vi "rio_veloster20.vi"() -> ()   [LabVIEW 2015]
uses:
  <vilib>/Analysis/Matrix/Datatypes/RealMatrix.ctl
  <vilib>/FPGAPlugInAG/cRIO-9113/niLvFpga_Open_cRIO-9113.vi
  <vilib>/rvi/interface/common/dynamic/niFpgaDynamicAddResources.vi
  <vilib>/FPGAPlugInAG/Dynamic/niLvFpga_Abort_Dynamic.vi
  <vilib>/FPGAPlugInAG/Dynamic/niLvFpga_Run_Dynamic.vi
  G_rio.vi
  <vilib>/Instr/_visa.llb/VISA Configure Serial Port (Instr).vi
  <vilib>/Utility/error.llb/Error Cluster From Error Code.vi
  <vilib>/rvi/errors/niLvFpgaAdjustHostInterfaceError.vi
  <vilib>/Analysis/Matrix/Numeric/Conversions/Array To Matrix - RA2.vi
  <vilib>/Analysis/Matrix/Numeric/Multiply/Multiply - RM,RM.vi
  <vilib>/Analysis/Matrix/Numeric/Add/Add - RM,RM.vi
  <vilib>/Analysis/baseanly.llb/Real Inverse Matrix.vi
  <vilib>/Analysis/Matrix/Numeric/Subtract/Subtract - RM,RM.vi
  <vilib>/Analysis/Matrix/Numeric/Conversions/Array To Matrix - RA.vi
  <vilib>/Analysis/Matrix/Numeric/Multiply/Multiply - R,RM.vi
  <vilib>/Analysis/Matrix/Numeric/Conversions/Matrix To Array - RM.vi
  <vilib>/rvi/interface/nirviOpenFPGA/nirviOpenFPGA.xnode
  FPGA Bitfiles/autonomous_FPGATarget2_fpga4_FZHAM7r+pqE.lvbitx
  fpga/fpga4.vi
  <vilib>/rvi/interface/nirviMethod/nirviMethod.xnode
  <vilib>/rvi/interface/nirviReadWriteControl/nirviReadWriteControl.xnode
  <vilib>/rvi/interface/Simulation/niFpgaSimulationCallBeginRW.vi
  <vilib>/rvi/errors/niLvFpgaMergeErrorWithErrorCode.vi
  NiFpgaLv.dll
  <vilib>/FPGAPlugInAG/Dynamic/niLvFpga_ReadFifo_Dynamic.vi
  <vilib>/Analysis/Matrix/NI_Matrix.lvlib
  <vilib>/Analysis/NI_AALBase.lvlib
panel:
  in  "map name":T1(ring)
  out "316H":u8[](array[numeric])
  out "FPGA":refnum<k20>
  out "Key":u8
  out "mdps torque":dbl(graph)
  out "battery voltage 2":dbl
  in  "steer limit":dbl=100.0
  in  "buzz":bool
  out "hcount":u64=1
  out "hbias":dbl
  out "vcount":u64=1
  out "vgain":dbl=1.0
  in  "heading gain":dbl=1.414
  in  "pos gain":dbl=4.0
  out "Pos_time 10":i32
  out "T PWM":u16
  out "B PWM":u16
  out "solenoid":bool
  out "brk enc":u8
  out "shift lever":dbl
  out "mobileye":u8[](array[numeric])
  out "timer":u32
  out "Mobileye_time 100":u32
  out "H_GPS":dbl
  out "pos":dbl[](array[numeric])
  out "pos error":dbl
  in  "GPS init":bool=TRUE
  in  "Gear Manual":i32(slide)=1 scale=-1.0..1.0
  out "map":i32=2
  out "P, R, D":i32
  out "heading error":dbl
  out "POS init":bool
  out "VS_CAN":dbl
  in  "brake":bool
  in  "Slide":dbl(slide)=1000.0 min=1000.0 max=2000.0 step=1500.0 scale=1000.0..2000.0
  out "novatel":refnum<visa-resource-name>
  in  "ublox":bool
  out "rest":u8[](array[numeric])
  out "GPS_novatel_time":u32
  out "GPS_time 100":u32
  out "Con_time 10":i32
  out "CAN_time 10":u32
  out "gps2":refnum<visa-resource-name>
  out "gps1":refnum<visa-resource-name>
  out "Heading":dbl
  out "ecef ref":dbl[](array[numeric])
  out "h_gps":dbl
  out "pos_gps":dbl[](array[numeric]) format="%#_19f"
  out "get heading":bool
  out "get position":bool
  out "dt":dbl
  out "rt":dbl
  out "CAN Comm Enabled":bool
  in  "SPAS Enable":bool=TRUE
  out "Ref steer":dbl=1.0
  in  "Steer input":bool=TRUE
  in  "Ref steer manual":dbl(knob) scale=-550.0..550.0
  out "Ref vel":dbl=1.0
  in  "Ref vel manual":dbl
  in  "Velocity input":bool
  out "Auto":bool
  out "Run":bool
  out "E - STOP":bool
  out "Throttle Enable":bool=TRUE
  # "P"
  # "R"
  # "D"
  # "Ref steer manual"
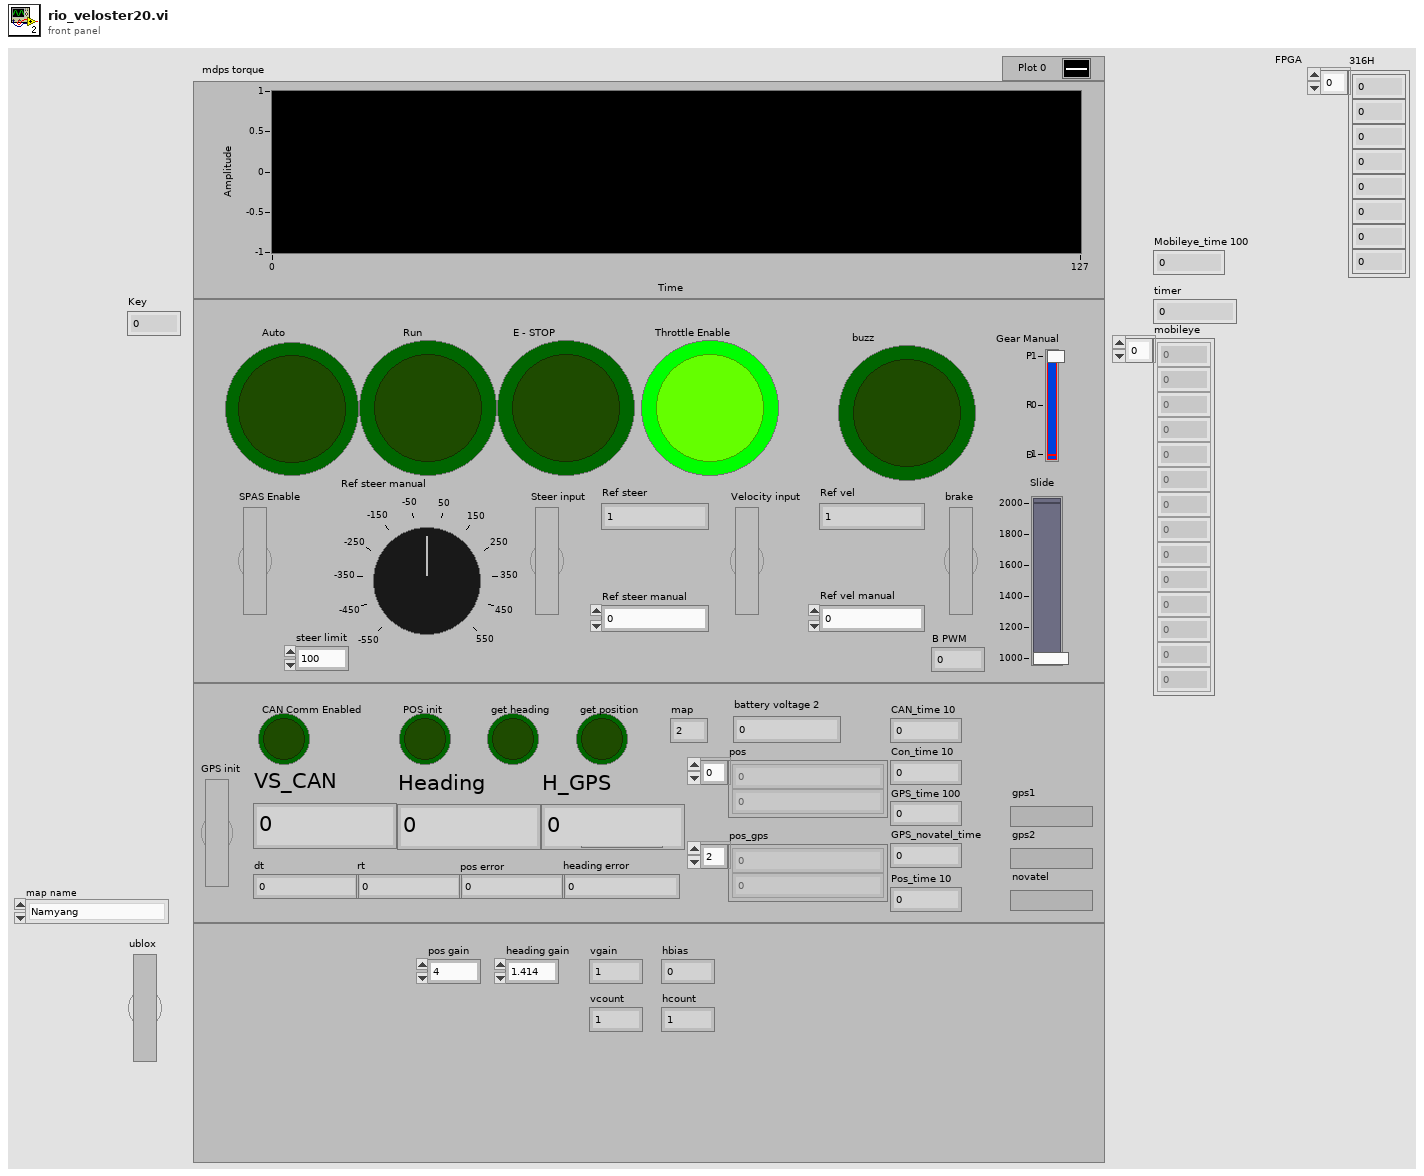
[diagram p1: front panel]
types:
  T1 = enum32{"Namyang", "Hyundai", "KAIST", "Ajou", "Munji", "Airforce", "Car", "KATRI", "Samsung", "Coex", "Gwangnaru", "Inje", "sinjin"}
  T2 = cluster{"timestamp high":u32, "timestamp low":u32, "identifier":u32, "type":enum8{"Data Frame", "Remote Frame", "(reserved)", "(reserved) ", "(reserved)  ", "(reserved)   ", "Bus Error", "Transceiver Fault"}, "info A":u8, "info B":u8, "data length":u8, "data":u8[]}
  T3 = cluster{"connection ID":refnum<k16>, "net address":u32, "port":u16}
  T4 = cluster{"hash":i64, "sys time":i64, "mobileye":u8[]}
  T5 = cluster{"hash":i64, "sys time":i64, "n":i32, "error":i32[]}
  T6 = cluster{"hash":i64, "sys time":i64, "time":dbl, "yaw_rate":dbl, "mdps torque":dbl, "mdps str_ang":dbl, "VS_CAN":dbl, "lat_accel":dbl, "mcp":dbl, "accel pedal value":dbl, "tps":dbl, "odometer":dbl, "battery voltage":dbl, "WHL_SPD_RR":dbl, "WHL_SPD_RL":dbl, "WHL_SPD_FR":dbl, "WHL_SPD_FL":dbl}
  T7 = cluster{"hash":i64, "sys time":i64, "ref_vel":dbl, "ref_steer":dbl, "alert":u8}
  T8 = cluster{"hash":i64, "sys time":i64, "ref_vel":dbl, "ref_steer":dbl}
  T9 = cluster{"hash":i64, "sys time":i64, "Auto":bool, "Run":bool, "Solenoid":bool, "T lim":bool, "brk_enc":u8, "B PWM":u16, "T PWM":u16, "ref_vel":dbl, "ref_bkr_enc":dbl, "ref_apv":dbl, "ref_steer":dbl}
  T10 = typedef "NI_Matrix.lvlib/RealMatrix.ctl" = dbl[][]
  T11 = cluster{"hash":i64, "sys time":i64, "time":dbl, "x":dbl, "y":dbl, "h":dbl, "numSV":i32, "postype":i32, "lag":i32, "hordev":dbl, "lat":dbl, "lon":dbl, "hgt":dbl, "map_idx":i32}
  T12 = cluster{"LCC[0]":dbl, "LCC[1]":dbl, "LCC[2]":dbl, "LCC[3]":dbl, "LCC[4]":dbl, "LCC[5]":dbl, "LCC[6]":dbl, "LCC[7]":dbl, "LCC[8]":dbl, "LCC[9]":dbl, "LCC[10]":dbl, "LCC[11]":dbl, "LCC[12]":dbl, "LCC[13]":dbl, "LCC[14]":dbl}
  T13 = cluster{"hash":i64, "sys time":i64, "time":dbl, "speed":dbl, "heading":dbl, "lat":dbl, "lon":dbl}
  T14 = cluster{"vel[0]":dbl, "vel[1]":dbl, "vel[2]":dbl, "vel[3]":dbl, "vel[4]":dbl, "vel[5]":dbl, "vel[6]":dbl}
  T15 = cluster{"output[0]":dbl, "output[1]":dbl, "output[2]":dbl, "output[3]":dbl, "output[4]":dbl, "output[5]":dbl, "output[6]":dbl, "output[7]":dbl, "output[8]":dbl, "output[9]":dbl, "output[10]":dbl, "output[11]":dbl, "output[12]":dbl, "output[13]":dbl, "output[14]":dbl}
  T16 = cluster{"output[0]":dbl, "output[1]":dbl, "output[2]":dbl, "output[3]":dbl, "output[4]":dbl, "output[5]":dbl, "output[6]":dbl}
  T17 = cluster{"hash":i64, "sys time":i64, "dt":dbl, "x":dbl, "y":dbl, "speed":dbl, "heading":dbl, "yaw_rate":dbl}
  T18 = cluster{"Real 2D Array[0]":dbl, "Real 2D Array[1]":dbl, "Real 2D Array[2]":dbl, "Real 2D Array[3]":dbl, "Real 2D Array[4]":dbl}
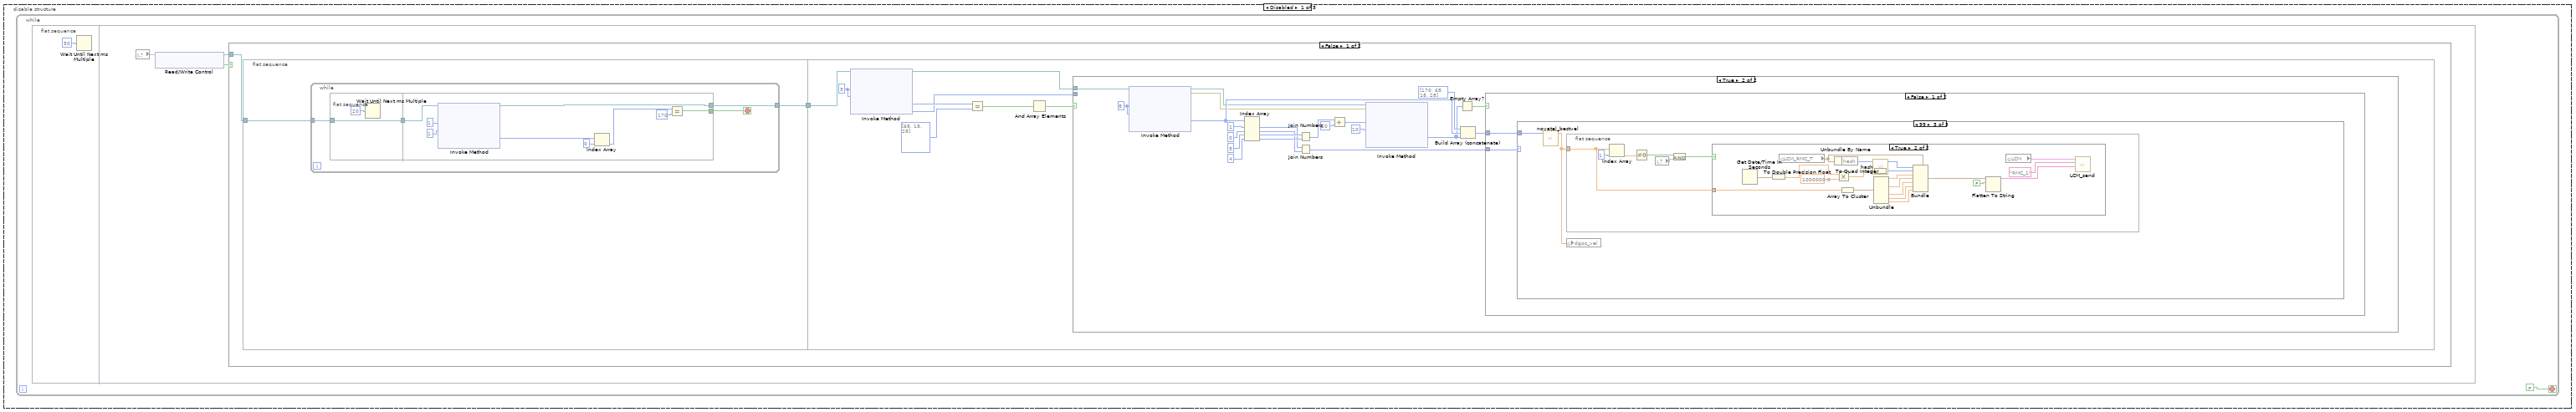
[diagram p2: hidden frame]
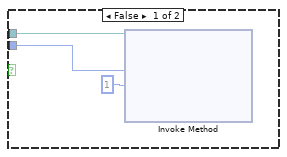
[diagram p3: hidden frame]
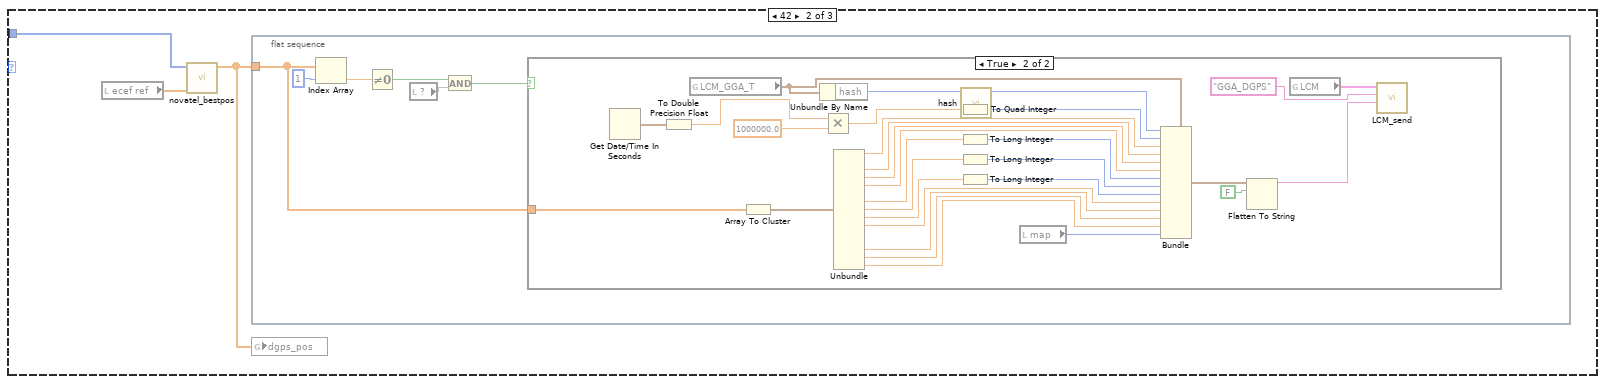
[diagram p5: hidden frame]
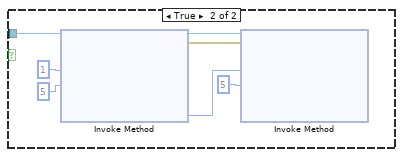
[diagram p9: hidden frame]
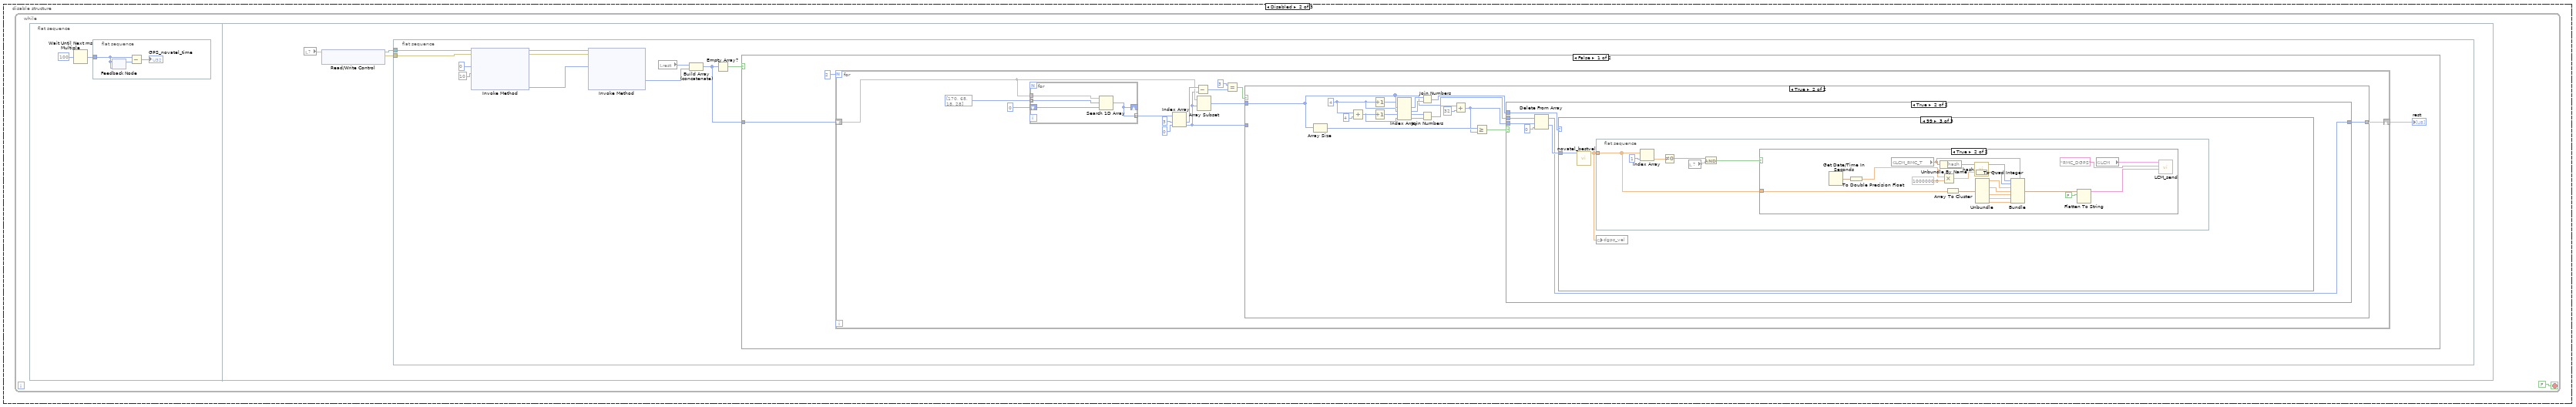
[diagram p10: hidden frame]
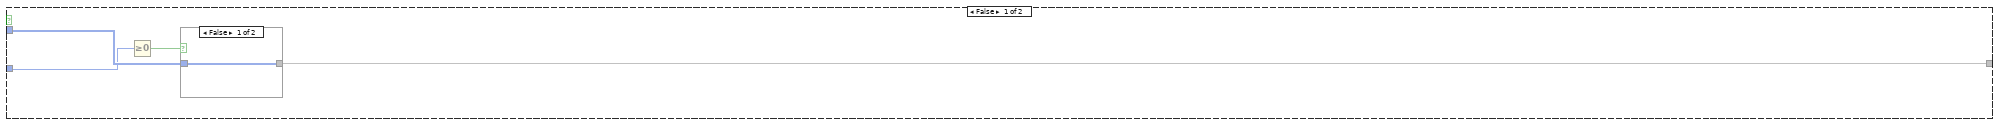
[diagram p11: hidden frame]
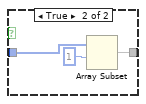
[diagram p12: hidden frame]
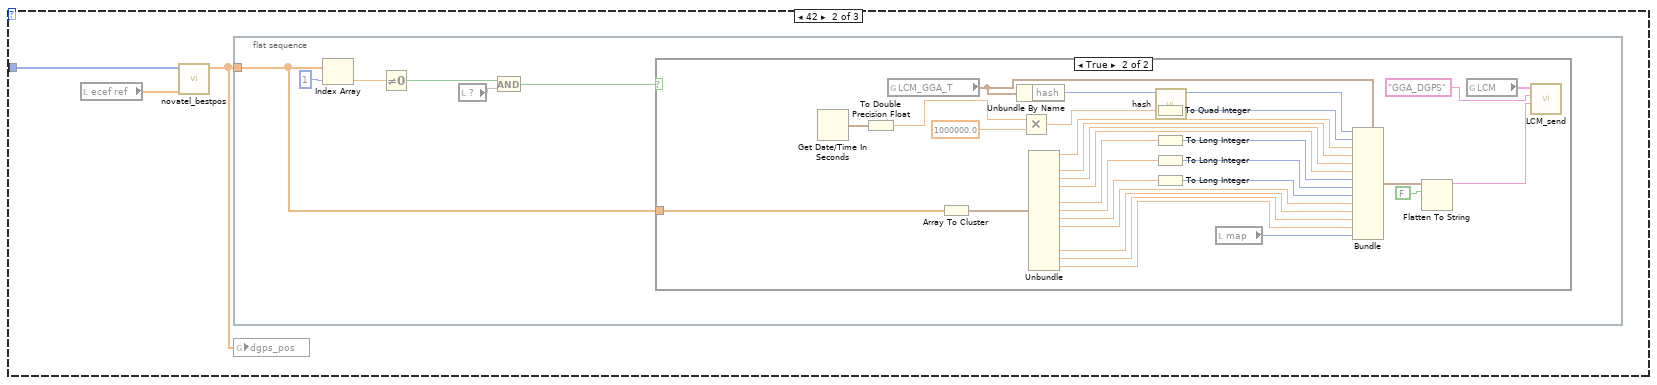
[diagram p15: hidden frame]
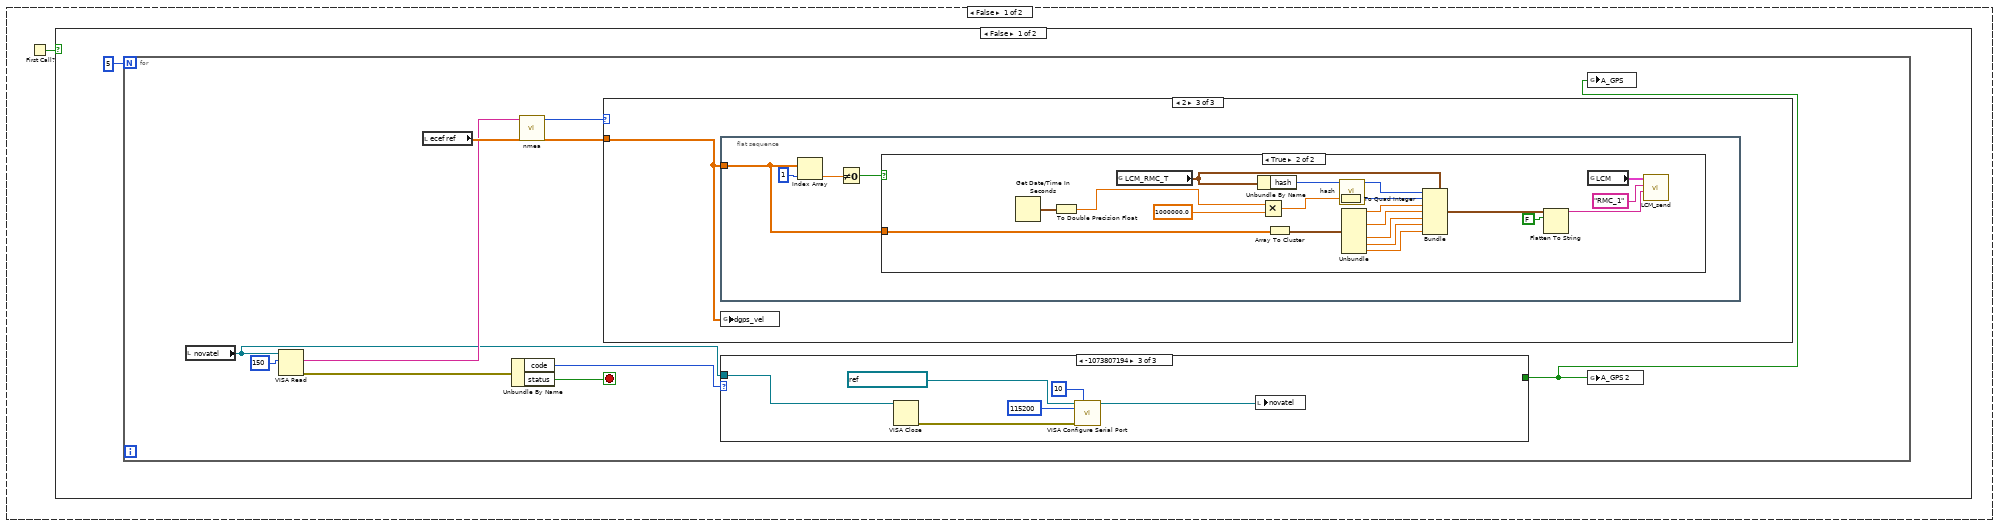
[diagram p19: hidden frame]
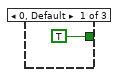
[diagram p20: hidden frame]
diagram:
  n1 = flat-sequence {
    frame #0 {
      w3 = u16 7668 ("port")
      w9 = u16 7667 ("port")
      n2 = xnode "Open FPGA VI Reference"() -> ("FPGA VI Reference Out"=w18:refnum<k20>, "error out"=w17:errorcluster)  [unwired: 2 in]
      n3 = global read "G_rio.vi" "LCM PC"() -> (w7:T3)
      n4 = Decrement(x=w9) -> (x-1=w8:u16)
      n5 = UDP Open(11:w3) -> (port=w5:refnum<k16>)  [unwired: 4 in, 2 out]
      n6 = xnode "Invoke Method"("FPGA VI Reference In"=w18, "error in"=w17) -> ("FPGA VI Reference Out"=w16:refnum<k20>, "error out"=w15:errorcluster)
      n7 = Bundle By Name(cluster=w7, "port"=w3, "connection ID"=w5, "net address"=u32 0) -> (w6:T3)
      n8 = UDP Open(11:w8) -> (port=w11:refnum<k16>)  [unwired: 4 in, 2 out]
      n9 = xnode "Invoke Method"("FPGA VI Reference In"=w16, "error in"=w15, "Wait Until Done (F)"=FALSE) -> ("FPGA VI Reference Out"=→"FPGA":refnum<k20>)  [unwired: 1 out]
      n10 = global read "G_rio.vi" "LCM"() -> (w13:T3)
      n11 = global write "G_rio.vi" "LCM PC"(w6) -> ()
      n12 = Bundle By Name(cluster=w13, "port"=w9, "connection ID"=w11, "net address"=u32 4294967295) -> (w12:T3)
      n13 = global write "G_rio.vi" "LCM"(w12) -> ()
    }
    frame #1 {
      n14 = flat-sequence {
        frame #0 {
          w59 = FALSE ("Auto")
          n15 = global write "G_rio.vi" "brake release"(FALSE ("brake release")) -> ()
          n16 = global write "G_rio.vi" "Auto"(w59) -> ()
          n17 = global write "G_rio.vi" "Auto SW"(w59) -> ()
        }
        frame #1 {
          w62 = FALSE ("GPS init")
          w63 = 0.0 ("Ref_vel_planner")
          n18 = global write "G_rio.vi" "T lim counter 2"(u16 300 ("T lim counter 2")) -> ()
          n19 = local write "Slide"(1500.0 ("Slide")) -> ()
          n20 = global write "G_rio.vi" "Ref_steer_planner"(w63) -> ()
          n21 = global write "G_rio.vi" "Ref_vel_planner"(w63) -> ()
          n22 = local write "rest"(u8[] [] ("rest")) -> ()
          n23 = local write "brake"(w62) -> ()
          n24 = local write "rest"(u8[] [] ("rest")) -> ()
          n25 = local write "Velocity input"(w62) -> ()
          n26 = local write "GPS init"(w62) -> ()
          "POS init" <- TRUE ("pos linit")
        }
      }
      n27 = disable-structure shown="Enabled" {
        frame Enabled {
          w22 = refnum<visa-resource-name> "ASRL1::INSTR" ("VISA resource name")
          w20 = refnum<visa-resource-name> "USB0::0x1546::0x01A6::NI-VISA-0::1::RAW" ("VISA resource name")
          w21 = refnum<visa-resource-name> "USB0::0x1546::0x01A6::NI-VISA-1::1::RAW" ("VISA resource name")
          n28 = call-poly "VISA Configure Serial Port"("VISA resource name"=w22, "timeout (10sec)"=u32 10, "baud rate (9600)"=u32 115200) -> ("VISA resource name out"=w24:refnum<visa-resource-name>, "error out"=w19:errorcluster)  [unwired: 11 in]
          n29 = case shown="Error" w19 {
            tunnel: [w37 w41] -> w23
            tunnel: w24 -> [w37 w40]
            tunnel: w22 -> [_ w38]
            frame No Error {
            }
            frame Error {
              n30 = VISA Close(VISA resource name=w40) -> (error out=w39:errorcluster)  [unwired: 1 in]
              n31 = call-poly "VISA Configure Serial Port"("VISA resource name"=w38, "timeout (10sec)"=u32 10, "baud rate (9600)"=u32 115200, "error in (no error)"=w39) -> ("VISA resource name out"=w41:refnum<visa-resource-name>)  [unwired: 10 in, 1 out]
            }
          }
          "novatel" <- w23
          n32 = call-poly "VISA Configure Serial Port"("VISA resource name"=w20, "timeout (10sec)"=u32 1, "baud rate (9600)"=u32 115200) -> ("VISA resource name out"=w27:refnum<visa-resource-name>, "error out"=w29:errorcluster)  [unwired: 11 in]
          n33 = call-poly "VISA Configure Serial Port"("VISA resource name"=w21, "timeout (10sec)"=u32 1, "baud rate (9600)"=u32 115200) -> ("VISA resource name out"=w25:refnum<visa-resource-name>, "error out"=w30:errorcluster)  [unwired: 11 in]
          n34 = case shown="Error" w29 {
            tunnel: [w44 w48] -> w28
            tunnel: w27 -> [w44 w47]
            tunnel: w20 -> [_ w45]
            frame No Error {
            }
            frame Error {
              n35 = VISA Close(VISA resource name=w47) -> (error out=w46:errorcluster)  [unwired: 1 in]
              n36 = call-poly "VISA Configure Serial Port"("VISA resource name"=w45, "timeout (10sec)"=u32 1, "baud rate (9600)"=u32 115200, "error in (no error)"=w46) -> ("VISA resource name out"=w48:refnum<visa-resource-name>)  [unwired: 10 in, 1 out]
            }
          }
          "gps2" <- w28
          n37 = case shown="Error" w30 {
            tunnel: [w51 w55] -> w26
            tunnel: w25 -> [w51 w54]
            tunnel: w21 -> [_ w52]
            frame No Error {
            }
            frame Error {
              n38 = VISA Close(VISA resource name=w54) -> (error out=w53:errorcluster)  [unwired: 1 in]
              n39 = call-poly "VISA Configure Serial Port"("VISA resource name"=w52, "timeout (10sec)"=u32 1, "baud rate (9600)"=u32 115200, "error in (no error)"=w53) -> ("VISA resource name out"=w55:refnum<visa-resource-name>)  [unwired: 10 in, 1 out]
            }
          }
          "gps1" <- w26
        }
        frame Disabled {
        }
      }
    }
    frame #2 {
      (unwired) FALSE
      n40 = disable-structure shown="Enabled" {
        frame Enabled {
          n41 = while {
            stop <- FALSE stop-if-true
            n42 = flat-sequence {
              frame #0 {
                n43 = Wait Until Next ms Multiple(millisecond multiple=u32 100) -> (millisecond timer value=w104:u32)
                n44 = flat-sequence {
                  tunnel: w104 -> [w106]
                  frame #0 {
                    n45 = feedback #1(w106) -> (w107:u32)
                    n46 = feedback-in #1(w106) -> ()
                    n47 = Subtract(x=w106, y=w107) -> (x-y=→"Mobileye_time 100":u32)
                  }
                }
              }
              frame #1 {
                n48 = local read "FPGA"() -> (w155:refnum<k20>)
                n49 = xnode "Read/Write Control"("FPGA VI Reference In"=w155) -> ("m 700"=w115:u8[], "m 760"=w151:u8[], "m 710"=w140:u8[], "m 711"=w136:u8[], "m 720"=w134:u8[], "m 721"=w133:u8[], "m 722"=w132:u8[], "m 723"=w131:u8[], "m 724"=w130:u8[], "m 725"=w129:u8[], "m 726"=w128:u8[], "m 727"=w127:u8[], "m 728"=w126:u8[], "m 729"=w125:u8[])  [unwired: 1 in, 2 out]
                n50 = Build Array(w134, w133, w132, w131, w130, w129, w128, w127, w126, w125) -> (w124:u8[][])
                n51 = Array Subset(array=w115, index=0, length=4) -> (w112:u8[])
                n52 = Array Subset(array=w136, index=6, length=6) -> (w135:u8[])
                n53 = Index Array(array=w115, index #1=4 ("index"), index #4=8 ("index"), index #5=11 ("index")) -> (element #1=w148:u8, element #2=w147:u8, element #3=w146:u8, element #4=w145:u8, element #5=w144:u8)  [unwired: 2 in]
                n54 = Index Array(array=w112, index #1=0 ("index")) -> (element #1=w121:u8, element #2=w120:u8, element #3=w119:u8, element #4=w118:u8)  [unwired: 3 in]
                n55 = Array Subset(array=w151, index=4, length=3) -> (w143:u8[])
                n56 = Array Subset(array=w140, index=5, length=7) -> (w139:u8[])
                n57 = Join Numbers(hi=w121, lo=w120) -> ((hi.lo)=w117:u16)
                n58 = Join Numbers(hi=w119, lo=w118) -> ((hi.lo)=w116:u16)
                n59 = Build Array (concatenate)(w112, w148, w147, w146, w145, w144, w143, w139, w135) -> (w123:u8[])
                n60 = for {
                  tunnel: w124 -> [w157] mode=indexing
                  shift-right: [w160] -> w111
                  shift-left: w123 -> [w161]
                  n61 = Array Subset(array=w157, index=4, length=8) -> (w156:u8[])
                  n62 = disable-structure shown="Enabled" {
                    disable-tunnel: [w164 TRUE ("lsb carry out")] -> w162
                    disable-tunnel: w156 -> [w163 _]
                    frame Disabled {
                      n63 = Index Array(array=w163, index=0) -> (element=w166:u8)
                      n64 = Rotate Right With Carry(2:w166, 3:FALSE ("carry")) -> (1:w164:bool)  [unwired: 1 out]
                    }
                    frame Enabled {
                    }
                  }
                  n65 = case shown="True" w162 {
                    tunnel: w161 -> [w169 w172]
                    tunnel: [w169 w171] -> w160
                    tunnel: w156 -> [_ w170]
                    frame False {
                    }
                    frame True {
                      n66 = Build Array (concatenate)(w172, w170) -> (w171:u8[])
                    }
                  }
                }
                "mobileye" <- w111
                n67 = Join Numbers(hi=w117, lo=w116) -> ((hi.lo)=w109:u32)
                "timer" <- w109
                n68 = feedback-in #2(w109) -> ()
                n69 = feedback #2(w109) -> (w110:u32)
                n70 = Not Equal?(x=w109, y=w110) -> (x != y?=w108:bool)
                n71 = global write "G_rio.vi" "A_camera"(w108) -> ()
              }
              frame #2 {
                n72 = Get Date/Time In Seconds() -> (seconds since 1Jan1904=w177:timestamp)
                n73 = global read "G_rio.vi" "LCM_EYE_RAW_T"() -> (w186:T4)
                n74 = To Double Precision Float(number=w177) -> (double precision float=w176:dbl)
                n75 = Unbundle By Name(w186) -> ("hash"=w185:i64)
                n76 = Multiply(x=w176, y=1000000.0) -> (x*y=w174:dbl)
                n77 = local read "mobileye"() -> (w178:u8[])
                n78 = call "hash.vi"("input"=w185) -> ("output"=w184:i64)  [unwired: 10 in]
                n79 = To Quad Integer(1:w174) -> (0:w173:i64)
                n80 = Bundle By Name(cluster=w186, "hash"=w184, "sys time"=w173, "mobileye"=w178) -> (w183:T4)
                n81 = Flatten To String(anything=w183, prepend array or string size? (T)=FALSE) -> (data string=w181:string)  [unwired: 2 in, 2 out]
                n82 = global read "G_rio.vi" "LCM"() -> (w182:T3)
                n83 = call "LCM_send.vi"("DATA"=w181, "ID"="EYE_RAW_T", "LCM"=w182) -> ()  [unwired: 7 in, 2 out]
              }
            }
          }
        }
        frame Disabled {
        }
      }
      n84 = while {
        stop <- FALSE stop-if-true
        n85 = flat-sequence {
          frame #0 {
            n86 = global read "G_rio.vi" "PWM Brake"() -> (w68:dbl)
            n87 = global read "G_rio.vi" "PWM Brake"() -> (w84:dbl)
            n88 = Wait Until Next ms Multiple(millisecond multiple=u32 33 ("millisecond timer value")) -> ()  [unwired: 1 out]
            n89 = global read "G_rio.vi" "accel pedal value"() -> (w72:dbl)
            n90 = global read "G_rio.vi" "brake_act_can"() -> (w74:bool)
            n91 = global read "G_rio.vi" "Ref APS"() -> (w73:dbl)
            n92 = local read "Ref vel"() -> (w85:dbl)
            n93 = Greater?(x=w68, y=1000.0) -> (0:w76:bool)
            n94 = Greater?(x=w84, y=1000.0) -> (0:w81:bool)
            n95 = Not Equal To 0?(x=w73) -> (x != 0?=w71:bool)
            n96 = Equal To 0?(x=w72) -> (x = 0?=w70:bool)
            n97 = Not(x=w74) -> (.not. x?=w75:bool)
            n98 = Not Equal To 0?(x=w85) -> (x != 0?=w82:bool)
            n99 = Or(x=w82, y=w81) -> (x .or. y?=w80:bool)
            n100 = And(x=w71, y=w70) -> (x .and. y?=w77:bool)
            n101 = And(x=w76, y=w75) -> (x .and. y?=w78:bool)
            n102 = Not Or(1:w78, 2:w77) -> (0:w79:bool)
            n103 = global write "G_rio.vi" "Speed Cont"(w80) -> ()
            n104 = global write "G_rio.vi" "A_control"(w79) -> ()
          }
          frame #1 {
            n105 = disable-structure shown="Enabled" {
              frame Enabled {
                n106 = call "alertvisual.vi"() -> ()  [unwired: 12 in]
              }
              frame Disabled {
              }
            }
          }
          frame #2 {
            n107 = Get Date/Time In Seconds() -> (seconds since 1Jan1904=w93:timestamp)
            n108 = To Double Precision Float(number=w93) -> (double precision float=w92:dbl)
            n109 = global read "G_rio.vi" "LCM_ERROR_T"() -> (w101:T5)
            n110 = global read "G_rio.vi" "error count"() -> (w87:i32[])
            n111 = Unbundle By Name(w101) -> ("hash"=w100:i64)
            n112 = Multiply(x=w92, y=1000000.0) -> (x*y=w90:dbl)
            n113 = Array Size(array=w87) -> (size(s)=w88:i32)
            n114 = call "hash.vi"("input"=w100) -> ("output"=w99:i64)  [unwired: 10 in]
            n115 = To Quad Integer(1:w90) -> (0:w89:i64)
            n116 = Bundle By Name(cluster=w101, "hash"=w99, "sys time"=w89, "n"=w88, "error"=w87) -> (w98:T5)
            n117 = Flatten To String(anything=w98, prepend array or string size? (T)=FALSE) -> (data string=w96:string)  [unwired: 2 in, 2 out]
            n118 = global read "G_rio.vi" "LCM"() -> (w97:T3)
            n119 = call "LCM_send.vi"("DATA"=w96, "ID"="ERROR_T", "LCM"=w97) -> ()  [unwired: 7 in, 2 out]
          }
        }
      }
      n120 = while {
        stop <- FALSE stop-if-true
        n121 = flat-sequence {
          frame #0 {
            n122 = Wait Until Next ms Multiple(millisecond multiple=u32 10) -> (millisecond timer value=w658:u32)
            n123 = flat-sequence {
              tunnel: w658 -> [w661]
              frame #0 {
                n124 = feedback #3(w661) -> (w662:u32)
                n125 = feedback-in #3(w661) -> ()
                n126 = Subtract(x=w661, y=w662) -> (x-y=→"CAN_time 10":u32)
              }
            }
          }
          frame #1 {
            n127 = disable-structure shown="Enabled" {
              disable-tunnel: [w665 _] -> w663
              frame Enabled {
                n128 = local read "FPGA"() -> (w664:refnum<k20>)
                n129 = for {
                  tunnel: u32[] [356, 544, 790, 809, 914, 1087, 1200, 1264, 1349, 1680] -> [w670] mode=indexing
                  tunnel: [w669] -> w666 mode=indexing
                  tunnel: w664 -> [w668]
                  n130 = case shown="4B0" w670 {
                    tunnel: [_ w672 w752 w784 w824 w884 w909 w976 w1009 w1038] -> w669
                    tunnel: w668 -> [_ w671 w751 w783 w823 w883 w908 w975 w1008 w1037]
                    frame 0, Default {
                    }
                    frame 544 {
                      n131 = flat-sequence {
                        tunnel: [w677] -> w672
                        tunnel: [w676] -> w673
                        tunnel: w671 -> [w674]
                        frame #0 {
                          n132 = xnode "Read/Write Control"("FPGA VI Reference In"=w674) -> ("can 220"=w681:u8[])  [unwired: 1 in, 2 out]
                          n133 = Index Array(array=w681, index #1=0 ("index")) -> (element #1=w687:u8, element #2=w686:u8, element #3=w685:u8, element #4=w684:u8)  [unwired: 3 in]
                          n134 = Join Numbers(hi=w687, lo=w686) -> ((hi.lo)=w683:u16)
                          n135 = Join Numbers(hi=w685, lo=w684) -> ((hi.lo)=w682:u16)
                          n136 = Join Numbers(hi=w683, lo=w682) -> ((hi.lo)=w675:u32)
                          n137 = disable-structure shown="Disabled" {
                            disable-tunnel: w675 -> [w689 _]
                            frame Disabled {
                              n138 = global write "G_rio.vi" "time"(w689) -> ()
                            }
                            frame Enabled {
                            }
                          }
                          n139 = feedback #4(u32 0) -> (w678:u32)
                          n140 = feedback-in #4(w675) -> ()
                          n141 = Not Equal?(x=w675, y=w678) -> (x != y?=w677:bool)
                          n142 = Array Subset(array=w681, index=4) -> (w676:u8[])  [unwired: 1 in]
                        }
                      }
                      n143 = case shown="True" w672 {
                        tunnel: w673 -> [_ w723]
                        frame False {
                        }
                        frame True {
                          w693 = u16 8191
                          w700 = u16 2047
                          n144 = Index Array(array=w723, index #1=5 ("index"), index #2=4 ("index"), index #3=1 ("index"), index #4=0 ("index"), index #5=7 ("index"), index #6=6 ("index")) -> (element #1=w716:u8, element #2=w715:u8, element #3=w714:u8, element #4=w713:u8, element #5=w712:u8, element #6=w711:u8)
                          n145 = Join Numbers(hi=w714, lo=w713) -> ((hi.lo)=w701:u16)
                          n146 = Join Numbers(hi=w712, lo=w711) -> ((hi.lo)=w692:u16)
                          n147 = And(x=w716, y=u8 15) -> (x .and. y?=w709:u8)
                          n148 = Logical Shift(y=i16 -6, x=w714) -> (x << y=w703:u8)
                          n149 = Logical Shift(y=i16 -6, x=w712) -> (x << y=w696:u8)
                          n150 = Equal To 0?(x=w703) -> (x = 0?=w704:bool)
                          n151 = Join Numbers(hi=w709, lo=w715) -> ((hi.lo)=w706:u16)
                          n152 = And(x=w700, y=w701) -> (x .and. y?=w699:u16)
                          n153 = And(x=w693, y=w692) -> (x .and. y?=w691:u16)
                          n154 = Not Equal?(x=w700, y=w699) -> (x != y?=w705:bool)
                          n155 = Not Equal?(x=w693, y=w691) -> (x != y?=w694:bool)
                          n156 = Equal To 0?(x=w696) -> (x = 0?=w695:bool)
                          n157 = Not Equal?(x=u16 4095, y=w706) -> (x != y?=w707:bool)
                          n158 = case shown="True" w707 {
                            tunnel: w706 -> [_ w750]
                            frame False {
                            }
                            frame True {
                              n159 = global write "G_rio.vi" "mcp"(w750) -> ()
                              n160 = Greater?(x=w750, y=u16 10) -> (0:w749:bool)
                              n161 = global write "G_rio.vi" "brake_act_can"(w749) -> ()
                            }
                          }
                          n162 = And(x=w704, y=w705) -> (x .and. y?=w698:bool)
                          n163 = And(x=w695, y=w694) -> (x .and. y?=w690:bool)
                          n164 = case shown="True" w698 {
                            tunnel: w699 -> [_ w747]
                            frame False {
                            }
                            frame True {
                              n165 = To Double Precision Float(number=w747) -> (double precision float=w746:dbl)
                              n166 = Multiply(x=w746, y=0.01) -> (x*y=w744:dbl)
                              n167 = Subtract(x=w744, y=10.23) -> (x-y=w742:dbl)
                              n168 = global write "G_rio.vi" "lat_accel"(w742) -> ()
                            }
                          }
                          n169 = case shown="True" w690 {
                            tunnel: w691 -> [_ w730]
                            frame False {
                            }
                            frame True {
                              n170 = To Double Precision Float(number=w730) -> (double precision float=w729:dbl)
                              n171 = Multiply(x=w729, y=0.01) -> (x*y=w727:dbl)
                              n172 = Subtract(x=w727, y=40.95) -> (x-y=w724:dbl)
                              n173 = disable-structure shown="Enabled" {
                                disable-tunnel: [w734 w739] -> w725
                                disable-tunnel: w724 -> [w732 w740]
                                frame Disabled {
                                n174 = Add(x=w732, y=-0.034) -> (x+y=w731:dbl)
                                n175 = Multiply(x=w731, y=1.045) -> (x*y=w735:dbl)
                                n176 = Add(x=w735, y=0.0) -> (x+y=w734:dbl)
                                }
                                frame Enabled {
                                n177 = Multiply(x=w740, y=1.007006684581104) -> (x*y=w739:dbl)
                                }
                              }
                              n178 = disable-structure shown="Enabled" {
                                disable-tunnel: w725 -> [w741 _]
                                frame Enabled {
                                n179 = global write "G_rio.vi" "yaw_rate"(w741) -> ()
                                }
                                frame Disabled {
                                }
                              }
                            }
                          }
                        }
                      }
                    }
                    frame 790 {
                      n180 = flat-sequence {
                        tunnel: [w757] -> w752
                        tunnel: [w756] -> w753
                        tunnel: w751 -> [w754]
                        frame #0 {
                          n181 = xnode "Read/Write Control"("FPGA VI Reference In"=w754) -> ("can 316"=w761:u8[])  [unwired: 1 in, 2 out]
                          n182 = Index Array(array=w761, index #1=0 ("index")) -> (element #1=w767:u8, element #2=w766:u8, element #3=w765:u8, element #4=w764:u8)  [unwired: 3 in]
                          n183 = Join Numbers(hi=w767, lo=w766) -> ((hi.lo)=w763:u16)
                          n184 = Join Numbers(hi=w765, lo=w764) -> ((hi.lo)=w762:u16)
                          n185 = Join Numbers(hi=w763, lo=w762) -> ((hi.lo)=w755:u32)
                          n186 = Array Subset(array=w761, index=4) -> (w756:u8[])  [unwired: 1 in]
                          n187 = feedback #5(u32 0) -> (w758:u32)
                          n188 = feedback-in #5(w755) -> ()
                          n189 = Not Equal?(x=w755, y=w758) -> (x != y?=w757:bool)
                        }
                      }
                      n190 = case shown="True" w752 {
                        tunnel: w753 -> [_ w781]
                        frame False {
                        }
                        frame True {
                          w772 = u8 1 ("x")
                          n191 = Index Array(array=w781, index #1=0 ("index"), index #2=3 ("index"), index #3=2 ("index")) -> (element #1=w775:u8, element #2=w778:u8, element #3=w777:u8)
                          n192 = Join Numbers(hi=w778, lo=w777) -> ((hi.lo)=w774:u16)
                          n193 = And(x=w772, y=w775) -> (x .and. y?=w773:u8)
                          n194 = Equal?(x=w772, y=w773) -> (x = y?=w771:bool)
                          n195 = Not Equal To 0?(x=w774) -> (x != 0?=w770:bool)
                          n196 = And(x=w771, y=w770) -> (x .and. y?=w769:bool)
                          n197 = case shown="False" w769 {
                            frame False {
                              n198 = global write "G_rio.vi" "Auto SW"(FALSE ("Auto SW")) -> ()
                            }
                            frame True {
                            }
                          }
                          "316H" <- w781
                        }
                      }
                    }
                    frame 809 {
                      n199 = flat-sequence {
                        tunnel: [w788] -> w784
                        tunnel: [w787] -> w785
                        tunnel: w783 -> [w786]
                        frame #0 {
                          n200 = xnode "Read/Write Control"("FPGA VI Reference In"=w786) -> ("can 329"=w793:u8[])  [unwired: 1 in, 2 out]
                          n201 = Index Array(array=w793, index #1=0 ("index")) -> (element #1=w799:u8, element #2=w798:u8, element #3=w797:u8, element #4=w796:u8)  [unwired: 3 in]
                          n202 = Join Numbers(hi=w799, lo=w798) -> ((hi.lo)=w795:u16)
                          n203 = Join Numbers(hi=w797, lo=w796) -> ((hi.lo)=w794:u16)
                          n204 = Join Numbers(hi=w795, lo=w794) -> ((hi.lo)=w789:u32)
                          n205 = Array Subset(array=w793, index=4) -> (w787:u8[])  [unwired: 1 in]
                          n206 = feedback #6(u32 0) -> (w790:u32)
                          n207 = feedback-in #6(w789) -> ()
                          n208 = Not Equal?(x=w789, y=w790) -> (x != y?=w788:bool)
                        }
                      }
                      n209 = case shown="True" w784 {
                        tunnel: w785 -> [_ w810]
                        frame False {
                        }
                        frame True {
                          # "10ms"
                          n210 = Index Array(array=w810, index #1=5 ("index"), index #2=6 ("index"), index #3=4 ("index")) -> (element #1=w807:u8, element #2=w804:u8)  [unwired: 1 out]
                          n211 = Not Equal?(x=w807, y=u8 255 ("x")) -> (x != y?=w803:bool)
                          n212 = Not Equal?(x=w804, y=u8 255 ("x")) -> (x != y?=w802:bool)
                          n213 = case shown="True" w803 {
                            tunnel: w807 -> [_ w822]
                            frame False {
                            }
                            frame True {
                              n214 = Subtract(x=w822, y=u8 32) -> (x-y=w820:u8)
                              n215 = To Double Precision Float(number=w820) -> (double precision float=w819:dbl)
                              n216 = Multiply(x=w819, y=100.0) -> (x*y=w817:dbl)
                              n217 = Divide(x=w817, y=213.0) -> (x/y=w815:dbl)
                              n218 = global write "G_rio.vi" "tps"(w815) -> ()
                            }
                          }
                          n219 = case shown="True" w802 {
                            tunnel: w804 -> [_ w814]
                            frame False {
                            }
                            frame True {
                              n220 = To Double Precision Float(number=w814) -> (double precision float=w813:dbl)
                              n221 = Multiply(x=w813, y=0.3906) -> (x*y=w812:dbl)
                              n222 = global write "G_rio.vi" "accel pedal value"(w812) -> ()
                            }
                          }
                        }
                      }
                    }
                    frame 914 {
                      n223 = flat-sequence {
                        tunnel: [w828] -> w824
                        tunnel: [w827] -> w825
                        tunnel: w823 -> [w826]
                        frame #0 {
                          n224 = xnode "Read/Write Control"("FPGA VI Reference In"=w826) -> ("can 392"=w833:u8[])  [unwired: 1 in, 2 out]
                          n225 = Index Array(array=w833, index #1=0 ("index")) -> (element #1=w839:u8, element #2=w838:u8, element #3=w837:u8, element #4=w836:u8)  [unwired: 3 in]
                          n226 = Join Numbers(hi=w839, lo=w838) -> ((hi.lo)=w835:u16)
                          n227 = Join Numbers(hi=w837, lo=w836) -> ((hi.lo)=w834:u16)
                          n228 = Join Numbers(hi=w835, lo=w834) -> ((hi.lo)=w829:u32)
                          n229 = Array Subset(array=w833, index=4) -> (w827:u8[])  [unwired: 1 in]
                          n230 = feedback #7(u32 0) -> (w830:u32)
                          n231 = feedback-in #7(w829) -> ()
                          n232 = Not Equal?(x=w829, y=w830) -> (x != y?=w828:bool)
                        }
                      }
                      n233 = case shown="True" w824 {
                        tunnel: w825 -> [_ w847]
                        frame False {
                        }
                        frame True {
                          # "20ms"
                          n234 = Array Subset(array=w847, index=0, length=7) -> (w844:u8[])
                          n235 = Index Array(array=w847, index #1=7 ("index"), index #2=2 ("index"), index #3=1 ("index"), index #4=4 ("index"), index #5=3 ("index")) -> (element #1=w841:u8, element #2=w853:u8, element #3=w852:u8, element #4=w849:u8, element #5=w848:u8)
                          n236 = Add Array Elements(numeric array=w844) -> (sum=w842:u8)
                          n237 = Equal?(x=w842, y=w841) -> (x = y?=w843:bool)
                          n238 = case shown="True" w843 {
                            tunnel: w853 -> [_ w867]
                            tunnel: w852 -> [_ w866]
                            tunnel: w849 -> [_ w863]
                            tunnel: w848 -> [_ w862]
                            frame False {
                            }
                            frame True {
                              w858 = u16 4095 ("y")
                              n239 = Join Numbers(hi=w867, lo=w866) -> ((hi.lo)=w859:u16)
                              n240 = Join Numbers(hi=w863, lo=w862) -> ((hi.lo)=w864:u16)
                              n241 = And(x=w858, y=w859) -> (x .and. y?=w857:u16)
                              n242 = Not Equal?(x=w864, y=u16 32767 ("x")) -> (x != y?=w860:bool)
                              n243 = Not Equal?(x=w858, y=w857) -> (x != y?=w861:bool)
                              n244 = case shown="True" w861 {
                                tunnel: w857 -> [_ w879]
                                frame False {
                                }
                                frame True {
                                n245 = To Double Precision Float(number=w879) -> (double precision float=w878:dbl)
                                n246 = Subtract(x=w878, y=2048.0) -> (x-y=w877:dbl)
                                n247 = Multiply(x=w877, y=0.01) -> (x*y=w880:dbl)
                                n248 = global write "G_rio.vi" "mdps torque"(w880) -> ()
                                }
                              }
                              n249 = case shown="True" w860 {
                                tunnel: w864 -> [_ w874]
                                frame False {
                                }
                                frame True {
                                n250 = To Double Precision Float(number=w874) -> (double precision float=w871:dbl)
                                n251 = Subtract(x=w871, y=65536.0) -> (x-y=w872:dbl)
                                n252 = Greater?(x=w871, y=32767.0 ("x")) -> (0:w875:bool)
                                n253 = Select(t=w872, s=w875, f=w871) -> (s? t:f=w870:dbl)
                                n254 = Multiply(x=w870, y=0.1) -> (x*y=w868:dbl)
                                n255 = global write "G_rio.vi" "mdps str_ang"(w868) -> ()
                                }
                              }
                            }
                          }
                        }
                      }
                    }
                    frame 1087 {
                      n256 = flat-sequence {
                        tunnel: [w888] -> w884
                        tunnel: [w887] -> w885
                        tunnel: w883 -> [w886]
                        frame #0 {
                          n257 = xnode "Read/Write Control"("FPGA VI Reference In"=w886) -> ("can 43F"=w893:u8[])  [unwired: 1 in, 2 out]
                          n258 = Index Array(array=w893, index #1=0 ("index")) -> (element #1=w899:u8, element #2=w898:u8, element #3=w897:u8, element #4=w896:u8)  [unwired: 3 in]
                          n259 = Join Numbers(hi=w899, lo=w898) -> ((hi.lo)=w895:u16)
                          n260 = Join Numbers(hi=w897, lo=w896) -> ((hi.lo)=w894:u16)
                          n261 = Join Numbers(hi=w895, lo=w894) -> ((hi.lo)=w889:u32)
                          n262 = Array Subset(array=w893, index=4) -> (w887:u8[])  [unwired: 1 in]
                          n263 = feedback #8(u32 0) -> (w890:u32)
                          n264 = feedback-in #8(w889) -> ()
                          n265 = Not Equal?(x=w889, y=w890) -> (x != y?=w888:bool)
                        }
                      }
                      n266 = case shown="True" w884 {
                        tunnel: w885 -> [_ w906]
                        frame False {
                        }
                        frame True {
                          w903 = u8 15 ("y")
                          # "10ms"
                          n267 = Index Array(array=w906, index=1) -> (element=w904:u8)
                          n268 = And(x=w904, y=w903) -> (x .and. y?=w902:u8)
                          n269 = Not Equal?(x=w902, y=w903) -> (x != y?=w901:bool)
                          n270 = case shown="True" w901 {
                            tunnel: w902 -> [_ w907]
                            frame False {
                            }
                            frame True {
                              n271 = global write "G_rio.vi" "gear selector disp"(w907) -> ()
                            }
                          }
                        }
                      }
                    }
                    frame 1200 {
                      n272 = flat-sequence {
                        tunnel: [w914] -> w909
                        tunnel: [w913] -> w910
                        tunnel: w908 -> [w912]
                        frame #0 {
                          n273 = xnode "Read/Write Control"("FPGA VI Reference In"=w912) -> ("can 4B0"=w918:u8[])  [unwired: 1 in, 2 out]
                          n274 = Index Array(array=w918, index #1=0 ("index")) -> (element #1=w924:u8, element #2=w923:u8, element #3=w922:u8, element #4=w921:u8)  [unwired: 3 in]
                          n275 = Join Numbers(hi=w924, lo=w923) -> ((hi.lo)=w920:u16)
                          n276 = Join Numbers(hi=w922, lo=w921) -> ((hi.lo)=w919:u16)
                          n277 = Join Numbers(hi=w920, lo=w919) -> ((hi.lo)=w911:u32)
                          n278 = Array Subset(array=w918, index=4) -> (w913:u8[])  [unwired: 1 in]
                          n279 = global write "G_rio.vi" "time"(w911) -> ()
                          n280 = feedback #9(u32 0) -> (w915:u32)
                          n281 = feedback-in #9(w911) -> ()
                          n282 = Not Equal?(x=w911, y=w915) -> (x != y?=w914:bool)
                        }
                      }
                      n283 = case shown="True" w909 {
                        tunnel: w910 -> [_ w955]
                        frame False {
                        }
                        frame True {
                          w929 = u16 16383 ("x")
                          w942 = u16 16383 ("x")
                          # "20ms"
                          n284 = Index Array(array=w955, index #1=1 ("index"), index #2=0 ("index"), index #3=3 ("index"), index #4=2 ("index"), index #5=5 ("index"), index #6=4 ("index"), index #7=7 ("index"), index #8=6 ("index")) -> (element #1=w934:u8, element #2=w933:u8, element #3=w932:u8, element #4=w931:u8, element #5=w952:u8, element #6=w951:u8, element #7=w947:u8, element #8=w946:u8)
                          n285 = Join Numbers(hi=w934, lo=w933) -> ((hi.lo)=w930:u16)
                          n286 = Join Numbers(hi=w932, lo=w931) -> ((hi.lo)=w928:u16)
                          n287 = Join Numbers(hi=w952, lo=w951) -> ((hi.lo)=w950:u16)
                          n288 = Join Numbers(hi=w947, lo=w946) -> ((hi.lo)=w943:u16)
                          n289 = And(x=w930, y=w929) -> (x .and. y?=w927:u16)
                          n290 = And(x=w929, y=w928) -> (x .and. y?=w926:u16)
                          n291 = And(x=w950, y=w942) -> (x .and. y?=w941:u16)
                          n292 = And(x=w942, y=w943) -> (x .and. y?=w940:u16)
                          n293 = Not Equal?(x=w941, y=w942) -> (x != y?=w945:bool)
                          n294 = Not Equal?(x=w942, y=w940) -> (x != y?=w944:bool)
                          n295 = And(x=w945, y=w944) -> (x .and. y?=w939:bool)
                          n296 = case shown="True" w939 {
                            tunnel: w941 -> [_ w974]
                            tunnel: w940 -> [_ w973]
                            tunnel: w927 -> [_ w966]
                            tunnel: w926 -> [_ w965]
                            frame False {
                            }
                            frame True {
                              w961 = 0.03125 ("y")
                              w972 = 0.03125 ("y")
                              n297 = To Double Precision Float(number=w966) -> (double precision float=w963:dbl)
                              n298 = To Double Precision Float(number=w965) -> (double precision float=w960:dbl)
                              n299 = To Double Precision Float(number=w974) -> (double precision float=w964:dbl)
                              n300 = To Double Precision Float(number=w973) -> (double precision float=w958:dbl)
                              n301 = Multiply(x=w963, y=w961) -> (x*y=w962:dbl)
                              n302 = Multiply(x=w961, y=w960) -> (x*y=w959:dbl)
                              n303 = Multiply(x=w964, y=w972) -> (x*y=w956:dbl)
                              n304 = Multiply(x=w972, y=w958) -> (x*y=w957:dbl)
                              n305 = global write "G_rio.vi" "WHL_SPD_FL"(w962) -> ()
                              n306 = global write "G_rio.vi" "WHL_SPD_FR"(w959) -> ()
                              n307 = global write "G_rio.vi" "WHL_SPD_RL"(w956) -> ()
                              n308 = global write "G_rio.vi" "WHL_SPD_RR"(w957) -> ()
                              n309 = Add(x=w956, y=w957) -> (x+y=w971:dbl)
                              n310 = Multiply(x=w971, y=0.5) -> (x*y=w968:dbl)
                              n311 = Multiply(x=w968, y=1.028) -> (x*y=w967:dbl)
                              n312 = global write "G_rio.vi" "vs_esc"(w967) -> ()
                            }
                          }
                        }
                      }
                    }
                    frame 1264 {
                      n313 = flat-sequence {
                        tunnel: [w980] -> w976
                        tunnel: [w979] -> w977
                        tunnel: w975 -> [w978]
                        frame #0 {
                          n314 = xnode "Read/Write Control"("FPGA VI Reference In"=w978) -> ("can 4F0"=w985:u8[])  [unwired: 1 in, 2 out]
                          n315 = Index Array(array=w985, index #1=0 ("index")) -> (element #1=w991:u8, element #2=w990:u8, element #3=w989:u8, element #4=w988:u8)  [unwired: 3 in]
                          n316 = Join Numbers(hi=w991, lo=w990) -> ((hi.lo)=w987:u16)
                          n317 = Join Numbers(hi=w989, lo=w988) -> ((hi.lo)=w986:u16)
                          n318 = Join Numbers(hi=w987, lo=w986) -> ((hi.lo)=w981:u32)
                          n319 = Array Subset(array=w985, index=4) -> (w979:u8[])  [unwired: 1 in]
                          n320 = feedback #10(u32 0) -> (w982:u32)
                          n321 = feedback-in #10(w981) -> ()
                          n322 = Not Equal?(x=w981, y=w982) -> (x != y?=w980:bool)
                        }
                      }
                      n323 = case shown="True" w976 {
                        tunnel: w977 -> [_ w1005]
                        frame False {
                        }
                        frame True {
                          # "20 ms"
                          n324 = Index Array(array=w1005, index #1=7 ("index"), index #2=6 ("index"), index #3=5 ("index")) -> (element #1=w999:u8, element #2=w1001:u8, element #3=w1000:u8)
                          n325 = Join Numbers(hi=w1001, lo=w1000) -> ((hi.lo)=w996:u16)
                          n326 = Join Numbers(hi=u8 0, lo=w999) -> ((hi.lo)=w997:u16)
                          n327 = Join Numbers(hi=w997, lo=w996) -> ((hi.lo)=w994:u32)
                          n328 = Not Equal?(x=u32 16777215, y=w994) -> (x != y?=w993:bool)
                          n329 = case shown="True" w993 {
                            tunnel: w994 -> [_ w1007]
                            frame False {
                            }
                            frame True {
                              n330 = To Double Precision Float(number=w1007) -> (double precision float=w1006:dbl)
                              n331 = global write "G_rio.vi" "odometer"(w1006) -> ()
                            }
                          }
                        }
                      }
                    }
                    frame 1349 {
                      n332 = flat-sequence {
                        tunnel: [w1013] -> w1009
                        tunnel: [w1012] -> w1010
                        tunnel: w1008 -> [w1011]
                        frame #0 {
                          n333 = xnode "Read/Write Control"("FPGA VI Reference In"=w1011) -> ("can 545"=w1018:u8[])  [unwired: 1 in, 2 out]
                          n334 = Index Array(array=w1018, index #1=0 ("index")) -> (element #1=w1024:u8, element #2=w1023:u8, element #3=w1022:u8, element #4=w1021:u8)  [unwired: 3 in]
                          n335 = Join Numbers(hi=w1024, lo=w1023) -> ((hi.lo)=w1020:u16)
                          n336 = Join Numbers(hi=w1022, lo=w1021) -> ((hi.lo)=w1019:u16)
                          n337 = Join Numbers(hi=w1020, lo=w1019) -> ((hi.lo)=w1014:u32)
                          n338 = Array Subset(array=w1018, index=4) -> (w1012:u8[])  [unwired: 1 in]
                          n339 = feedback #11(u32 0) -> (w1015:u32)
                          n340 = feedback-in #11(w1014) -> ()
                          n341 = Not Equal?(x=w1014, y=w1015) -> (x != y?=w1013:bool)
                        }
                      }
                      n342 = case shown="True" w1009 {
                        tunnel: w1010 -> [_ w1026]
                        frame False {
                        }
                        frame True {
                          n343 = Index Array(array=w1026, index=3) -> (element=w1028:u8)
                          n344 = Not Equal?(x=w1028, y=u8 255 ("x")) -> (x != y?=w1030:bool)
                          n345 = case shown="True" w1030 {
                            tunnel: w1028 -> [_ w1036]
                            frame False {
                            }
                            frame True {
                              n346 = To Double Precision Float(number=w1036) -> (double precision float=w1035:dbl)
                              n347 = Multiply(x=26.0, y=w1035) -> (x*y=w1033:dbl)
                              n348 = Divide(x=w1033, y=256.0) -> (x/y=w1031:dbl)
                              "battery voltage 2" <- w1031
                              n349 = global write "G_rio.vi" "battery voltage"(w1031) -> ()
                            }
                          }
                        }
                      }
                    }
                    frame 1680 {
                      n350 = flat-sequence {
                        tunnel: [w1042] -> w1038
                        tunnel: [w1041] -> w1039
                        tunnel: w1037 -> [w1040]
                        frame #0 {
                          n351 = xnode "Read/Write Control"("FPGA VI Reference In"=w1040) -> ("can 690"=w1047:u8[])  [unwired: 1 in, 2 out]
                          n352 = Index Array(array=w1047, index #1=0 ("index")) -> (element #1=w1053:u8, element #2=w1052:u8, element #3=w1051:u8, element #4=w1050:u8)  [unwired: 3 in]
                          n353 = Join Numbers(hi=w1053, lo=w1052) -> ((hi.lo)=w1049:u16)
                          n354 = Join Numbers(hi=w1051, lo=w1050) -> ((hi.lo)=w1048:u16)
                          n355 = Join Numbers(hi=w1049, lo=w1048) -> ((hi.lo)=w1043:u32)
                          n356 = Array Subset(array=w1047, index=4) -> (w1041:u8[])  [unwired: 1 in]
                          n357 = feedback #12(u32 0) -> (w1044:u32)
                          n358 = feedback-in #12(w1043) -> ()
                          n359 = Not Equal?(x=w1043, y=w1044) -> (x != y?=w1042:bool)
                        }
                      }
                      n360 = case shown="True" w1038 {
                        tunnel: w1039 -> [_ w1059]
                        frame False {
                        }
                        frame True {
                          n361 = Index Array(array=w1059, index=0) -> (element=w1056:u8)
                          n362 = And(x=u8 3, y=w1056) -> (x .and. y?=→"Key":u8)
                        }
                      }
                    }
                  }
                }
                n363 = Or Array Elements(Boolean array=w666) -> (logical OR=w665:bool)
              }
              frame Disabled {
              }
            }
            "CAN Comm Enabled" <- w663
            n364 = global write "G_rio.vi" "A_CAN"(w663) -> ()
          }
          frame #2 {
            n365 = global read "G_rio.vi" "gear selector disp"() -> (w1064:i8)
            n366 = global read "G_rio.vi" "vs_esc"() -> (w1060:dbl)
            n367 = Negate(x=w1060) -> (-x=w1062:dbl)
            n368 = Equal?(x=w1064, y=u8 7) -> (x = y?=w1063:bool)
            n369 = Select(t=w1062, s=w1063, f=w1060) -> (s? t:f=w1061:dbl)
            "VS_CAN" <- w1061
            n370 = global write "G_rio.vi" "VS_CAN"(w1061) -> ()
          }
          frame #3 {
            n371 = local read "CAN Comm Enabled"() -> (w1066:bool)
            n372 = case shown="True" w1066 {
              frame False {
              }
              frame True {
                n373 = Get Date/Time In Seconds() -> (seconds since 1Jan1904=w1075:timestamp)
                n374 = global read "G_rio.vi" "LCM_CAN_T"() -> (w1092:T6)
                n375 = To Double Precision Float(number=w1075) -> (double precision float=w1074:dbl)
                n376 = global read "G_rio.vi" "accel pedal value"() -> (w1082:dbl)
                n377 = global read "G_rio.vi" "battery voltage"() -> (w1081:dbl)
                n378 = global read "G_rio.vi" "time"() -> (w1094:u32)
                n379 = global read "G_rio.vi" "mcp"() -> (w1093:u16)
                n380 = Unbundle By Name(w1092) -> ("hash"=w1091:i64)
                n381 = global read "G_rio.vi" "mdps str_ang"() -> (w1086:dbl)
                n382 = global read "G_rio.vi" "WHL_SPD_RR"() -> (w1070:dbl)
                n383 = global read "G_rio.vi" "WHL_SPD_RL"() -> (w1069:dbl)
                n384 = global read "G_rio.vi" "WHL_SPD_FR"() -> (w1068:dbl)
                n385 = global read "G_rio.vi" "WHL_SPD_FL"() -> (w1067:dbl)
                n386 = Multiply(x=w1074, y=1000000.0) -> (x*y=w1072:dbl)
                n387 = global read "G_rio.vi" "mdps torque"() -> (w1087:dbl)
                n388 = global read "G_rio.vi" "odometer"() -> (w1079:dbl)
                n389 = global read "G_rio.vi" "yaw_rate"() -> (w1088:dbl)
                n390 = global read "G_rio.vi" "lat_accel"() -> (w1085:dbl)
                n391 = global read "G_rio.vi" "VS_CAN"() -> (w1080:dbl)
                n392 = call "hash.vi"("input"=w1091) -> ("output"=w1090:i64)  [unwired: 10 in]
                n393 = To Quad Integer(1:w1072) -> (0:w1071:i64)
                n394 = To Double Precision Float(number=w1094) -> (double precision float=w1089:dbl)
                n395 = To Double Precision Float(number=w1093) -> (double precision float=w1084:dbl)
                n396 = global read "G_rio.vi" "tps"() -> (w1083:dbl)
                n397 = Bundle By Name(cluster=w1092, "hash"=w1090, "sys time"=w1071, "time"=w1089, "yaw_rate"=w1088, "mdps torque"=w1087, "mdps str_ang"=w1086, "VS_CAN"=w1080, "lat_accel"=w1085, "mcp"=w1084, "accel pedal value"=w1082, "tps"=w1083, "odometer"=w1079, "battery voltage"=w1081, "WHL_SPD_RR"=w1070, "WHL_SPD_RL"=w1069, "WHL_SPD_FR"=w1068, "WHL_SPD_FL"=w1067) -> (w1078:T6)
                n398 = Flatten To String(anything=w1078, prepend array or string size? (T)=FALSE) -> (data string=w1077:string)  [unwired: 2 in, 2 out]
                n399 = disable-structure shown="Enabled" {
                  disable-tunnel: w1077 -> [w1096 _]
                  frame Enabled {
                    n400 = global read "G_rio.vi" "LCM"() -> (w1097:T3)
                    n401 = call "LCM_send.vi"("DATA"=w1096, "ID"="CAN_T", "LCM"=w1097) -> ()  [unwired: 7 in, 2 out]
                  }
                  frame Disabled {
                  }
                }
              }
            }
          }
        }
      }
      n402 = while {
        stop <- FALSE stop-if-true
        n403 = flat-sequence {
          frame #0 {
            n404 = Wait Until Next ms Multiple(millisecond multiple=u32 10) -> (millisecond timer value=w188:u32)
            n405 = flat-sequence {
              tunnel: w188 -> [w192]
              frame #0 {
                n406 = feedback #13(w192) -> (w193:u32)
                n407 = feedback-in #13(w192) -> ()
                n408 = Subtract(x=w192, y=w193) -> (x-y=w191:u32)
                n409 = To Long Integer(number=w191) -> (32bit integer=→"Con_time 10":i32)
              }
            }
          }
          frame #1 {
            n410 = disable-structure shown="Enabled" {
              disable-tunnel: [w216 TRUE ("Auto SW")] -> w197
              frame Disabled {
                n411 = global read "G_rio.vi" "Auto SW"() -> (w216:bool)
              }
              frame Enabled {
              }
            }
            n412 = flat-sequence {
              frame #0 {
                n413 = global read "G_rio.vi" "LCM PC"() -> (w230:T3)
                n414 = call "LCM_read.vi"("LCM"=w230) -> ("data"=w228:string, "ID"=w229:string)  [unwired: 7 in, 2 out]
                n415 = case shown="\"CON_INPUT_T\"" w229 {
                  tunnel: w228 -> [_ w231]
                  frame "False", Default {
                  }
                  frame "CON_INPUT_T" {
                    n416 = global read "G_rio.vi" "CON_INPUT_T 2"() -> (w233:T7)
                    n417 = Unflatten From String(type=w233, binary string=w231, data includes array or string size? (T)=FALSE) -> (value=w232:T7, error out=w234:errorcluster)  [unwired: 2 in, 1 out]
                    n418 = case shown="No Error" w234 {
                      tunnel: w232 -> [w242 _]
                      tunnel: w231 -> [_ w243]
                      frame No Error {
                        w238 = u8 1 ("y")
                        n419 = Unbundle By Name(w242) -> ("ref_vel"=w241:dbl, "ref_steer"=w240:dbl, "alert"=w239:u8)
                        n420 = global write "G_rio.vi" "Ref_vel_planner"(w241) -> ()
                        n421 = global write "G_rio.vi" "Ref_steer_planner"(w240) -> ()
                        n422 = And(x=w239, y=w238) -> (x .and. y?=w237:u8)
                        n423 = Equal?(x=w237, y=w238) -> (x = y?=w236:bool)
                        n424 = global write "G_rio.vi" "A_laser"(w236) -> ()
                      }
                      frame Error {
                        n425 = global read "G_rio.vi" "CON_INPUT_T"() -> (w246:T8)
                        n426 = Unflatten From String(type=w246, binary string=w243, data includes array or string size? (T)=FALSE) -> (value=w248:T8)  [unwired: 2 in, 2 out]
                        n427 = Unbundle By Name(w248) -> ("ref_vel"=w245:dbl, "ref_steer"=w244:dbl)
                        n428 = global write "G_rio.vi" "Ref_vel_planner"(w245) -> ()
                        n429 = global write "G_rio.vi" "Ref_steer_planner"(w244) -> ()
                      }
                    }
                  }
                }
              }
            }
            n430 = global read "G_rio.vi" "Throttle_Enable"() -> (→"Throttle Enable":bool)
            n431 = local read "FPGA"() -> (w213:refnum<k20>)
            n432 = xnode "Read/Write Control"("FPGA VI Reference In"=w213) -> ("Auto"=w196:bool, "Run"=w212:bool, "T Lim"=w214:bool, "brk enc"=w202:u8)  [unwired: 1 in, 2 out]
            "brk enc" <- w202
            n433 = global write "G_rio.vi" "T Lim"(w214) -> ()
            n434 = case shown="True" w197 {
              tunnel: w196 -> [w223 w226]
              tunnel: [_ w225] -> w195
              frame False {
                n435 = case shown="False" w223 {
                  frame False {
                    n436 = global write "G_rio.vi" "Auto SW"(TRUE ("Auto SW")) -> ()
                  }
                  frame True {
                  }
                }
              }
              frame True {
                n437 = case shown="True" w226 {
                  tunnel: [_ TRUE] -> w225
                  frame False {
                  }
                  frame True {
                  }
                }
              }
            }
            "Auto" <- w195
            n438 = To Double Precision Float(number=w202) -> (double precision float=w210:dbl)
            n439 = Subtract(x=w210, y=220.0) -> (x-y=w208:dbl)
            n440 = Multiply(x=w208, y=-100.0) -> (x*y=w205:dbl)
            n441 = Divide(x=w205, y=175.0) -> (x/y=w204:dbl)
            n442 = In Range and Coerce(upper limit=100.0, x=w204, lower limit=0.0) -> (coerced(x)=w201:dbl)  [unwired: 1 out]
            n443 = global write "G_rio.vi" "Auto"(w195) -> ()
            n444 = global write "G_rio.vi" "brake encoder"(w201) -> ()
            n445 = case shown="False" w195 {
              tunnel: [_ w219] -> w194
              frame False {
                n446 = global write "G_rio.vi" "Auto SW counter"(u16 0 ("Auto SW counter")) -> ()
              }
              frame True {
                n447 = global read "G_rio.vi" "brake_act_can"() -> (w222:bool)
                n448 = global read "G_rio.vi" "brake release"() -> (w220:bool)
                n449 = Not(x=w222) -> (.not. x?=w221:bool)
                n450 = Or(x=w220, y=w221) -> (x .or. y?=w219:bool)
              }
            }
            n451 = And(x=w195, y=w212) -> (x .and. y?=w199:bool)
            "Run" <- w199
            n452 = global write "G_rio.vi" "Run"(w199) -> ()
            n453 = Not(x=w199) -> (.not. x?=w198:bool)
            n454 = And(x=w195, y=w198) -> (x .and. y?=→"E - STOP":bool)
            n455 = global write "G_rio.vi" "brake release"(w194) -> ()
          }
          frame #2 {
            n456 = flat-sequence {
              frame #0 {
                n457 = global read "G_rio.vi" "Ref_vel_planner"() -> (w307:dbl)
                n458 = Select(t=w307, s="Velocity input", f="Ref vel manual") -> (s? t:f=w310:dbl)
                n459 = To Long Integer(number=w310) -> (32bit integer=w309:i32)
                n460 = Sign(1:w309) -> (0:w308:i32)
                "P, R, D" <- w308
                n461 = case shown="1" w308 {
                  tunnel: [w314 _ w321] -> w311
                  tunnel: w310 -> [w316 _ w320]
                  frame -1 {
                    n462 = global read "G_rio.vi" "gear selector disp"() -> (w319:i8)
                    n463 = Equal?(x=w319, y=u8 7) -> (x = y?=w317:bool)
                    n464 = Select(t=w316, s=w317, f=0.0) -> (s? t:f=w314:dbl)
                  }
                  frame 0, Default {
                  }
                  frame 1 {
                    n465 = global read "G_rio.vi" "gear selector disp"() -> (w322:i8)
                    n466 = case shown="4, 5" w322 {
                      tunnel: [_ w323] -> w321
                      tunnel: w320 -> [_ w323]
                      frame 0, Default {
                      }
                      frame 4, 5 {
                      }
                    }
                  }
                }
                "Ref vel" <- w311
              }
            }
            n467 = disable-structure shown="Enabled" {
              disable-tunnel: [w251 TRUE ("Steer input")] -> w249
              frame Disabled {
                n468 = feedback #14(FALSE ("Steer input")) -> (w251:bool)
                n469 = Not(x=w251) -> (.not. x?=w250:bool)
                n470 = feedback-in #14(w250) -> ()
              }
              frame Enabled {
              }
            }
            n471 = case shown="True" w249 {
              frame False {
              }
              frame True {
                n472 = flat-sequence {
                  frame #0 {
                    n473 = global read "G_rio.vi" "Ref_steer_planner"() -> (w257:dbl)
                    n474 = global read "G_rio.vi" "mdps str_ang"() -> (w259:dbl)
                    n475 = global read "G_rio.vi" "mdps str_ang"() -> (w260:dbl)
                    n476 = Negate(x="Ref steer manual") -> (-x=w255:dbl)
                    n477 = Select(t=w257, s="Steer input", f=w255) -> (s? t:f=w258:dbl)
                    n478 = Subtract(x=w259, y="steer limit") -> (x-y=w261:dbl)
                    n479 = Add(x=w260, y="steer limit") -> (x+y=w262:dbl)
                    n480 = In Range and Coerce(upper limit=w262, x=w258, lower limit=w261) -> (coerced(x)=→"Ref steer":dbl)  [unwired: 1 out]
                  }
                  frame #1 {
                    w268 = u8 0 ("element")
                    n481 = local read "Ref steer"() -> (w270:dbl)
                    n482 = Multiply(x=w270, y=10.0) -> (x*y=w279:dbl)
                    n483 = Greater Than 0?(x=w279) -> (x > 0?=w280:bool)
                    n484 = Add(x=w279, y=65536.0) -> (x+y=w277:dbl)
                    n485 = Select(t=w279, s=w280, f=w277) -> (s? t:f=w276:dbl)
                    n486 = To Unsigned Word Integer(number=w276) -> (unsigned 16bit integer=w267:u16)
                    n487 = Split Number(x=w267) -> (hi(x)=w275:u8, lo(x)=w274:u8)
                    n488 = Build Array(u8 0 ("Con steer status"), w274, w275, w268, w268, w268, w268) -> (w272:u8[])
                    n489 = global read "G_rio.vi" "Auto"() -> (w282:bool)
                    n490 = Add Array Elements(numeric array=w272) -> (sum=w273:u8)
                    n491 = Build Array (concatenate)(w272, w273) -> (w269:u8[])
                    n492 = And(x=w282, y="SPAS Enable") -> (x .and. y?=w265:bool)
                    n493 = global write "G_rio.vi" "Steering Cont"(w265) -> ()
                    n494 = local read "FPGA"() -> (w266:refnum<k20>)
                    n495 = case shown="True" w265 {
                      tunnel: w269 -> [_ w287]
                      tunnel: w266 -> [w284 w286]
                      frame False {
                        n496 = xnode "Read/Write Control"("FPGA VI Reference In"=w284, "send can"=FALSE) -> ()  [unwired: 1 in, 2 out]
                      }
                      frame True {
                        n497 = disable-structure shown="Enabled" {
                          disable-tunnel: w287 -> [w292 _]
                          disable-tunnel: w286 -> [w288 _]
                          frame Enabled {
                            n498 = flat-sequence {
                              tunnel: w292 -> [w296]
                              tunnel: [w296] -> w291
                              tunnel: [w294] -> w290
                              tunnel: w288 -> [w293]
                              tunnel: w291 -> [w301]
                              tunnel: w290 -> [w299]
                              tunnel: [w298] -> w289
                              tunnel: w289 -> [w304]
                              frame #0 {
                                n499 = xnode "Read/Write Control"("FPGA VI Reference In"=w293, "send can"=TRUE) -> ("FPGA VI Reference Out"=w294:refnum<k20>)  [unwired: 1 in, 1 out]
                              }
                              frame #1 {
                                n500 = Bundle By Name(cluster=T2 {"timestamp high"=0, "timestamp low"=0, "identifier"=0, "type"=enum."Data Frame", "info A"=0, "info B"=0, "data length"=8, "data"=[0, 0, 0, 0, 0, 0, 0, 0]} ("Mod4/CAN1 input"), "identifier"=u32 912, "data"=w301, "data length"=u8 8) -> (w300:T2)
                                n501 = xnode "Read/Write Control"("FPGA VI Reference In"=w299, "Mod4/CAN1 input"=w300) -> ("FPGA VI Reference Out"=w298:refnum<k20>)  [unwired: 1 in, 1 out]
                              }
                              frame #2 {
                                n502 = disable-structure shown="Disabled" {
                                disable-tunnel: w304 -> [w306 _]
                                frame Disabled {
                                n503 = xnode "Read/Write Control"("FPGA VI Reference In"=w306, "send can"=FALSE) -> ()  [unwired: 1 in, 2 out]
                                }
                                frame Enabled {
                                }
                                }
                              }
                            }
                          }
                          frame Disabled {
                          }
                        }
                      }
                    }
                  }
                }
              }
            }
          }
          frame #3 {
            n504 = flat-sequence {
              frame #0 {
                n505 = global read "G_rio.vi" "VS_CAN"() -> (w378:dbl)
                n506 = local read "Ref vel"() -> (w377:dbl)
                n507 = call "T_control.vi"("Ref vel"=w377, "VS_CAN"=w378, "pid gain"=dbl[] [3.0, 0.0, 0.10000000000000003] ("pid gain 1")) -> ("Ref APS"=w380:dbl)  [unwired: 16 in]
                n508 = global write "G_rio.vi" "Ref APS"(w380) -> ()
              }
            }
            n509 = global read "G_rio.vi" "Auto"() -> (w324:bool)
            n510 = case shown="False" w324 {
              tunnel: [w326 w360] -> w325
              frame False {
                n511 = global read "G_rio.vi" "VS_CAN"() -> (w330:dbl)
                n512 = Absolute Value(x=w330) -> (abs(x)=w329:dbl)
                n513 = Less?(x=w329, y=0.05) -> (x < y?=w327:bool)
                n514 = case shown="True" w327 {
                  tunnel: [_ w333] -> w326
                  frame False {
                  }
                  frame True {
                    n515 = Sign(1:"Gear Manual") -> (0:w334:i32)
                    n516 = To Long Integer(number=w334) -> (32bit integer=w332:i32)
                    n517 = case shown="0" w332 {
                      tunnel: [w341 w345 w349] -> w333
                      frame 0 {
                        n518 = global read "G_rio.vi" "gear selector disp"() -> (w339:i8)
                        n519 = Equal To 0?(x=w339) -> (x = 0?=w338:bool)
                        n520 = Equal?(x=u8 7 ("y"), y=w339) -> (x = y?=w343:bool)
                        n521 = Select(t=-1.0, s=w338, f=1.0) -> (s? t:f=w337:dbl)
                        n522 = Select(t=0.0, s=w343, f=w337) -> (s? t:f=w341:dbl)
                      }
                      frame 1, Default {
                        n523 = global read "G_rio.vi" "gear selector disp"() -> (w348:i8)
                        n524 = Equal To 0?(x=w348) -> (x = 0?=w347:bool)
                        n525 = Select(t=0.0, s=w347, f=1.0 ("t")) -> (s? t:f=w345:dbl)
                      }
                      frame -1 {
                        n526 = global read "G_rio.vi" "gear selector disp"() -> (w350:i8)
                        n527 = case shown="3..5, Default" w350 {
                          tunnel: [-1.0 1.0 0.0] -> w349
                          frame 0, 6, 7 {
                          }
                          frame 1, 2 {
                          }
                          frame 3..5, Default {
                          }
                        }
                      }
                    }
                  }
                }
              }
              frame True {
                n528 = global read "G_rio.vi" "VS_CAN"() -> (w357:dbl)
                n529 = Absolute Value(x=w357) -> (abs(x)=w356:dbl)
                n530 = Less?(x=w356, y=0.05) -> (x < y?=w354:bool)
                n531 = global read "G_rio.vi" "Run"() -> (w359:bool)
                n532 = And(x=w354, y=w359) -> (x .and. y?=w358:bool)
                n533 = case shown="True" w358 {
                  tunnel: [_ w362] -> w360
                  frame False {
                  }
                  frame True {
                    n534 = local read "P, R, D"() -> (w361:i32)
                    n535 = case shown="-1" w361 {
                      tunnel: [w363 w368 w372] -> w362
                      frame -1 {
                        n536 = global read "G_rio.vi" "gear selector disp"() -> (w364:i8)
                        n537 = case shown="0" w364 {
                          tunnel: [-1.0 ("t") 1.0 ("t") _ _] -> w363
                          frame 0 {
                          }
                          frame 1, Default {
                          }
                          frame 4, 8 {
                          }
                          frame 7 {
                          }
                        }
                      }
                      frame 0, Default {
                        n538 = global read "G_rio.vi" "gear selector disp"() -> (w371:i8)
                        n539 = Equal To 0?(x=w371) -> (x = 0?=w370:bool)
                        n540 = Select(t=0.0, s=w370, f=1.0 ("t")) -> (s? t:f=w368:dbl)
                      }
                      frame 1 {
                        n541 = global read "G_rio.vi" "gear selector disp"() -> (w373:i8)
                        n542 = case shown="1, 2" w373 {
                          tunnel: [-1.0 1.0 0.0] -> w372
                          frame 0, 6, 7 {
                          }
                          frame 1, 2 {
                          }
                          frame 3..5, Default {
                          }
                        }
                      }
                    }
                  }
                }
              }
            }
            "shift lever" <- w325
          }
          frame #4 {
            n543 = flat-sequence {
              tunnel: [w386] -> w382
              tunnel: [w385] -> w381
              tunnel: w382 -> [w609]
              tunnel: w381 -> [w610]
              frame #0 {
                n544 = flat-sequence {
                  tunnel: [w442] -> w387
                  frame #0 {
                    n545 = global read "G_rio.vi" "accel pedal value"() -> (w434:dbl)
                    n546 = Equal To 0?(x=w434) -> (x = 0?=w433:bool)
                    n547 = case shown="True" w433 {
                      tunnel: [TRUE w445] -> w436
                      frame False {
                        n548 = global write "G_rio.vi" "T lim counter 2"(u16 300 ("T lim counter 2")) -> ()
                      }
                      frame True {
                        n549 = global read "G_rio.vi" "T lim counter 2"() -> (w447:u16)
                        n550 = Decrement(x=w447) -> (x-1=w448:u16)
                        n551 = Max & Min(x=u16 0, y=w448) -> (max(x,y)=w446:u16)  [unwired: 1 out]
                        n552 = global write "G_rio.vi" "T lim counter 2"(w446) -> ()
                        n553 = Not Equal To 0?(x=w446) -> (x != 0?=w445:bool)
                      }
                    }
                    n554 = global read "G_rio.vi" "brake_act_can"() -> (w435:bool)
                    n555 = global read "G_rio.vi" "Throttle_Enable"() -> (w439:bool)
                    n556 = local read "Ref vel"() -> (w432:dbl)
                    n557 = Not Equal To 0?(x=w432) -> (x != 0?=w441:bool)
                    n558 = Not(x=w435) -> (.not. x?=w440:bool)
                    n559 = global read "G_rio.vi" "Auto"() -> (w437:bool)
                    n560 = global read "G_rio.vi" "Run"() -> (w438:bool)
                    n561 = Compound Arithmetic op=AND(w437, w438, w441, w440, w439, w436) -> (w442:bool)
                  }
                }
                n562 = global read "G_rio.vi" "Auto"() -> (w383:bool)
                n563 = case shown="True" w383 {
                  tunnel: [1000.0 ("f") w392] -> w384
                  frame False {
                  }
                  frame True {
                    n564 = global read "G_rio.vi" "VS_CAN"() -> (w390:dbl)
                    n565 = local read "Ref vel"() -> (w395:dbl)
                    n566 = Subtract(x=w395, y=w390) -> (x-y=w394:dbl)
                    n567 = Less?(x=w394, y=-2.0 ("lower limit")) -> (x < y?=w396:bool)
                    n568 = case shown="True" w396 {
                      tunnel: w394 -> [w399 w429]
                      tunnel: [w400 w419] -> w393
                      tunnel: w395 -> [w404 w420]
                      frame False {
                        n569 = Equal To 0?(x=w404) -> (x = 0?=w403:bool)
                        n570 = global read "G_rio.vi" "PWM Brake"() -> (w398:dbl)
                        n571 = Greater?(x=w399, y=1.0) -> (0:w408:bool)
                        n572 = Multiply(x=w398, y=0.999) -> (x*y=w410:dbl)
                        n573 = Max & Min(x=w410, y=1000.0) -> (max(x,y)=w406:dbl)  [unwired: 1 out]
                        n574 = Select(t=1000.0, s=w408, f=w406) -> (s? t:f=w401:dbl)
                        n575 = Select(t=2000.0, s=w403, f=w401) -> (s? t:f=w400:dbl)
                      }
                      frame True {
                        w417 = 0.5 ("gain brake")
                        w426 = 10.0 ("y")
                        n576 = Absolute Value(x=w429) -> (abs(x)=w428:dbl)
                        n577 = Add(x=w428, y=w426) -> (x+y=w427:dbl)
                        n578 = Multiply(x=w427, y=w426) -> (x*y=w425:dbl)
                        n579 = Threshold 1D Array(2:w425, 3:dbl[] [10.0, 15.0, 25.0, 50.0, 80.0, 120.0, 170.0, 230.0, 290.0, 350.0, 420.0]) -> (0:w423:dbl)  [unwired: 1 in]
                        n580 = global read "G_rio.vi" "PWM Brake"() -> (w412:dbl)
                        n581 = Interpolate 1D Array(1:w423, 2:dbl[] [1000.0, 1100.0, 1200.0, 1300.0, 1400.0, 1500.0, 1600.0, 1700.0, 1800.0, 1900.0, 2000.0]) -> (0:w418:dbl)
                        n582 = Decrement(x=w417) -> (x-1=w416:dbl)
                        n583 = Multiply(x=w418, y=w417) -> (x*y=w414:dbl)
                        n584 = Multiply(x=w416, y=w412) -> (x*y=w415:dbl)
                        n585 = Subtract(x=w414, y=w415) -> (x-y=w413:dbl)
                        n586 = Equal To 0?(x=w420) -> (x = 0?=w421:bool)
                        n587 = Select(t=2000.0, s=w421, f=w413) -> (s? t:f=w419:dbl)
                      }
                    }
                    n588 = global read "G_rio.vi" "Run"() -> (w389:bool)
                    n589 = Select(t=w393, s=w389, f=2000.0) -> (s? t:f=w392:dbl)
                  }
                }
                n590 = case shown="True" w387 {
                  tunnel: [_ TRUE] -> w386
                  tunnel: [w450 w469] -> w385
                  frame False {
                    n591 = flat-sequence {
                      tunnel: [w460] -> w450
                      frame #0 {
                        n592 = global read "G_rio.vi" "T Lim"() -> (w451:bool)
                        n593 = case shown="True" w451 {
                          selector: w451 -> [_ w458]
                          frame False {
                            n594 = global write "G_rio.vi" "T lim counter"(u16 0 ("T lim counter")) -> ()
                          }
                          frame True {
                            n595 = global write "G_rio.vi" "T lim once"(w458) -> ()
                            n596 = global write "G_rio.vi" "T lim counter 2"(u16 300 ("T lim counter 2")) -> ()
                            n597 = global read "G_rio.vi" "T lim counter"() -> (w457:u16)
                            n598 = Increment(x=w457) -> (x+1=w456:u16)
                            n599 = Max & Min(x=u16 100, y=w456) -> (min(x,y)=w455:u16)  [unwired: 1 out]
                            n600 = global write "G_rio.vi" "T lim counter"(w455) -> ()
                          }
                        }
                      }
                      frame #1 {
                        n601 = global read "G_rio.vi" "T lim once"() -> (w459:bool)
                        n602 = case shown="True" w459 {
                          tunnel: [-1.0 ("t") w465] -> w460
                          frame False {
                          }
                          frame True {
                            n603 = global read "G_rio.vi" "T lim counter"() -> (w464:u16)
                            n604 = Equal?(x=w464, y=u16 100) -> (x = y?=w463:bool)
                            n605 = Select(t=0.0, s=w463, f=-0.15) -> (s? t:f=w465:dbl)
                          }
                        }
                        n606 = global write "G_rio.vi" "Throttle_Enable"(w459) -> ()
                      }
                    }
                  }
                  frame True {
                    n607 = disable-structure shown="Enabled" {
                      disable-tunnel: [w488 w544] -> w469
                      frame Enabled {
                        n608 = global read "G_rio.vi" "accel pedal value"() -> (w492:dbl)
                        n609 = global read "G_rio.vi" "Ref APS"() -> (w493:dbl)
                        n610 = global read "G_rio.vi" "accel pedal value"() -> (w491:dbl)
                        n611 = global read "G_rio.vi" "accel pedal value"() -> (w480:dbl)
                        n612 = Subtract(x=w493, y=w492) -> (x-y=w479:dbl)
                        n613 = flat-sequence {
                          tunnel: w479 -> [w514]
                          tunnel: [w511] -> w487
                          frame #0 {
                            n614 = feedback #15(0.0) -> (w519:dbl)
                            n615 = feedback-in #15(w514) -> ()
                            n616 = Multiply(x=w514, y=0.01) -> (x*y=w515:dbl)
                            n617 = Subtract(x=w514, y=w519) -> (x-y=w518:dbl)
                            n618 = feedback #16(0.0) -> (w510:dbl)
                            n619 = Multiply(x=0.999, y=w510) -> (x*y=w509:dbl)
                            n620 = Divide(x=w518, y=0.01) -> (x/y=w505:dbl)
                            n621 = Add(x=w515, y=w509) -> (x+y=w506:dbl)
                            n622 = feedback-in #16(w506) -> ()
                            n623 = Build Array(w514, w506, w505) -> (w513:dbl[])
                            n624 = Multiply(x=w513, y=dbl[] [8.0, 0.02, 0.4] ("pid gain 2")) -> (x*y=w512:dbl[])
                            n625 = Add Array Elements(numeric array=w512) -> (sum=w511:dbl)
                          }
                        }
                        n626 = Greater Than 0?(x=w479) -> (x > 0?=w481:bool)
                        n627 = Less Than 0?(x=w479) -> (x < 0?=w473:bool)
                        n628 = Equal To 0?(x=w480) -> (x = 0?=w472:bool)
                        n629 = Greater?(x=w491, y=95.0) -> (0:w482:bool)
                        n630 = And(x=w482, y=w481) -> (x .and. y?=w477:bool)
                        n631 = And(x=w472, y=w473) -> (x .and. y?=w478:bool)
                        n632 = Or(x=w477, y=w478) -> (x .or. y?=w476:bool)
                        n633 = Multiply(x=w487, y=0.01) -> (x*y=w485:dbl)
                        n634 = In Range and Coerce(upper limit=1.0 ("x"), x=w485, lower limit=-1.0) -> (coerced(x)=w475:dbl)  [unwired: 1 out]
                        n635 = flat-sequence {
                          tunnel: w475 -> [w495]
                          tunnel: [w501] -> w474
                          frame #0 {
                            w494 = 0.5 ("x")
                            n636 = Multiply(x=w495, y=w494) -> (x*y=w499:dbl)
                            n637 = Subtract(x=1.0, y=w494) -> (x-y=w497:dbl)
                            n638 = feedback #17(0.0) -> (w496:dbl)
                            n639 = Multiply(x=w497, y=w496) -> (x*y=w498:dbl)
                            n640 = Add(x=w499, y=w498) -> (x+y=w501:dbl)
                            n641 = feedback-in #17(w501) -> ()
                          }
                        }
                        n642 = Select(t=0.0 ("f"), s=w476, f=w474) -> (s? t:f=w488:dbl)
                      }
                      frame Disabled {
                        n643 = global read "G_rio.vi" "VS_CAN"() -> (w546:dbl)
                        n644 = global read "G_rio.vi" "VS_CAN"() -> (w532:dbl)
                        n645 = local read "Ref vel"() -> (w547:dbl)
                        n646 = Divide(x=w532, y=3.6) -> (x/y=w530:dbl)
                        n647 = Subtract(x=w547, y=w546) -> (x-y=w525:dbl)
                        n648 = feedback #18(0.0 ("y")) -> (w537:dbl)
                        n649 = feedback-in #18(w530) -> ()
                        n650 = Subtract(x=w530, y=w537) -> (x-y=w536:dbl)
                        n651 = Divide(x=w525, y=3.6) -> (x/y=w521:dbl)
                        n652 = Divide(x=dbl[] [-100.0, -3.0, -1.0, 1.0, 3.0, 100.0] ("array_x"), y=3.6) -> (x/y=w522:dbl[])
                        n653 = call "lookuptable.vi"("array_y"=dbl[] [-0.5, -0.1, -0.01, 0.01, 0.1, 0.5] ("array_x"), "array_x"=w522, "x"=w521) -> ("y"=w540:dbl)  [unwired: 8 in]
                        n654 = Multiply(x=100.0, y=w536) -> (x*y=w534:dbl)
                        n655 = Multiply(x=1.0 ("P_gain"), y=w540) -> (x*y=w529:dbl)
                        n656 = Multiply(x=0.0 ("D_gain"), y=w534) -> (x*y=w528:dbl)
                        n657 = Subtract(x=w529, y=w528) -> (x-y=w527:dbl)
                        n658 = flat-sequence {
                          tunnel: w527 -> [w549]
                          tunnel: [w548] -> w520
                          frame #0 {
                            n659 = feedback #19(0.0 ("y")) -> (w556:dbl)
                            n660 = Multiply(x=-0.01, y=999.0) -> (x*y=w555:dbl)
                            n661 = Multiply(x=0.7 ("Rate"), y=0.01 ("x")) -> (x*y=w551:dbl)
                            n662 = Add(x=w556, y=w555) -> (x+y=w557:dbl)
                            n663 = Add(x=w551, y=w556) -> (x+y=w558:dbl)
                            n664 = In Range and Coerce(upper limit=w558, x=w549, lower limit=w557) -> (coerced(x)=w548:dbl)  [unwired: 1 out]
                            n665 = feedback-in #19(w548) -> ()
                          }
                        }
                        n666 = In Range and Coerce(upper limit=1.0, x=w520, lower limit=-1.0) -> (coerced(x)=w541:dbl)  [unwired: 1 out]
                        n667 = flat-sequence {
                          tunnel: w541 -> [w561]
                          tunnel: [w560] -> w544
                          frame #0 {
                            n668 = Greater Than 0?(x=w561) -> (x > 0?=w569:bool)
                            n669 = global read "G_rio.vi" "accel pedal value"() -> (w572:dbl)
                            n670 = global read "G_rio.vi" "accel pedal value"() -> (w568:dbl)
                            n671 = Less Than 0?(x=w561) -> (x < 0?=w567:bool)
                            n672 = Equal To 0?(x=w568) -> (x = 0?=w566:bool)
                            n673 = Greater?(x=w572, y=95.0) -> (0:w570:bool)
                            n674 = And(x=w570, y=w569) -> (x .and. y?=w565:bool)
                            n675 = And(x=w567, y=w566) -> (x .and. y?=w564:bool)
                            n676 = Or(x=w565, y=w564) -> (x .or. y?=w563:bool)
                            n677 = Select(t=0.0, s=w563, f=w561) -> (s? t:f=w560:dbl)
                          }
                        }
                      }
                    }
                    n678 = global write "G_rio.vi" "T lim counter"(u16 0 ("T lim counter")) -> ()
                    n679 = global write "G_rio.vi" "T lim once"(FALSE ("T lim once")) -> ()
                  }
                }
                n680 = disable-structure shown="Enabled" {
                  disable-tunnel: w384 -> [w431 _]
                  frame Enabled {
                    n681 = global write "G_rio.vi" "PWM Brake"(w431) -> ()
                  }
                  frame Disabled {
                  }
                }
              }
              frame #1 {
                n682 = local read "shift lever"() -> (w589:dbl)
                n683 = disable-structure shown="Enabled" {
                  disable-tunnel: [w611 w616] -> w578
                  frame Disabled {
                    n684 = global read "G_rio.vi" "accel pedal value"() -> (w614:dbl)
                    n685 = global read "G_rio.vi" "Ref APS"() -> (w615:dbl)
                    n686 = Equal To 0?(x=w615) -> (x = 0?=w612:bool)
                    n687 = Not Equal To 0?(x=w614) -> (x != 0?=w613:bool)
                    n688 = And(x=w612, y=w613) -> (x .and. y?=w611:bool)
                  }
                  frame Enabled {
                    n689 = global read "G_rio.vi" "accel pedal value"() -> (w617:dbl)
                    n690 = global read "G_rio.vi" "Ref APS"() -> (w618:dbl)
                    n691 = Subtract(x=w617, y=w618) -> (x-y=w619:dbl)
                    n692 = Greater?(x=w619, y=5.0) -> (0:w616:bool)
                  }
                }
                n693 = Multiply(x=w610, y=500.0 ("T gain")) -> (x*y=w607:dbl)
                n694 = disable-structure shown="Enabled" {
                  disable-tunnel: [w628 _] -> w588
                  frame Enabled {
                    n695 = global read "G_rio.vi" "Auto"() -> (w632:bool)
                    n696 = global read "G_rio.vi" "Run"() -> (w631:bool)
                    n697 = Compound Arithmetic op=AND(w632, w631) -> (w630:bool)
                    n698 = And(x=w630, y="buzz") -> (x .and. y?=w628:bool)
                  }
                  frame Disabled {
                  }
                }
                n699 = Multiply(x=w589, y=250.0 ("S gain")) -> (x*y=w597:dbl)
                n700 = In Range and Coerce(upper limit=500.0, x=w607, lower limit=-500.0) -> (coerced(x)=w591:dbl)  [unwired: 1 out]
                n701 = global read "G_rio.vi" "PWM Brake"() -> (w584:dbl)
                n702 = global read "G_rio.vi" "PWM Brake"() -> (w586:dbl)
                n703 = In Range and Coerce(upper limit=500.0, x=w597, lower limit=-500.0) -> (coerced(x)=w600:dbl)  [unwired: 1 out]
                n704 = global read "G_rio.vi" "mdps torque"() -> (w576:dbl)
                n705 = Add(x=w591, y=1500.0) -> (x+y=w603:dbl)
                n706 = global read "G_rio.vi" "brake_act_can"() -> (w581:bool)
                n707 = global read "G_rio.vi" "brake release"() -> (w580:bool)
                n708 = Equal?(x=w584, y=1000.0) -> (x = y?=w582:bool)
                n709 = Add(x=w600, y=1500.0) -> (x+y=w602:dbl)
                n710 = Select(t=w586, s="brake", f="Slide") -> (s? t:f=w585:dbl)
                n711 = Absolute Value(x=w576) -> (abs(x)=w573:dbl)
                "mdps torque" <- w573
                n712 = To Unsigned Word Integer(number=w603) -> (unsigned 16bit integer=w587:u16)
                "T PWM" <- w587
                n713 = Compound Arithmetic op=AND(w582, w581, w580) -> (w579:bool)
                n714 = To Unsigned Word Integer(number=w602) -> (unsigned 16bit integer=w590:u16)
                n715 = To Unsigned Word Integer(number=w585) -> (unsigned 16bit integer=w594:u16)
                "B PWM" <- w594
                n716 = Greater?(x=w573, y=5.0) -> (0:w574:bool)
                n717 = local read "FPGA"() -> (w595:refnum<k20>)
                n718 = Compound Arithmetic op=OR(w574, w579, w578) -> (w577:bool)
                n719 = case shown="True" w577 {
                  frame False {
                    n720 = global write "G_rio.vi" "Auto SW counter"(u16 0 ("Auto SW counter")) -> ()
                  }
                  frame True {
                    w624 = u16 40 ("x")
                    n721 = global read "G_rio.vi" "Auto SW counter"() -> (w626:u16)
                    n722 = Increment(x=w626) -> (x+1=w625:u16)
                    n723 = Max & Min(x=w624, y=w625) -> (min(x,y)=w623:u16)  [unwired: 1 out]
                    n724 = Equal?(x=w624, y=w623) -> (x = y?=w622:bool)
                    n725 = global write "G_rio.vi" "Auto SW counter"(w623) -> ()
                    n726 = case shown="True" w622 {
                      frame False {
                      }
                      frame True {
                        n727 = global write "G_rio.vi" "Auto SW"(FALSE ("Auto SW")) -> ()
                      }
                    }
                  }
                }
                n728 = xnode "Read/Write Control"("FPGA VI Reference In"=w595, "Buzz"=w588, "S Pwm 1"=w590, "S Pwm 2"=w590, "B Pwm"=w594, "T Pwm"=w587, "Solenoid"=w609) -> ()  [unwired: 1 in, 2 out]
                "solenoid" <- w609
              }
              frame #2 {
                n729 = Get Date/Time In Seconds() -> (seconds since 1Jan1904=w637:timestamp)
                n730 = global read "G_rio.vi" "LCM_CON_T"() -> (w656:T9)
                n731 = To Double Precision Float(number=w637) -> (double precision float=w636:dbl)
                n732 = Unbundle By Name(w656) -> ("hash"=w654:i64)
                n733 = Multiply(x=w636, y=1000000.0) -> (x*y=w634:dbl)
                n734 = global read "G_rio.vi" "Ref Brk Enc"() -> (w640:dbl)
                n735 = local read "solenoid"() -> (w645:bool)
                n736 = local read "Ref steer"() -> (w638:dbl)
                n737 = global read "G_rio.vi" "Ref APS"() -> (w639:dbl)
                n738 = local read "brk enc"() -> (w644:u8)
                n739 = local read "B PWM"() -> (w643:u16)
                n740 = local read "T PWM"() -> (w642:u16)
                n741 = To Quad Integer(1:w634) -> (0:w633:i64)
                n742 = call "hash.vi"("input"=w654) -> ("output"=w653:i64)  [unwired: 10 in]
                n743 = local read "Ref vel"() -> (w641:dbl)
                n744 = global read "G_rio.vi" "T Lim"() -> (w646:bool)
                n745 = global read "G_rio.vi" "Auto"() -> (w648:bool)
                n746 = global read "G_rio.vi" "Run"() -> (w647:bool)
                n747 = Bundle(cluster=w656, "hash"=w653, "sys time"=w633, "Auto"=w648, "Run"=w647, "Solenoid"=w645, "T lim"=w646, "brk_enc"=w644, "B PWM"=w643, "T PWM"=w642, "ref_vel"=w641, "ref_bkr_enc"=w640, "ref_apv"=w639, "ref_steer"=w638) -> (w649:T9)
                n748 = Flatten To String(anything=w649, prepend array or string size? (T)=FALSE) -> (data string=w651:string)  [unwired: 2 in, 2 out]
                n749 = global read "G_rio.vi" "LCM"() -> (w650:T3)
                n750 = call "LCM_send.vi"("DATA"=w651, "ID"="CON_T", "LCM"=w650) -> ()  [unwired: 7 in, 2 out]
              }
            }
          }
        }
      }
    }
  }
  n751 = flat-sequence {
    tunnel: [dbl[] [0.0, 0.0, 0.0, 0.0, 0.0] ("pos(i)")] -> w1
    tunnel: w1 -> [w1106]
    frame #0 {
      w1102 = FALSE ("get heading")
      w1105 = u64 1
      w1104 = 0.0 ("dh_hat")
      n752 = local write "GPS init"(w1102) -> ()
      n753 = call "getecefdcmref.vi"("map name"="map name") -> ("XYZ"=→"ecef ref":dbl[])  [unwired: 10 in, 4 out]
      "vgain" <- 1.0 ("initH")
      "vcount" <- w1105
      "hbias" <- 0.02314872284554697 ("hbias")
      "hcount" <- w1105
      "get heading" <- w1102
      "get position" <- w1102
      "heading error" <- w1104
      "h_gps" <- w1104
      "rt" <- w1104
      "pos error" <- w1104
      "map" <- "map name"
    }
    frame #1 {
      n754 = disable-structure shown="Enabled" {
        frame Disabled {
          n755 = while {
            stop <- FALSE stop-if-true
            n756 = flat-sequence {
              frame #0 {
                n757 = Wait Until Next ms Multiple(millisecond multiple=u32 50) -> ()  [unwired: 1 out]
              }
              frame #1 {
                n758 = local read item#-1() -> (w1111)
                n759 = xnode "Read/Write Control"("FPGA VI Reference In"=w1111) -> ("FPGA VI Reference Out"=w1109:refnum<k20>, "Connection error GPS 1"=w1110:bool)  [unwired: 1 in, 1 out]
                n760 = case shown="False" w1110 {
                  tunnel: w1109 -> [w1113 w1233]
                  frame False {
                    n761 = flat-sequence {
                      tunnel: w1113 -> [w1115]
                      tunnel: [w1114] -> w1112
                      tunnel: w1112 -> [w1134]
                      frame #0 {
                        n762 = while {
                          tunnel: w1115 -> [w1119]
                          tunnel: [w1117] -> w1114
                          stop <- w1118 stop-if-true
                          n763 = flat-sequence {
                            tunnel: w1119 -> [w1121]
                            tunnel: [w1121] -> w1116
                            tunnel: [w1124] -> w1118
                            tunnel: [w1123] -> w1117
                            tunnel: w1116 -> [w1130]
                            frame #0 {
                              n764 = Wait Until Next ms Multiple(millisecond multiple=u32 20) -> ()  [unwired: 1 out]
                            }
                            frame #1 {
                              n765 = xnode "Invoke Method"("FPGA VI Reference In"=w1130, "Number of Elements"=u32 1, "Timeout (ms)"=1) -> ("FPGA VI Reference Out"=w1123:refnum<k20>, "Data"=w1125:u8[])  [unwired: 1 in, 2 out]
                              n766 = Index Array(array=w1125, index=0) -> (element=w1127:u8)
                              n767 = Equal?(x=w1127, y=u8 170) -> (x = y?=w1124:bool)
                            }
                          }
                        }
                      }
                      frame #1 {
                        w1135 = u32 3 ("Number of Elements")
                        n768 = xnode "Invoke Method"("FPGA VI Reference In"=w1134, "Number of Elements"=w1135, "Timeout (ms)"=w1135) -> ("FPGA VI Reference Out"=w1133:refnum<k20>, "Data"=w1137:u8[], "Elements Remaining"=w1131:u32)  [unwired: 1 in, 1 out]
                        n769 = Equal?(x=w1137, y=u8[] [68, 18, 28]) -> (x = y?=w1138:bool[])
                        n770 = And Array Elements(Boolean array=w1138) -> (logical AND=w1132:bool)
                        n771 = case shown="True" w1132 {
                          tunnel: w1133 -> [w1141 w1146]
                          tunnel: w1131 -> [w1140 _]
                          frame False {
                            n772 = xnode "Invoke Method"("FPGA VI Reference In"=w1141, "Number of Elements"=w1140, "Timeout (ms)"=1) -> ()  [unwired: 1 in, 4 out]
                          }
                          frame True {
                            w1142 = u32 8 ("Number of Elements")
                            n773 = xnode "Invoke Method"("FPGA VI Reference In"=w1146, "Number of Elements"=w1142, "Timeout (ms)"=w1142) -> ("FPGA VI Reference Out"=w1159:refnum<k20>, "error out"=w1160:errorcluster, "Data"=w1162:u8[])  [unwired: 1 in, 1 out]
                            n774 = Index Array(array=w1162, index #1=1 ("index"), index #2=0 ("index"), index #3=5 ("index"), index #4=4 ("index")) -> (element #1=w1149:u8, element #2=w1150:u8, element #3=w1154:u8, element #4=w1155:u8)
                            n775 = Join Numbers(hi=w1154, lo=w1155) -> ((hi.lo)=w1156:u16)
                            n776 = Join Numbers(hi=w1149, lo=w1150) -> ((hi.lo)=w1151:u16)
                            n777 = Add(x=w1156, y=u16 20) -> (x+y=w1158:u16)
                            n778 = xnode "Invoke Method"("FPGA VI Reference In"=w1159, "error in"=w1160, "Number of Elements"=w1158, "Timeout (ms)"=10) -> ("Data"=w1144:u8[])  [unwired: 3 out]
                            n779 = Empty Array?(array=w1144) -> (empty?=w1143:bool)
                            n780 = Build Array (concatenate)(u8[] [170, 68, 18, 28], w1162, w1144) -> (w1163:u8[])
                            n781 = case shown="False" w1143 {
                              tunnel: w1163 -> [w1165 _]
                              tunnel: w1151 -> [w1164 _]
                              frame False {
                                n782 = case shown="99" w1164 {
                                tunnel: w1165 -> [_ w1168 w1206]
                                frame 0, Default {
                                }
                                frame 42 {
                                n783 = local read "ecef ref"() -> (w1167:dbl[])
                                n784 = call "novatel_bestpos.vi"("ecef ref"=w1167, "gps_data"=w1168) -> ("LCC"=w1166:dbl[])  [unwired: 9 in]
                                n785 = flat-sequence {
                                tunnel: w1166 -> [w1171]
                                frame #0 {
                                n786 = Index Array(array=w1171, index=1) -> (element=w1174:dbl)
                                n787 = Not Equal To 0?(x=w1174) -> (x != 0?=w1170:bool)
                                n788 = local read item#-1() -> (w1173)
                                n789 = And(x=w1170, y=w1173) -> (x .and. y?=w1169:bool)
                                n790 = case shown="True" w1169 {
                                tunnel: w1171 -> [_ w1194]
                                frame False {
                                }
                                frame True {
                                n791 = Get Date/Time In Seconds() -> (seconds since 1Jan1904=w1179:timestamp)
                                n792 = To Double Precision Float(number=w1179) -> (double precision float=w1178:dbl)
                                n793 = global read "G_rio.vi" "LCM_GGA_T"() -> (w1203:T11)
                                n794 = Array To Cluster(array=w1194) -> (cluster=w1202:T12)
                                n795 = Unbundle By Name(w1203) -> ("hash"=w1199:i64)
                                n796 = Multiply(x=w1178, y=1000000.0) -> (x*y=w1176:dbl)
                                n797 = Unbundle(w1202) -> ("LCC[0]"=w1204:dbl, "LCC[2]"=w1193:dbl, "LCC[3]"=w1192:dbl, "LCC[4]"=w1191:dbl, "LCC[6]"=w1190:dbl, "LCC[7]"=w1188:dbl, "LCC[8]"=w1186:dbl, "LCC[9]"=w1184:dbl, "LCC[12]"=w1183:dbl, "LCC[13]"=w1182:dbl, "LCC[14]"=w1181:dbl)  [unwired: 4 out]
                                n798 = To Quad Integer(1:w1176) -> (0:w1175:i64)
                                n799 = To Long Integer(number=w1190) -> (32bit integer=w1189:i32)
                                n800 = To Long Integer(number=w1188) -> (32bit integer=w1187:i32)
                                n801 = To Long Integer(number=w1186) -> (32bit integer=w1185:i32)
                                n802 = call "hash.vi"("input"=w1199) -> ("output"=w1198:i64)  [unwired: 10 in]
                                n803 = local read "map"() -> (w1180:i32)
                                n804 = Bundle(cluster=w1203, "hash"=w1198, "sys time"=w1175, "time"=w1204, "x"=w1193, "y"=w1192, "h"=w1191, "numSV"=w1189, "postype"=w1187, "lag"=w1185, "hordev"=w1184, "lat"=w1183, "lon"=w1182, "hgt"=w1181, "map_idx"=w1180) -> (w1200:T11)
                                n805 = Flatten To String(anything=w1200, prepend array or string size? (T)=FALSE) -> (data string=w1196:string)  [unwired: 2 in, 2 out]
                                n806 = global read "G_rio.vi" "LCM"() -> (w1195:T3)
                                n807 = call "LCM_send.vi"("DATA"=w1196, "ID"="GGA_DGPS", "LCM"=w1195) -> ()  [unwired: 7 in, 2 out]
                                }
                                }
                                }
                                }
                                n808 = global write "G_rio.vi" "dgps_pos"(w1166) -> ()
                                }
                                frame 99 {
                                n809 = call "novatel_bestvel.vi"("gps_data"=w1206) -> ("vel"=w1205:dbl[])  [unwired: 10 in]
                                n810 = flat-sequence {
                                tunnel: w1205 -> [w1208]
                                frame #0 {
                                n811 = Index Array(array=w1208, index=1) -> (element=w1211:dbl)
                                n812 = Not Equal To 0?(x=w1211) -> (x != 0?=w1212:bool)
                                n813 = local read item#-1() -> (w1210)
                                n814 = And(x=w1212, y=w1210) -> (x .and. y?=w1207:bool)
                                n815 = case shown="True" w1207 {
                                tunnel: w1208 -> [_ w1231]
                                frame False {
                                }
                                frame True {
                                n816 = Get Date/Time In Seconds() -> (seconds since 1Jan1904=w1217:timestamp)
                                n817 = To Double Precision Float(number=w1217) -> (double precision float=w1216:dbl)
                                n818 = global read "G_rio.vi" "LCM_RMC_T"() -> (w1232:T13)
                                n819 = Unbundle By Name(w1232) -> ("hash"=w1228:i64)
                                n820 = Multiply(x=w1216, y=1000000.0) -> (x*y=w1214:dbl)
                                n821 = Array To Cluster(array=w1231) -> (cluster=w1230:T14)
                                n822 = To Quad Integer(1:w1214) -> (0:w1213:i64)
                                n823 = call "hash.vi"("input"=w1228) -> ("output"=w1227:i64)  [unwired: 10 in]
                                n824 = Unbundle(w1230) -> ("vel[0]"=w1222:dbl, "vel[2]"=w1221:dbl, "vel[4]"=w1220:dbl, "vel[5]"=w1219:dbl, "vel[6]"=w1218:dbl)  [unwired: 2 out]
                                n825 = Bundle(cluster=w1232, "hash"=w1227, "sys time"=w1213, "time"=w1222, "speed"=w1221, "heading"=w1220, "lat"=w1219, "lon"=w1218) -> (w1223:T13)
                                n826 = Flatten To String(anything=w1223, prepend array or string size? (T)=FALSE) -> (data string=w1225:string)  [unwired: 2 in, 2 out]
                                n827 = global read "G_rio.vi" "LCM"() -> (w1224:T3)
                                n828 = call "LCM_send.vi"("DATA"=w1225, "ID"="RMC_1", "LCM"=w1224) -> ()  [unwired: 7 in, 2 out]
                                }
                                }
                                }
                                }
                                n829 = global write "G_rio.vi" "dgps_vel"(w1205) -> ()
                                }
                                }
                              }
                              frame True {
                              }
                            }
                          }
                        }
                      }
                    }
                  }
                  frame True {
                    n830 = xnode "Invoke Method"("FPGA VI Reference In"=w1233, "Number of Elements"=u32 1, "Timeout (ms)"=5) -> ("FPGA VI Reference Out"=w1237:refnum<k20>, "error out"=w1238:errorcluster, "Elements Remaining"=w1239:u32)  [unwired: 1 in, 1 out]
                    n831 = xnode "Invoke Method"("FPGA VI Reference In"=w1237, "error in"=w1238, "Number of Elements"=w1239, "Timeout (ms)"=5) -> ()  [unwired: 4 out]
                  }
                }
              }
            }
          }
        }
        frame Disabled {
          n832 = while {
            stop <- FALSE stop-if-true
            n833 = flat-sequence {
              frame #0 {
                n834 = Wait Until Next ms Multiple(millisecond multiple=u32 100) -> (millisecond timer value=w1241:u32)
                n835 = flat-sequence {
                  tunnel: w1241 -> [w1244]
                  frame #0 {
                    n836 = feedback #20(w1244) -> (w1245:u32)
                    n837 = feedback-in #20(w1244) -> ()
                    n838 = Subtract(x=w1244, y=w1245) -> (x-y=→"GPS_novatel_time":u32)
                  }
                }
              }
              frame #1 {
                n839 = local read item#-1() -> (w1248)
                n840 = xnode "Read/Write Control"("FPGA VI Reference In"=w1248) -> ("FPGA VI Reference Out"=w1247:refnum<k20>, "error out"=w1246:errorcluster)  [unwired: 1 in, 1 out]
                n841 = flat-sequence {
                  tunnel: w1247 -> [w1259]
                  tunnel: w1246 -> [w1258]
                  frame #0 {
                    n842 = xnode "Invoke Method"("FPGA VI Reference In"=w1259, "error in"=w1258, "Number of Elements"=u32 0, "Timeout (ms)"=10) -> ("FPGA VI Reference Out"=w1257:refnum<k20>, "error out"=w1256:errorcluster, "Elements Remaining"=w1255:u32)  [unwired: 1 out]
                    n843 = xnode "Invoke Method"("FPGA VI Reference In"=w1257, "error in"=w1256, "Number of Elements"=w1255) -> ("Data"=w1249:u8[])  [unwired: 1 in, 3 out]
                    n844 = local read "rest"() -> (w1251:u8[])
                    n845 = Build Array (concatenate)(w1251, w1249) -> (w1250:u8[])
                    n846 = Empty Array?(array=w1250) -> (empty?=w1252:bool)
                    n847 = case shown="False" w1252 {
                      tunnel: w1250 -> [w1262 _]
                      frame False {
                        n848 = for {
                          N: 2 -> [_]
                          shift-right: [w1266] -> w1260
                          shift-left: w1262 -> [w1264]
                          n849 = for {
                            tunnel: w1264 -> [w1377]
                            tunnel: u8[] [170, 68, 18, 28] -> [w1375] mode=indexing
                            shift-right: [w1374] -> _
                            shift-left: 0 ("start index (0)") -> [w1376]
                            tunnel: [w1374] -> w1273 mode=indexing
                            n850 = Search 1D Array(1D array=w1377, element=w1375, start index (0)=w1376) -> (index of element=w1374:i32)
                          }
                          n851 = Index Array(array=w1273, index #1=3 ("index"), index #2=0 ("index")) -> (element #1=w1270:i32, element #2=w1263:i32)
                          n852 = Subtract(x=w1270, y=w1263) -> (x-y=w1269:i32)
                          n853 = Array Subset(array=w1264, index=w1263) -> (w1265:u8[])  [unwired: 1 in]
                          n854 = Equal?(x=3, y=w1269) -> (x = y?=w1267:bool)
                          n855 = case shown="True" w1267 {
                            tunnel: w1265 -> [w1279 w1288]
                            tunnel: [w1278 w1285] -> w1266
                            tunnel: w1263 -> [w1277 _]
                            frame False {
                              n856 = Greater Or Equal To 0?(x=w1277) -> (x >= 0?=w1276:bool)
                              n857 = case shown="False" w1276 {
                                tunnel: w1279 -> [w1280 w1283]
                                tunnel: [w1280 w1281] -> w1278
                                frame False {
                                }
                                frame True {
                                n858 = Array Subset(array=w1283, index=1 ("length")) -> (w1281:u8[])  [unwired: 1 in]
                                }
                              }
                            }
                            frame True {
                              w1284 = 4 ("index")
                              n859 = Array Size(array=w1288) -> (size(s)=w1290:i32)
                              n860 = Add(x=w1284, y=4) -> (x+y=w1297:i32)
                              n861 = Increment(x=w1284) -> (x+1=w1300:i32)
                              n862 = Increment(x=w1297) -> (x+1=w1298:i32)
                              n863 = Index Array(array=w1288, index #1=w1300, index #2=w1284, index #3=w1298, index #4=w1297) -> (element #1=w1296:u8, element #2=w1295:u8, element #3=w1294:u8, element #4=w1293:u8)
                              n864 = Join Numbers(hi=w1296, lo=w1295) -> ((hi.lo)=w1286:u16)
                              n865 = Join Numbers(hi=w1294, lo=w1293) -> ((hi.lo)=w1292:u16)
                              n866 = Add(x=w1292, y=u16 32) -> (x+y=w1287:u16)
                              n867 = Greater Or Equal?(x=w1290, y=w1287) -> (x >= y?=w1289:bool)
                              n868 = case shown="True" w1289 {
                                tunnel: w1288 -> [_ w1306]
                                tunnel: w1287 -> [_ w1305]
                                tunnel: w1286 -> [_ w1302]
                                tunnel: [_ w1301] -> w1285
                                frame False {
                                }
                                frame True {
                                n869 = Delete From Array(array=w1306, length=w1305, index=0) -> (deleted portion=w1303:u8[], array with subset deleted=w1301:u8[])
                                n870 = case shown="99" w1302 {
                                tunnel: w1303 -> [_ w1309 w1347]
                                frame 0, Default {
                                }
                                frame 42 {
                                n871 = local read "ecef ref"() -> (w1308:dbl[])
                                n872 = call "novatel_bestpos.vi"("ecef ref"=w1308, "gps_data"=w1309) -> ("LCC"=w1307:dbl[])  [unwired: 9 in]
                                n873 = flat-sequence {
                                tunnel: w1307 -> [w1312]
                                frame #0 {
                                n874 = Index Array(array=w1312, index=1) -> (element=w1315:dbl)
                                n875 = Not Equal To 0?(x=w1315) -> (x != 0?=w1311:bool)
                                n876 = local read item#-1() -> (w1314)
                                n877 = And(x=w1311, y=w1314) -> (x .and. y?=w1310:bool)
                                n878 = case shown="True" w1310 {
                                tunnel: w1312 -> [_ w1335]
                                frame False {
                                }
                                frame True {
                                n879 = Get Date/Time In Seconds() -> (seconds since 1Jan1904=w1320:timestamp)
                                n880 = To Double Precision Float(number=w1320) -> (double precision float=w1319:dbl)
                                n881 = global read "G_rio.vi" "LCM_GGA_T"() -> (w1344:T11)
                                n882 = Array To Cluster(array=w1335) -> (cluster=w1343:T12)
                                n883 = Unbundle By Name(w1344) -> ("hash"=w1340:i64)
                                n884 = Multiply(x=w1319, y=1000000.0) -> (x*y=w1317:dbl)
                                n885 = Unbundle(w1343) -> ("LCC[0]"=w1345:dbl, "LCC[2]"=w1334:dbl, "LCC[3]"=w1333:dbl, "LCC[4]"=w1332:dbl, "LCC[6]"=w1331:dbl, "LCC[7]"=w1329:dbl, "LCC[8]"=w1327:dbl, "LCC[9]"=w1325:dbl, "LCC[12]"=w1324:dbl, "LCC[13]"=w1323:dbl, "LCC[14]"=w1322:dbl)  [unwired: 4 out]
                                n886 = To Quad Integer(1:w1317) -> (0:w1316:i64)
                                n887 = To Long Integer(number=w1331) -> (32bit integer=w1330:i32)
                                n888 = To Long Integer(number=w1329) -> (32bit integer=w1328:i32)
                                n889 = To Long Integer(number=w1327) -> (32bit integer=w1326:i32)
                                n890 = call "hash.vi"("input"=w1340) -> ("output"=w1339:i64)  [unwired: 10 in]
                                n891 = local read "map"() -> (w1321:i32)
                                n892 = Bundle(cluster=w1344, "hash"=w1339, "sys time"=w1316, "time"=w1345, "x"=w1334, "y"=w1333, "h"=w1332, "numSV"=w1330, "postype"=w1328, "lag"=w1326, "hordev"=w1325, "lat"=w1324, "lon"=w1323, "hgt"=w1322, "map_idx"=w1321) -> (w1341:T11)
                                n893 = Flatten To String(anything=w1341, prepend array or string size? (T)=FALSE) -> (data string=w1337:string)  [unwired: 2 in, 2 out]
                                n894 = global read "G_rio.vi" "LCM"() -> (w1336:T3)
                                n895 = call "LCM_send.vi"("DATA"=w1337, "ID"="GGA_DGPS", "LCM"=w1336) -> ()  [unwired: 7 in, 2 out]
                                }
                                }
                                }
                                }
                                n896 = global write "G_rio.vi" "dgps_pos"(w1307) -> ()
                                }
                                frame 99 {
                                n897 = call "novatel_bestvel.vi"("gps_data"=w1347) -> ("vel"=w1346:dbl[])  [unwired: 10 in]
                                n898 = flat-sequence {
                                tunnel: w1346 -> [w1350]
                                frame #0 {
                                n899 = Index Array(array=w1350, index=1) -> (element=w1352:dbl)
                                n900 = Not Equal To 0?(x=w1352) -> (x != 0?=w1353:bool)
                                n901 = local read item#-1() -> (w1348)
                                n902 = And(x=w1353, y=w1348) -> (x .and. y?=w1349:bool)
                                n903 = case shown="True" w1349 {
                                tunnel: w1350 -> [_ w1372]
                                frame False {
                                }
                                frame True {
                                n904 = Get Date/Time In Seconds() -> (seconds since 1Jan1904=w1358:timestamp)
                                n905 = To Double Precision Float(number=w1358) -> (double precision float=w1357:dbl)
                                n906 = global read "G_rio.vi" "LCM_RMC_T"() -> (w1373:T13)
                                n907 = Unbundle By Name(w1373) -> ("hash"=w1369:i64)
                                n908 = Multiply(x=w1357, y=1000000.0) -> (x*y=w1355:dbl)
                                n909 = Array To Cluster(array=w1372) -> (cluster=w1371:T14)
                                n910 = To Quad Integer(1:w1355) -> (0:w1354:i64)
                                n911 = call "hash.vi"("input"=w1369) -> ("output"=w1368:i64)  [unwired: 10 in]
                                n912 = Unbundle(w1371) -> ("vel[0]"=w1363:dbl, "vel[2]"=w1362:dbl, "vel[4]"=w1361:dbl, "vel[5]"=w1360:dbl, "vel[6]"=w1359:dbl)  [unwired: 2 out]
                                n913 = Bundle(cluster=w1373, "hash"=w1368, "sys time"=w1354, "time"=w1363, "speed"=w1362, "heading"=w1361, "lat"=w1360, "lon"=w1359) -> (w1364:T13)
                                n914 = Flatten To String(anything=w1364, prepend array or string size? (T)=FALSE) -> (data string=w1366:string)  [unwired: 2 in, 2 out]
                                n915 = global read "G_rio.vi" "LCM"() -> (w1365:T3)
                                n916 = call "LCM_send.vi"("DATA"=w1366, "ID"="RMC_DGPS", "LCM"=w1365) -> ()  [unwired: 7 in, 2 out]
                                }
                                }
                                }
                                }
                                n917 = global write "G_rio.vi" "dgps_vel"(w1346) -> ()
                                }
                                }
                                }
                              }
                            }
                          }
                        }
                        "rest" <- w1260
                      }
                      frame True {
                      }
                    }
                  }
                }
              }
            }
          }
        }
        frame Enabled {
          n918 = while {
            stop <- FALSE stop-if-true
            n919 = flat-sequence {
              tunnel: [w1380] -> w1378
              tunnel: w1378 -> [w1385]
              frame #0 {
                n920 = Wait Until Next ms Multiple(millisecond multiple=u32 50) -> (millisecond timer value=w1383:u32)
                n921 = feedback #21(w1383) -> (w1382:u32)
                n922 = feedback-in #21(w1383) -> ()
                n923 = Subtract(x=w1383, y=w1382) -> (x-y=→"GPS_time 100":u32)
                n924 = local read "ublox"() -> (w1380:bool)
              }
              frame #1 {
                n925 = case shown="True" w1385 {
                  frame False {
                    n926 = First Call?() -> (First Call?: T/F=w1386:bool)
                    n927 = case shown="False" w1386 {
                      frame False {
                        n928 = for {
                          N: 5 -> [_]
                          stop <- w1392 stop-if-true
                          n929 = local read "novatel"() -> (w1388:refnum<visa-resource-name>)
                          n930 = VISA Read(VISA resource name=w1388, byte count=u32 150) -> (read buffer=w1394:string, error out=w1393:errorcluster)  [unwired: 1 in, 2 out]
                          n931 = local read "ecef ref"() -> (w1395:dbl[])
                          n932 = Unbundle By Name(w1393) -> ("code"=w1391:i32, "status"=w1392:bool)
                          n933 = call "nmea.vi"("ecef ref"=w1395, "NMEA"=w1394) -> ("output"=w1397:dbl[], "type"=w1396:u32)  [unwired: 8 in]
                          n934 = case shown="2" w1396 {
                            tunnel: w1397 -> [_ w1406 w1439]
                            frame 0, Default {
                            }
                            frame 1 {
                              n935 = global write "G_rio.vi" "dgps_pos"(w1406) -> ()
                              n936 = Index Array(array=w1406, index=1) -> (element=w1408:dbl)
                              n937 = Not Equal To 0?(x=w1408) -> (x != 0?=w1405:bool)
                              n938 = case shown="True" w1405 {
                                tunnel: w1406 -> [_ w1428]
                                frame False {
                                }
                                frame True {
                                n939 = Get Date/Time In Seconds() -> (seconds since 1Jan1904=w1413:timestamp)
                                n940 = To Double Precision Float(number=w1413) -> (double precision float=w1412:dbl)
                                n941 = global read "G_rio.vi" "LCM_GGA_T"() -> (w1437:T11)
                                n942 = Array To Cluster(array=w1428) -> (cluster=w1436:T15)
                                n943 = Unbundle By Name(w1437) -> ("hash"=w1433:i64)
                                n944 = Multiply(x=w1412, y=1000000.0) -> (x*y=w1410:dbl)
                                n945 = Unbundle(w1436) -> ("output[0]"=w1438:dbl, "output[2]"=w1427:dbl, "output[3]"=w1426:dbl, "output[4]"=w1425:dbl, "output[6]"=w1424:dbl, "output[7]"=w1422:dbl, "output[8]"=w1420:dbl, "output[9]"=w1418:dbl, "output[12]"=w1417:dbl, "output[13]"=w1416:dbl, "output[14]"=w1415:dbl)  [unwired: 4 out]
                                n946 = call "hash.vi"("input"=w1433) -> ("output"=w1432:i64)  [unwired: 10 in]
                                n947 = To Quad Integer(1:w1410) -> (0:w1409:i64)
                                n948 = To Long Integer(number=w1424) -> (32bit integer=w1423:i32)
                                n949 = To Long Integer(number=w1422) -> (32bit integer=w1421:i32)
                                n950 = To Long Integer(number=w1420) -> (32bit integer=w1419:i32)
                                n951 = local read "map"() -> (w1414:i32)
                                n952 = Bundle(cluster=w1437, "hash"=w1432, "sys time"=w1409, "time"=w1438, "x"=w1427, "y"=w1426, "h"=w1425, "numSV"=w1423, "postype"=w1421, "lag"=w1419, "hordev"=w1418, "lat"=w1417, "lon"=w1416, "hgt"=w1415, "map_idx"=w1414) -> (w1434:T11)
                                n953 = Flatten To String(anything=w1434, prepend array or string size? (T)=FALSE) -> (data string=w1430:string)  [unwired: 2 in, 2 out]
                                n954 = global read "G_rio.vi" "LCM"() -> (w1429:T3)
                                n955 = call "LCM_send.vi"("DATA"=w1430, "ID"="GGA_1", "LCM"=w1429) -> ()  [unwired: 7 in, 2 out]
                                }
                              }
                            }
                            frame 2 {
                              n956 = flat-sequence {
                                tunnel: w1439 -> [w1441]
                                frame #0 {
                                n957 = Index Array(array=w1441, index=1) -> (element=w1443:dbl)
                                n958 = Not Equal To 0?(x=w1443) -> (x != 0?=w1440:bool)
                                n959 = case shown="True" w1440 {
                                tunnel: w1441 -> [_ w1462]
                                frame False {
                                }
                                frame True {
                                n960 = Get Date/Time In Seconds() -> (seconds since 1Jan1904=w1448:timestamp)
                                n961 = To Double Precision Float(number=w1448) -> (double precision float=w1447:dbl)
                                n962 = global read "G_rio.vi" "LCM_RMC_T"() -> (w1463:T13)
                                n963 = Unbundle By Name(w1463) -> ("hash"=w1459:i64)
                                n964 = Multiply(x=w1447, y=1000000.0) -> (x*y=w1445:dbl)
                                n965 = Array To Cluster(array=w1462) -> (cluster=w1461:T16)
                                n966 = To Quad Integer(1:w1445) -> (0:w1444:i64)
                                n967 = call "hash.vi"("input"=w1459) -> ("output"=w1458:i64)  [unwired: 10 in]
                                n968 = Unbundle(w1461) -> ("output[0]"=w1453:dbl, "output[2]"=w1452:dbl, "output[4]"=w1451:dbl, "output[5]"=w1450:dbl, "output[6]"=w1449:dbl)  [unwired: 2 out]
                                n969 = Bundle(cluster=w1463, "hash"=w1458, "sys time"=w1444, "time"=w1453, "speed"=w1452, "heading"=w1451, "lat"=w1450, "lon"=w1449) -> (w1454:T13)
                                n970 = Flatten To String(anything=w1454, prepend array or string size? (T)=FALSE) -> (data string=w1456:string)  [unwired: 2 in, 2 out]
                                n971 = global read "G_rio.vi" "LCM"() -> (w1455:T3)
                                n972 = call "LCM_send.vi"("DATA"=w1456, "ID"="RMC_1", "LCM"=w1455) -> ()  [unwired: 7 in, 2 out]
                                }
                                }
                                }
                              }
                              n973 = global write "G_rio.vi" "dgps_vel"(w1439) -> ()
                            }
                          }
                          n974 = case shown="-1073807194" w1391 {
                            tunnel: w1388 -> [_ _ w1401]
                            tunnel: [TRUE _ _] -> w1390
                            frame 0, Default {
                            }
                            frame -1073807343 {
                            }
                            frame -1073807194 {
                              n975 = VISA Close(VISA resource name=w1401) -> (error out=w1402:errorcluster)  [unwired: 1 in]
                              n976 = call-poly "VISA Configure Serial Port"("VISA resource name"=refnum<visa-resource-name> "ASRL1::INSTR", "timeout (10sec)"=u32 10, "baud rate (9600)"=u32 115200, "error in (no error)"=w1402) -> ("VISA resource name out"=w1400:refnum<visa-resource-name>)  [unwired: 10 in, 1 out]
                              n977 = local write "novatel"(w1400) -> ()
                            }
                          }
                          n978 = global write "G_rio.vi" "A_GPS"(w1390) -> ()
                          n979 = global write "G_rio.vi" "A_GPS 2"(w1390) -> ()
                        }
                      }
                      frame True {
                        n980 = global write "G_rio.vi" "R"(T10 [[5.0, 0.0, 0.0], [0.0, 5.0, 0.0], [0.0, 0.0, 0.5]] ("R")) -> ()
                      }
                    }
                  }
                  frame True {
                    n981 = First Call?() -> (First Call?: T/F=w1465:bool)
                    n982 = case shown="False" w1465 {
                      frame False {
                        n983 = for {
                          N: 5 -> [_]
                          stop <- w1547 stop-if-true
                          n984 = local read "gps2"() -> (w1548:refnum<visa-resource-name>)
                          n985 = VISA Read(VISA resource name=w1548, byte count=u32 100) -> (VISA resource name out=w1545:refnum<visa-resource-name>, read buffer=w1554:string, error out=w1549:errorcluster)  [unwired: 1 in, 1 out]
                          n986 = local read "ecef ref"() -> (w1553:dbl[])
                          n987 = Unbundle By Name(w1549) -> ("code"=w1546:i32, "status"=w1547:bool)
                          n988 = call "nmea.vi"("ecef ref"=w1553, "NMEA"=w1554) -> ("output"=w1551:dbl[], "type"=w1552:u32)  [unwired: 8 in]
                          n989 = case shown="2" w1552 {
                            tunnel: w1551 -> [_ w1565 w1601]
                            frame 0, Default {
                            }
                            frame 1 {
                              n990 = global write "G_rio.vi" "gps_pos 2"(w1565) -> ()
                              n991 = Index Array(array=w1565, index=1) -> (element=w1566:dbl)
                              n992 = Not Equal To 0?(x=w1566) -> (x != 0?=w1564:bool)
                              n993 = case shown="True" w1564 {
                                tunnel: w1565 -> [_ w1587]
                                frame False {
                                }
                                frame True {
                                n994 = Get Date/Time In Seconds() -> (seconds since 1Jan1904=w1572:timestamp)
                                n995 = To Double Precision Float(number=w1572) -> (double precision float=w1571:dbl)
                                n996 = global read "G_rio.vi" "LCM_GGA_T"() -> (w1596:T11)
                                n997 = Array To Cluster(array=w1587) -> (cluster=w1595:T15)
                                n998 = Unbundle By Name(w1596) -> ("hash"=w1592:i64)
                                n999 = Multiply(x=w1571, y=1000000.0) -> (x*y=w1569:dbl)
                                n1000 = Unbundle(w1595) -> ("output[0]"=w1597:dbl, "output[2]"=w1586:dbl, "output[3]"=w1585:dbl, "output[4]"=w1584:dbl, "output[6]"=w1583:dbl, "output[7]"=w1581:dbl, "output[8]"=w1579:dbl, "output[9]"=w1577:dbl, "output[12]"=w1576:dbl, "output[13]"=w1575:dbl, "output[14]"=w1574:dbl)  [unwired: 4 out]
                                n1001 = call "hash.vi"("input"=w1592) -> ("output"=w1591:i64)  [unwired: 10 in]
                                n1002 = To Quad Integer(1:w1569) -> (0:w1568:i64)
                                n1003 = To Long Integer(number=w1583) -> (32bit integer=w1582:i32)
                                n1004 = To Long Integer(number=w1581) -> (32bit integer=w1580:i32)
                                n1005 = To Long Integer(number=w1579) -> (32bit integer=w1578:i32)
                                n1006 = local read "map"() -> (w1573:i32)
                                n1007 = Bundle(cluster=w1596, "hash"=w1591, "sys time"=w1568, "time"=w1597, "x"=w1586, "y"=w1585, "h"=w1584, "numSV"=w1582, "postype"=w1580, "lag"=w1578, "hordev"=w1577, "lat"=w1576, "lon"=w1575, "hgt"=w1574, "map_idx"=w1573) -> (w1593:T11)
                                n1008 = Flatten To String(anything=w1593, prepend array or string size? (T)=FALSE) -> (data string=w1589:string)  [unwired: 2 in, 2 out]
                                n1009 = global read "G_rio.vi" "LCM"() -> (w1588:T3)
                                n1010 = call "LCM_send.vi"("DATA"=w1589, "ID"="GGA_2", "LCM"=w1588) -> ()  [unwired: 7 in, 2 out]
                                }
                              }
                            }
                            frame 2 {
                              n1011 = global write "G_rio.vi" "gps_vel 2"(w1601) -> ()
                              n1012 = Index Array(array=w1601, index=1) -> (element=w1599:dbl)
                              n1013 = Not Equal To 0?(x=w1599) -> (x != 0?=w1598:bool)
                              n1014 = case shown="True" w1598 {
                                tunnel: w1601 -> [_ w1612]
                                frame False {
                                }
                                frame True {
                                n1015 = Get Date/Time In Seconds() -> (seconds since 1Jan1904=w1606:timestamp)
                                n1016 = To Double Precision Float(number=w1606) -> (double precision float=w1605:dbl)
                                n1017 = global read "G_rio.vi" "LCM_RMC_T"() -> (w1613:T13)
                                n1018 = Unbundle By Name(w1613) -> ("hash"=w1617:i64)
                                n1019 = Multiply(x=w1605, y=1000000.0) -> (x*y=w1603:dbl)
                                n1020 = Array To Cluster(array=w1612) -> (cluster=w1614:T16)
                                n1021 = call "hash.vi"("input"=w1617) -> ("output"=w1618:i64)  [unwired: 10 in]
                                n1022 = To Quad Integer(1:w1603) -> (0:w1602:i64)
                                n1023 = Unbundle(w1614) -> ("output[0]"=w1611:dbl, "output[2]"=w1610:dbl, "output[4]"=w1609:dbl, "output[5]"=w1608:dbl, "output[6]"=w1607:dbl)  [unwired: 2 out]
                                n1024 = Bundle(cluster=w1613, "hash"=w1618, "sys time"=w1602, "time"=w1611, "speed"=w1610, "heading"=w1609, "lat"=w1608, "lon"=w1607) -> (w1616:T13)
                                n1025 = Flatten To String(anything=w1616, prepend array or string size? (T)=FALSE) -> (data string=w1620:string)  [unwired: 2 in, 2 out]
                                n1026 = global read "G_rio.vi" "LCM"() -> (w1621:T3)
                                n1027 = call "LCM_send.vi"("DATA"=w1620, "ID"="RMC_2", "LCM"=w1621) -> ()  [unwired: 7 in, 2 out]
                                }
                              }
                            }
                          }
                          n1028 = case shown="0, Default" w1546 {
                            tunnel: w1545 -> [_ _ w1559]
                            tunnel: [TRUE FALSE FALSE] -> w1544
                            frame 0, Default {
                            }
                            frame -1073807343 {
                            }
                            frame -1073807194 {
                              n1029 = VISA Close(VISA resource name=w1559) -> (error out=w1560:errorcluster)  [unwired: 1 in]
                              n1030 = call-poly "VISA Configure Serial Port"("VISA resource name"=refnum<visa-resource-name> "USB0::0x1546::0x01A6::NI-VISA-0::1::RAW", "timeout (10sec)"=u32 1, "baud rate (9600)"=u32 115200, "error in (no error)"=w1560) -> ("VISA resource name out"=w1558:refnum<visa-resource-name>)  [unwired: 10 in, 1 out]
                              n1031 = local write "gps2"(w1558) -> ()
                            }
                          }
                          n1032 = global write "G_rio.vi" "A_GPS 2"(w1544) -> ()
                        }
                        n1033 = for {
                          N: 5 -> [_]
                          stop <- w1471 stop-if-true
                          n1034 = local read "gps1"() -> (w1470:refnum<visa-resource-name>)
                          n1035 = VISA Read(VISA resource name=w1470, byte count=u32 100) -> (read buffer=w1474:string, error out=w1472:errorcluster)  [unwired: 1 in, 2 out]
                          n1036 = local read "ecef ref"() -> (w1475:dbl[])
                          n1037 = Unbundle By Name(w1472) -> ("code"=w1469:i32, "status"=w1471:bool)
                          n1038 = call "nmea.vi"("ecef ref"=w1475, "NMEA"=w1474) -> ("output"=w1477:dbl[], "type"=w1476:u32)  [unwired: 8 in]
                          n1039 = case shown="2" w1476 {
                            tunnel: w1477 -> [_ w1486 w1519]
                            frame 0, Default {
                            }
                            frame 1 {
                              n1040 = global write "G_rio.vi" "gps_pos 1"(w1486) -> ()
                              n1041 = Index Array(array=w1486, index=1) -> (element=w1488:dbl)
                              n1042 = Not Equal To 0?(x=w1488) -> (x != 0?=w1485:bool)
                              n1043 = case shown="True" w1485 {
                                tunnel: w1486 -> [_ w1508]
                                frame False {
                                }
                                frame True {
                                n1044 = Get Date/Time In Seconds() -> (seconds since 1Jan1904=w1493:timestamp)
                                n1045 = To Double Precision Float(number=w1493) -> (double precision float=w1492:dbl)
                                n1046 = global read "G_rio.vi" "LCM_GGA_T"() -> (w1517:T11)
                                n1047 = Array To Cluster(array=w1508) -> (cluster=w1516:T15)
                                n1048 = Unbundle By Name(w1517) -> ("hash"=w1513:i64)
                                n1049 = Multiply(x=w1492, y=1000000.0) -> (x*y=w1490:dbl)
                                n1050 = Unbundle(w1516) -> ("output[0]"=w1518:dbl, "output[2]"=w1507:dbl, "output[3]"=w1506:dbl, "output[4]"=w1505:dbl, "output[6]"=w1504:dbl, "output[7]"=w1502:dbl, "output[8]"=w1500:dbl, "output[9]"=w1498:dbl, "output[12]"=w1497:dbl, "output[13]"=w1496:dbl, "output[14]"=w1495:dbl)  [unwired: 4 out]
                                n1051 = call "hash.vi"("input"=w1513) -> ("output"=w1512:i64)  [unwired: 10 in]
                                n1052 = To Quad Integer(1:w1490) -> (0:w1489:i64)
                                n1053 = To Long Integer(number=w1504) -> (32bit integer=w1503:i32)
                                n1054 = To Long Integer(number=w1502) -> (32bit integer=w1501:i32)
                                n1055 = To Long Integer(number=w1500) -> (32bit integer=w1499:i32)
                                n1056 = local read "map"() -> (w1494:i32)
                                n1057 = Bundle(cluster=w1517, "hash"=w1512, "sys time"=w1489, "time"=w1518, "x"=w1507, "y"=w1506, "h"=w1505, "numSV"=w1503, "postype"=w1501, "lag"=w1499, "hordev"=w1498, "lat"=w1497, "lon"=w1496, "hgt"=w1495, "map_idx"=w1494) -> (w1514:T11)
                                n1058 = Flatten To String(anything=w1514, prepend array or string size? (T)=FALSE) -> (data string=w1510:string)  [unwired: 2 in, 2 out]
                                n1059 = global read "G_rio.vi" "LCM"() -> (w1509:T3)
                                n1060 = call "LCM_send.vi"("DATA"=w1510, "ID"="GGA_1", "LCM"=w1509) -> ()  [unwired: 7 in, 2 out]
                                }
                              }
                            }
                            frame 2 {
                              n1061 = flat-sequence {
                                tunnel: w1519 -> [w1521]
                                frame #0 {
                                n1062 = Index Array(array=w1521, index=1) -> (element=w1523:dbl)
                                n1063 = Not Equal To 0?(x=w1523) -> (x != 0?=w1520:bool)
                                n1064 = case shown="True" w1520 {
                                tunnel: w1521 -> [_ w1542]
                                frame False {
                                }
                                frame True {
                                n1065 = Get Date/Time In Seconds() -> (seconds since 1Jan1904=w1528:timestamp)
                                n1066 = To Double Precision Float(number=w1528) -> (double precision float=w1527:dbl)
                                n1067 = global read "G_rio.vi" "LCM_RMC_T"() -> (w1543:T13)
                                n1068 = Unbundle By Name(w1543) -> ("hash"=w1539:i64)
                                n1069 = Multiply(x=w1527, y=1000000.0) -> (x*y=w1525:dbl)
                                n1070 = Array To Cluster(array=w1542) -> (cluster=w1541:T16)
                                n1071 = call "hash.vi"("input"=w1539) -> ("output"=w1538:i64)  [unwired: 10 in]
                                n1072 = To Quad Integer(1:w1525) -> (0:w1524:i64)
                                n1073 = Unbundle(w1541) -> ("output[0]"=w1533:dbl, "output[2]"=w1532:dbl, "output[4]"=w1531:dbl, "output[5]"=w1530:dbl, "output[6]"=w1529:dbl)  [unwired: 2 out]
                                n1074 = Bundle(cluster=w1543, "hash"=w1538, "sys time"=w1524, "time"=w1533, "speed"=w1532, "heading"=w1531, "lat"=w1530, "lon"=w1529) -> (w1534:T13)
                                n1075 = Flatten To String(anything=w1534, prepend array or string size? (T)=FALSE) -> (data string=w1536:string)  [unwired: 2 in, 2 out]
                                n1076 = global read "G_rio.vi" "LCM"() -> (w1535:T3)
                                n1077 = call "LCM_send.vi"("DATA"=w1536, "ID"="RMC_1", "LCM"=w1535) -> ()  [unwired: 7 in, 2 out]
                                }
                                }
                                }
                              }
                              n1078 = global write "G_rio.vi" "gps_vel 1"(w1519) -> ()
                            }
                          }
                          n1079 = case shown="-1073807343" w1469 {
                            tunnel: w1470 -> [_ _ w1480]
                            tunnel: [TRUE _ _] -> w1468
                            frame 0, Default {
                            }
                            frame -1073807343 {
                            }
                            frame -1073807194 {
                              n1080 = VISA Close(VISA resource name=w1480) -> (error out=w1481:errorcluster)  [unwired: 1 in]
                              n1081 = call-poly "VISA Configure Serial Port"("VISA resource name"=refnum<visa-resource-name> "USB0::0x1546::0x01A6::NI-VISA-1::1::RAW", "timeout (10sec)"=u32 1, "baud rate (9600)"=u32 115200, "error in (no error)"=w1481) -> ("VISA resource name out"=w1479:refnum<visa-resource-name>)  [unwired: 10 in, 1 out]
                              n1082 = local write "gps1"(w1479) -> ()
                            }
                          }
                          n1083 = global write "G_rio.vi" "A_GPS"(w1468) -> ()
                        }
                      }
                      frame True {
                        n1084 = global write "G_rio.vi" "R"(T10 [[10.0, 0.0, 0.0], [0.0, 10.0, 0.0], [0.0, 0.0, 0.5]] ("R")) -> ()
                      }
                    }
                  }
                }
              }
            }
          }
        }
      }
      n1085 = while {
        shift-right: [w1628] -> _
        shift-left: w1106 -> [w1627]
        stop <- FALSE stop-if-true
        n1086 = flat-sequence {
          tunnel: [w1637] -> w1624
          tunnel: w1627 -> [w1637]
          tunnel: w1624 -> [w1643]
          tunnel: [w1644] -> w1625
          tunnel: [w1642] -> w1623
          tunnel: [w2343] -> w1628
          tunnel: w1625 -> [w2344]
          tunnel: w1623 -> [w2343]
          frame #0 {
            n1087 = global read "G_rio.vi" "time"() -> (w1630:u32)
            n1088 = Wait Until Next ms Multiple(millisecond multiple=u32 10) -> (millisecond timer value=w1635:u32)
            n1089 = feedback #22(w1630) -> (w1629:u32)
            n1090 = feedback-in #22(w1630) -> ()
            n1091 = Subtract(x=w1630, y=w1629) -> (x-y=w1631:u32)
            n1092 = flat-sequence {
              tunnel: w1635 -> [w1640]
              frame #0 {
                n1093 = feedback #23(w1640) -> (w1641:u32)
                n1094 = feedback-in #23(w1640) -> ()
                n1095 = Subtract(x=w1640, y=w1641) -> (x-y=w1639:u32)
                n1096 = To Long Integer(number=w1639) -> (32bit integer=→"Pos_time 10":i32)
              }
            }
            n1097 = To Double Precision Float(number=w1631) -> (double precision float=w1632:dbl)
            n1098 = Multiply(x=w1632, y=1e-07) -> (x*y=→"dt":dbl)
          }
          frame #1 {
            n1099 = disable-structure shown="Enabled" {
              disable-tunnel: [w1645 w2050] -> w1644
              disable-tunnel: w1643 -> [w1646 w2072]
              disable-tunnel: [w1645 w2059] -> w1642
              frame Enabled {
                n1100 = flat-sequence {
                  tunnel: w1646 -> [w1659]
                  tunnel: [w1659] -> w1647
                  tunnel: [w1781] -> w1645
                  tunnel: w1647 -> [w1782]
                  frame #0 {
                    n1101 = case shown="True" "ublox" {
                      tunnel: [w1753 w1771] -> w1648
                      tunnel: [w1752 w1772] -> w1650
                      frame True {
                        n1102 = global read "G_rio.vi" "gps_pos 1"() -> (w1768:dbl[])
                        n1103 = global read "G_rio.vi" "gps_pos 2"() -> (w1755:dbl[])
                        n1104 = Add(x=w1768, y=w1755) -> (x+y=w1770:dbl[])
                        n1105 = Index Array(array=w1768, index #1=0 ("index")) -> (element #1=w1767:dbl, element #2=w1766:dbl)  [unwired: 1 in]
                        n1106 = Index Array(array=w1755, index #1=0 ("index")) -> (element #1=w1756:dbl, element #2=w1757:dbl)  [unwired: 1 in]
                        n1107 = feedback #24(w1767) -> (w1765:dbl)
                        n1108 = feedback-in #24(w1767) -> ()
                        n1109 = feedback #25(w1756) -> (w1758:dbl)
                        n1110 = feedback-in #25(w1756) -> ()
                        n1111 = Not Equal?(x=w1767, y=w1765) -> (x != y?=w1764:bool)
                        n1112 = Not Equal?(x=w1756, y=w1758) -> (x != y?=w1759:bool)
                        n1113 = Not Equal To 0?(x=w1766) -> (x != 0?=w1763:bool)
                        n1114 = Not Equal To 0?(x=w1757) -> (x != 0?=w1760:bool)
                        n1115 = And(x=w1764, y=w1763) -> (x .and. y?=w1751:bool)
                        n1116 = And(x=w1759, y=w1760) -> (x .and. y?=w1754:bool)
                        n1117 = And(x=w1751, y=w1754) -> (x .and. y?=w1753:bool)
                        n1118 = Multiply(x=w1770, y=0.5) -> (x*y=w1752:dbl[])
                      }
                      frame False {
                        n1119 = global read "G_rio.vi" "dgps_pos"() -> (w1772:dbl[])
                        n1120 = Index Array(array=w1772, index #1=0 ("index")) -> (element #1=w1778:dbl, element #2=w1777:dbl)  [unwired: 1 in]
                        n1121 = feedback #26(w1778) -> (w1776:dbl)
                        n1122 = feedback-in #26(w1778) -> ()
                        n1123 = Not Equal?(x=w1778, y=w1776) -> (x != y?=w1775:bool)
                        n1124 = Not Equal To 0?(x=w1777) -> (x != 0?=w1774:bool)
                        n1125 = And(x=w1775, y=w1774) -> (x .and. y?=w1771:bool)
                      }
                    }
                    n1126 = case shown="False" "ublox" {
                      tunnel: [w1660 w1717] -> w1649
                      tunnel: [w1678 w1718] -> w1653
                      frame True {
                        n1127 = global read "G_rio.vi" "gps_vel 1"() -> (w1705:dbl[])
                        n1128 = global read "G_rio.vi" "gps_vel 2"() -> (w1684:dbl[])
                        n1129 = Index Array(array=w1705, index #1=0 ("index"), index #2=1 ("index"), index #3=4 ("index"), index #4=2 ("index")) -> (element #1=w1696:dbl, element #2=w1701:dbl, element #3=w1698:dbl, element #4=w1668:dbl)
                        n1130 = Index Array(array=w1684, index #1=0 ("index"), index #2=1 ("index"), index #3=4 ("index"), index #4=2 ("index")) -> (element #1=w1693:dbl, element #2=w1688:dbl, element #3=w1691:dbl, element #4=w1667:dbl)
                        n1131 = global read "G_rio.vi" "VS_CAN"() -> (w1663:dbl)
                        n1132 = Add(x=w1668, y=w1667) -> (x+y=w1666:dbl)
                        n1133 = Not Equal To 0?(x=w1688) -> (x != 0?=w1689:bool)
                        n1134 = call "angleconv.vi"("deg"=w1698) -> ("rad"=w1681:dbl)  [unwired: 9 in, 1 out]
                        n1135 = call "angleconv.vi"("deg"=w1691) -> ("rad"=w1680:dbl)  [unwired: 9 in, 1 out]
                        n1136 = feedback #27(0.0 ("Real Matrix Element")) -> (w1695:dbl)
                        n1137 = feedback-in #27(w1696) -> ()
                        n1138 = feedback #28(0.0 ("Real Matrix Element")) -> (w1694:dbl)
                        n1139 = feedback-in #28(w1693) -> ()
                        n1140 = Not Equal?(x=w1696, y=w1695) -> (x != y?=w1702:bool)
                        n1141 = Not Equal?(x=w1693, y=w1694) -> (x != y?=w1687:bool)
                        n1142 = call "headingweightsum.vi"("a"=0.5, "h1"=w1680, "h2"=w1681) -> ("a*h2+(1-a)*h1"=w1678:dbl)  [unwired: 8 in]
                        n1143 = Absolute Value(x=w1663) -> (abs(x)=w1675:dbl)
                        n1144 = Not Equal To 0?(x=w1701) -> (x != 0?=w1700:bool)
                        n1145 = Multiply(x=w1666, y=0.5) -> (x*y=w1676:dbl)
                        n1146 = And(x=w1702, y=w1700) -> (x .and. y?=w1683:bool)
                        n1147 = And(x=w1687, y=w1689) -> (x .and. y?=w1682:bool)
                        n1148 = Divide(x=w1676, y=w1675) -> (x/y=w1677:dbl)
                        n1149 = And(x=w1683, y=w1682) -> (x .and. y?=w1660:bool)
                        n1150 = Decrement(x=w1677) -> (x-1=w1672:dbl)
                        n1151 = Absolute Value(x=w1672) -> (abs(x)=w1673:dbl)
                        n1152 = Greater?(x=w1663, y=15.0) -> (0:w1661:bool)
                        n1153 = Less?(x=w1673, y=0.05) -> (x < y?=w1665:bool)
                        n1154 = Compound Arithmetic op=AND(w1661, w1665, w1660) -> (w1664:bool)
                        n1155 = case shown="True" w1664 {
                          tunnel: w1677 -> [_ w1713]
                          frame False {
                          }
                          frame True {
                            w1707 = u64 18446744073709551615
                            n1156 = local read "vcount"() -> (w1710:u64)
                            n1157 = local read "vgain"() -> (w1715:dbl)
                            n1158 = Increment(x=w1710) -> (x+1=w1709:u64)
                            n1159 = Multiply(x=w1715, y=w1710) -> (x*y=w1714:dbl)
                            n1160 = Not Equal?(x=w1710, y=w1707) -> (x != y?=w1708:bool)
                            n1161 = Add(x=w1713, y=w1714) -> (x+y=w1712:dbl)
                            n1162 = Select(t=w1709, s=w1708, f=w1707) -> (s? t:f=w1706:u64)
                            n1163 = local write "vcount"(w1706) -> ()
                            n1164 = Divide(x=w1712, y=w1706) -> (x/y=w1711:dbl)
                            n1165 = local write "vgain"(w1711) -> ()
                          }
                        }
                      }
                      frame False {
                        n1166 = global read "G_rio.vi" "dgps_vel"() -> (w1740:dbl[])
                        n1167 = global read "G_rio.vi" "VS_CAN"() -> (w1721:dbl)
                        n1168 = Index Array(array=w1740, index #1=0 ("index"), index #2=1 ("index"), index #3=4 ("index"), index #4=2 ("index")) -> (element #1=w1731:dbl, element #2=w1736:dbl, element #3=w1733:dbl, element #4=w1716:dbl)
                        n1169 = Absolute Value(x=w1721) -> (abs(x)=w1728:dbl)
                        n1170 = Divide(x=w1716, y=w1728) -> (x/y=w1729:dbl)
                        n1171 = feedback #29(0.0 ("Real Matrix Element")) -> (w1730:dbl)
                        n1172 = feedback-in #29(w1731) -> ()
                        n1173 = Not Equal?(x=w1731, y=w1730) -> (x != y?=w1737:bool)
                        n1174 = Decrement(x=w1729) -> (x-1=w1725:dbl)
                        n1175 = Not Equal To 0?(x=w1736) -> (x != 0?=w1735:bool)
                        n1176 = And(x=w1737, y=w1735) -> (x .and. y?=w1717:bool)
                        n1177 = Absolute Value(x=w1725) -> (abs(x)=w1726:dbl)
                        n1178 = Greater?(x=w1721, y=15.0) -> (0:w1719:bool)
                        n1179 = Less?(x=w1726, y=0.05) -> (x < y?=w1723:bool)
                        n1180 = Compound Arithmetic op=AND(w1719, w1723, w1717) -> (w1722:bool)
                        n1181 = case shown="True" w1722 {
                          tunnel: w1729 -> [_ w1748]
                          frame False {
                          }
                          frame True {
                            w1742 = u64 18446744073709551615
                            n1182 = local read "vcount"() -> (w1745:u64)
                            n1183 = local read "vgain"() -> (w1750:dbl)
                            n1184 = Increment(x=w1745) -> (x+1=w1744:u64)
                            n1185 = Multiply(x=w1750, y=w1745) -> (x*y=w1749:dbl)
                            n1186 = Not Equal?(x=w1745, y=w1742) -> (x != y?=w1743:bool)
                            n1187 = Add(x=w1748, y=w1749) -> (x+y=w1747:dbl)
                            n1188 = Select(t=w1744, s=w1743, f=w1742) -> (s? t:f=w1741:u64)
                            n1189 = local write "vcount"(w1741) -> ()
                            n1190 = Divide(x=w1747, y=w1741) -> (x/y=w1746:dbl)
                            n1191 = local write "vgain"(w1746) -> ()
                          }
                        }
                        n1192 = call "angleconv.vi"("deg"=w1733) -> ("rad"=w1718:dbl)  [unwired: 9 in, 1 out]
                      }
                    }
                    n1193 = local write "pos_gps"(w1650) -> ()
                    n1194 = local write "get position"(w1648) -> ()
                    n1195 = global read "G_rio.vi" "VS_CAN"() -> (w1654:dbl)
                    n1196 = Greater Or Equal To 0?(x=w1654) -> (x >= 0?=w1655:bool)
                    n1197 = Select(t=0.0, s=w1655, f=3.141592653589793) -> (s? t:f=w1652:dbl)
                    n1198 = local write "get heading"(w1649) -> ()
                    n1199 = call "headingoperater.vi"("h1"=w1652, "h2"=w1653) -> ("h2-h1"=w1651:dbl)  [unwired: 8 in, 1 out]
                    n1200 = local write "h_gps"(w1651) -> ()
                  }
                  frame #1 {
                    n1201 = local read "dt"() -> (w1780:dbl)
                    n1202 = Greater Than 0?(x=w1780) -> (x > 0?=w1779:bool)
                    n1203 = case shown="True" w1779 {
                      tunnel: w1782 -> [w1783 w1786]
                      tunnel: [w1783 w1785] -> w1781
                      frame False {
                      }
                      frame True {
                        n1204 = flat-sequence {
                          tunnel: w1786 -> [w1820]
                          tunnel: [w1798] -> w1784
                          tunnel: [w1849] -> w1785
                          tunnel: w1784 -> [w1848]
                          frame #0 {
                            n1205 = global read "G_rio.vi" "VS_CAN"() -> (w1788:dbl)
                            n1206 = Equal To 0?(x=w1788) -> (x = 0?=w1789:bool)
                            n1207 = case shown="True" w1789 {
                              tunnel: [w1821 _] -> w1787
                              frame False {
                                n1208 = global read "G_rio.vi" "yaw_rate"() -> (w1824:dbl)
                                n1209 = local read "hbias"() -> (w1825:dbl)
                                n1210 = Subtract(x=w1824, y=w1825) -> (x-y=w1822:dbl)
                                n1211 = Negate(x=w1822) -> (-x=w1823:dbl)
                                n1212 = call "angleconv.vi"("deg"=w1823) -> ("rad"=w1821:dbl)  [unwired: 9 in, 1 out]
                              }
                              frame True {
                                n1213 = disable-structure shown="Enabled" {
                                disable-tunnel: [w1828 _] -> w1826
                                frame Enabled {
                                w1830 = u64 18446744073709551615
                                n1214 = local read "hcount"() -> (w1833:u64)
                                n1215 = local read "hbias"() -> (w1836:dbl)
                                n1216 = Not Equal?(x=w1833, y=w1830) -> (x != y?=w1831:bool)
                                n1217 = Increment(x=w1833) -> (x+1=w1832:u64)
                                n1218 = global read "G_rio.vi" "yaw_rate"() -> (w1827:dbl)
                                n1219 = Multiply(x=w1836, y=w1833) -> (x*y=w1835:dbl)
                                n1220 = Select(t=w1832, s=w1831, f=w1830) -> (s? t:f=w1829:u64)
                                n1221 = local write "hcount"(w1829) -> ()
                                n1222 = Add(x=w1827, y=w1835) -> (x+y=w1834:dbl)
                                n1223 = Divide(x=w1834, y=w1829) -> (x/y=w1828:dbl)
                                }
                                frame Disabled {
                                }
                                }
                                n1224 = local write "hbias"(w1826) -> ()
                              }
                            }
                            n1225 = global read "G_rio.vi" "VS_CAN"() -> (w1792:dbl)
                            n1226 = local read "vgain"() -> (w1793:dbl)
                            n1227 = Multiply(x=w1792, y=w1793) -> (x*y=w1791:dbl)
                            n1228 = Divide(x=w1791, y=3.6) -> (x/y=w1790:dbl)
                            n1229 = Index Array(array=w1820, index #1=0 ("index"), index #2=3 ("index"), index #3=1 ("index"), index #4=3 ("index")) -> (element #1=w1814:dbl, element #2=w1812:dbl, element #3=w1808:dbl, element #4=w1803:dbl)
                            n1230 = local read "dt"() -> (w1817:dbl)
                            n1231 = local read "dt"() -> (w1801:dbl)
                            n1232 = Multiply(x=w1790, y=w1817) -> (x*y=w1813:dbl)
                            n1233 = Multiply(x=w1801, y=w1787) -> (x*y=w1794:dbl)
                            n1234 = Cosine(x=w1812) -> (cos(x)=w1818:dbl)
                            n1235 = Sine(x=w1812) -> (sin(x)=w1811:dbl)
                            n1236 = local write "rt"(w1794) -> ()
                            n1237 = Multiply(x=w1818, y=w1813) -> (x*y=w1815:dbl)
                            n1238 = Multiply(x=w1813, y=w1811) -> (x*y=w1810:dbl)
                            n1239 = Add(x=w1814, y=w1815) -> (x+y=w1807:dbl)
                            n1240 = Add(x=w1810, y=w1808) -> (x+y=w1806:dbl)
                            n1241 = call "headingoperater.vi"("h1"=w1794, "h2"=w1803) -> ("h2+h1"=w1802:dbl)  [unwired: 8 in, 1 out]
                            n1242 = Build Array(w1807, w1806, w1790, w1802, w1787) -> (w1798:dbl[])
                            n1243 = Index Array(array=w1798, index=3) -> (element=w1797:dbl)
                            n1244 = local read "h_gps"() -> (w1796:dbl)
                            n1245 = call "headingoperater.vi"("h1"=w1797, "h2"=w1796) -> ("h2-h1"=w1800:dbl)  [unwired: 8 in, 1 out]
                            n1246 = Absolute Value(x=w1800) -> (abs(x)=w1795:dbl)
                            n1247 = local write "heading error"(w1795) -> ()
                          }
                          frame #1 {
                            n1248 = local read "get heading"() -> (w1856:bool)
                            n1249 = local read "get position"() -> (w1855:bool)
                            n1250 = local read "POS init"() -> (w1841:bool)
                            n1251 = case shown="True" w1841 {
                              tunnel: w1856 -> [w1859 w1866]
                              tunnel: w1855 -> [w1863 w1865]
                              tunnel: [w1857 w1864] -> w1851
                              frame False {
                                n1252 = local read "heading error"() -> (w1860:dbl)
                                n1253 = Less?(x=w1860, y=0.05) -> (x < y?=w1861:bool)
                                n1254 = And(x=w1859, y=w1861) -> (x .and. y?=w1858:bool)
                                n1255 = Or(x=w1858, y=w1863) -> (x .or. y?=w1857:bool)
                              }
                              frame True {
                                n1256 = disable-structure shown="Enabled" {
                                disable-tunnel: w1866 -> [w1869 w1871]
                                disable-tunnel: w1865 -> [w1868 w1870]
                                disable-tunnel: [w1867 w1872] -> w1864
                                frame Disabled {
                                n1257 = And(x=w1869, y=w1868) -> (x .and. y?=w1867:bool)
                                }
                                frame Enabled {
                                n1258 = Or(x=w1871, y=w1870) -> (x .or. y?=w1872:bool)
                                }
                                }
                              }
                            }
                            n1259 = global read "G_rio.vi" "VS_CAN"() -> (w1854:dbl)
                            n1260 = local read "heading error"() -> (w1844:dbl)
                            n1261 = Absolute Value(x=w1854) -> (abs(x)=w1853:dbl)
                            n1262 = local read "POS init"() -> (w1842:bool)
                            n1263 = Greater?(x=w1853, y=5.0) -> (0:w1850:bool)
                            n1264 = Less?(x=w1844, y=1.0) -> (x < y?=w1843:bool)
                            n1265 = Or(x=w1843, y=w1842) -> (x .or. y?=w1845:bool)
                            n1266 = And(x=w1851, y=w1850) -> (x .and. y?=w1846:bool)
                            n1267 = And(x=w1846, y=w1845) -> (x .and. y?=w1839:bool)
                            n1268 = Select(t=FALSE, s="GPS init", f=w1839) -> (s? t:f=w1838:bool)
                            n1269 = case shown="True" w1838 {
                              tunnel: [w1876 w1905] -> w1849
                              tunnel: w1848 -> [w1877 w1908]
                              frame False {
                                n1270 = global read "G_rio.vi" "VS_CAN"() -> (w1880:dbl)
                                n1271 = local read "POS init"() -> (w1879:bool)
                                n1272 = Equal To 0?(x=w1880) -> (x = 0?=w1878:bool)
                                n1273 = local read "GPS init"() -> (w1873:bool)
                                n1274 = And(x=w1879, y=w1878) -> (x .and. y?=w1875:bool)
                                n1275 = Or(x=w1875, y=w1873) -> (x .or. y?=w1874:bool)
                                n1276 = case shown="True" w1874 {
                                tunnel: w1877 -> [w1881 w1882]
                                tunnel: [w1881 w1884] -> w1876
                                tunnel: w1873 -> [_ w1883]
                                frame False {
                                }
                                frame True {
                                n1277 = case shown="True" w1883 {
                                tunnel: [w1895 w1904] -> w1884
                                tunnel: w1882 -> [w1890 w1898]
                                frame True {
                                n1278 = Index Array(array=w1890, index #1=2 ("index")) -> (element #2=w1885:dbl, element #3=w1888:dbl)  [unwired: 2 in, 1 out]
                                n1279 = local read "pos_gps"() -> (w1891:dbl[])
                                n1280 = local write "GPS init"(FALSE ("GPS init")) -> ()
                                n1281 = Index Array(array=w1891, index #1=2 ("index")) -> (element #1=w1893:dbl, element #2=w1892:dbl)  [unwired: 1 in]
                                n1282 = local read "h_gps"() -> (w1886:dbl)
                                n1283 = Build Array(w1893, w1892, w1885, w1886, w1888) -> (w1895:dbl[])
                                }
                                frame False {
                                w1897 = 0.0 ("element")
                                n1284 = Index Array(array=w1898, index=3) -> (element=w1896:dbl)
                                n1285 = local read "pos_gps"() -> (w1900:dbl[])
                                n1286 = Index Array(array=w1900, index #1=2 ("index")) -> (element #1=w1902:dbl, element #2=w1901:dbl)  [unwired: 1 in]
                                n1287 = Build Array(w1902, w1901, w1897, w1896, w1897) -> (w1904:dbl[])
                                }
                                }
                                }
                                }
                              }
                              frame True {
                                n1288 = flat-sequence {
                                tunnel: w1908 -> [w1909]
                                tunnel: [w1909] -> w1907
                                tunnel: w1907 -> [w1950]
                                tunnel: [w1950] -> w1906
                                tunnel: w1906 -> [w1977]
                                tunnel: [w1981] -> w1905
                                frame #0 {
                                w1918 = 0.0 ("element")
                                w1922 = 0.0 ("element")
                                w1924 = 0.0 ("element")
                                w1926 = 0.0 ("element")
                                w1928 = 0.0 ("element")
                                n1289 = Index Array(array=w1909, index #1=3 ("index"), index #2=2 ("index"), index #3=3 ("index"), index #4=2 ("index")) -> (element #1=w1938:dbl, element #2=w1940:dbl, element #3=w1943:dbl, element #4=w1932:dbl)
                                n1290 = Negate(x=w1940) -> (-x=w1939:dbl)
                                n1291 = Sine & Cosine(0:w1943) -> (1:w1935:dbl, 2:w1933:dbl)
                                n1292 = Multiply(x=w1939, y=w1935) -> (x*y=w1936:dbl)
                                n1293 = Multiply(x=w1933, y=w1932) -> (x*y=w1931:dbl)
                                n1294 = Cosine(x=w1938) -> (cos(x)=w1937:dbl)
                                n1295 = Build Array(w1928, w1928, w1937, w1936, 0.0 ("element")) -> (w1930:dbl[])
                                n1296 = Build Array(w1926, w1926, w1935, w1931, 0.0 ("element")) -> (w1929:dbl[])
                                n1297 = Build Array(w1924, w1924, w1924, w1924, w1924) -> (w1923:dbl[])
                                n1298 = Build Array(w1922, w1922, w1922, w1922, 1.0 ("element")) -> (w1920:dbl[])
                                n1299 = Build Array(w1918, w1918, w1918, w1918, w1918) -> (w1919:dbl[])
                                n1300 = Build Array(w1930, w1929, w1923, w1920, w1919) -> (w1916:dbl[][])
                                n1301 = call-poly <vilib>:"Array To Matrix.vi"("Real 2D Array"=w1916) -> ("Real Matrix"=w1914:T10)
                                n1302 = global read "G_rio.vi" "P"() -> (w1917:T10)
                                n1303 = Transpose Matrix(1:w1914) -> (0:w1913:T10)
                                n1304 = call-poly <vilib>:"Multiply.vi"("Real Matrix B"=w1917, "Real Matrix A"=w1914) -> ("A * B"=w1915:T10)
                                n1305 = call-poly <vilib>:"Multiply.vi"("Real Matrix B"=w1913, "Real Matrix A"=w1915) -> ("A * B"=w1912:T10)
                                n1306 = global read "G_rio.vi" "Q"() -> (w1911:T10)
                                n1307 = call-poly <vilib>:"Add.vi"("Real Matrix B"=w1911, "Real Matrix A"=w1912) -> ("A + B"=w1910:T10)
                                n1308 = global write "G_rio.vi" "Pp"(w1910) -> ()
                                }
                                frame #1 {
                                n1309 = global read "G_rio.vi" "Pp"() -> (w1975:T10)
                                n1310 = global read "G_rio.vi" "H"() -> (w1974:T10)
                                n1311 = Array Subset(array=w1950, index=0, length=2) -> (w1957:dbl[])
                                n1312 = local read "pos_gps"() -> (w1953:dbl[])
                                n1313 = call-poly <vilib>:"Multiply.vi"("Real Matrix B"=w1975, "Real Matrix A"=w1974) -> ("A * B"=w1973:T10)
                                n1314 = Transpose Matrix(1:w1974) -> (0:w1972:T10)
                                n1315 = call-poly <vilib>:"Multiply.vi"("Real Matrix B"=w1972, "Real Matrix A"=w1973) -> ("A * B"=w1971:T10)
                                n1316 = Array Subset(array=w1953, index=2, length=2) -> (w1956:dbl[])
                                n1317 = Subtract(x=w1956, y=w1957) -> (x-y=w1958:dbl[])
                                n1318 = global read "G_rio.vi" "H"() -> (w1969:T10)
                                n1319 = global read "G_rio.vi" "R"() -> (w1970:T10)
                                n1320 = global read "G_rio.vi" "Pp"() -> (w1968:T10)
                                n1321 = call-poly <vilib>:"Add.vi"("Real Matrix B"=w1970, "Real Matrix A"=w1971) -> ("A + B"=w1965:T10)
                                n1322 = Square(x=w1958) -> (x^2=w1959:dbl[])
                                n1323 = Transpose Matrix(1:w1969) -> (0:w1967:T10)
                                n1324 = local read "heading error"() -> (w1962:dbl)
                                n1325 = call-poly <vilib>:"Multiply.vi"("Real Matrix B"=w1967, "Real Matrix A"=w1968) -> ("A * B"=w1966:T10)
                                n1326 = Add Array Elements(numeric array=w1959) -> (sum=w1960:dbl)
                                n1327 = call-poly <vilib>:"Inverse Matrix.vi"("Input Matrix"=w1965) -> ("Inverse Matrix"=w1964:T10)  [unwired: 1 in, 1 out]
                                n1328 = call-poly <vilib>:"Multiply.vi"("Real Matrix B"=w1964, "Real Matrix A"=w1966) -> ("A * B"=w1963:T10)
                                n1329 = Square Root(x=w1960) -> (sqrt(x)=w1949:dbl)
                                n1330 = global write "G_rio.vi" "K"(w1963) -> ()
                                n1331 = Less?(x=w1949, y=2.5) -> (x < y?=w1946:bool)
                                n1332 = Less?(x=w1962, y=0.05) -> (x < y?=w1947:bool)
                                n1333 = And(x=w1947, y=w1946) -> (x .and. y?=w1945:bool)
                                n1334 = case shown="True" w1945 {
                                frame False {
                                }
                                frame True {
                                n1335 = local write "POS init"(FALSE ("Kalman init")) -> ()
                                }
                                }
                                }
                                frame #2 {
                                n1336 = disable-structure shown="Enabled" {
                                disable-tunnel: [w1999 w2001] -> w1979
                                disable-tunnel: w1977 -> [_ w2010]
                                frame Disabled {
                                n1337 = local read "get position"() -> (w1999:bool)
                                }
                                frame Enabled {
                                n1338 = Array Subset(array=w2010, index=0, length=2) -> (w2008:dbl[])
                                n1339 = local read "pos_gps"() -> (w2013:dbl[])
                                n1340 = Array Subset(array=w2013, index=2, length=2) -> (w2009:dbl[])
                                n1341 = disable-structure shown="Enabled" {
                                disable-tunnel: [w2016 TRUE ("Kalman init")] -> w2003
                                frame Disabled {
                                n1342 = local read "POS init"() -> (w2016:bool)
                                }
                                frame Enabled {
                                }
                                }
                                n1343 = Subtract(x=w2009, y=w2008) -> (x-y=w2007:dbl[])
                                n1344 = Square(x=w2007) -> (x^2=w2006:dbl[])
                                n1345 = Add Array Elements(numeric array=w2006) -> (sum=w2005:dbl)
                                n1346 = Square Root(x=w2005) -> (sqrt(x)=w2000:dbl)
                                n1347 = local write "pos error"(w2000) -> ()
                                n1348 = Less?(x=w2000, y=3.0) -> (x < y?=w2002:bool)
                                n1349 = Or(x=w2003, y=w2002) -> (x .or. y?=w2001:bool)
                                }
                                }
                                n1350 = disable-structure shown="Enabled" {
                                disable-tunnel: [w1993 w1994] -> w1980
                                frame Disabled {
                                n1351 = local read "get heading"() -> (w1993:bool)
                                }
                                frame Enabled {
                                n1352 = local read "heading error"() -> (w1997:dbl)
                                n1353 = local read "POS init"() -> (w1995:bool)
                                n1354 = Less?(x=w1997, y=0.1) -> (x < y?=w1996:bool)
                                n1355 = Or(x=w1996, y=w1995) -> (x .or. y?=w1994:bool)
                                }
                                }
                                n1356 = Index Array(array=w1977, index=3) -> (element=w1984:dbl)
                                n1357 = global read "G_rio.vi" "K"() -> (w1992:T10)
                                n1358 = global read "G_rio.vi" "H"() -> (w1991:T10)
                                n1359 = global read "G_rio.vi" "Pp"() -> (w1989:T10)
                                n1360 = call-poly <vilib>:"Multiply.vi"("Real Matrix B"=w1991, "Real Matrix A"=w1992) -> ("A * B"=w1990:T10)
                                n1361 = global read "G_rio.vi" "Pp"() -> (w1987:T10)
                                n1362 = call-poly <vilib>:"Multiply.vi"("Real Matrix B"=w1989, "Real Matrix A"=w1990) -> ("A * B"=w1988:T10)
                                n1363 = call-poly <vilib>:"Subtract.vi"("Real Matrix B"=w1988, "Real Matrix A"=w1987) -> ("A - B"=w1986:T10)
                                n1364 = global write "G_rio.vi" "P"(w1986) -> ()
                                n1365 = case shown="True" w1980 {
                                tunnel: w1984 -> [w2042 w2049]
                                tunnel: [w2042 w2044] -> w1978
                                frame False {
                                }
                                frame True {
                                n1366 = global read "G_rio.vi" "K"() -> (w2048:T10)
                                n1367 = Index Array(array=w2048, index (row)=3, index (col)=2 ("disabled index (col)")) -> (element=w2045:dbl)
                                n1368 = local read "h_gps"() -> (w2043:dbl)
                                n1369 = call "headingweightsum2.vi"("a"=w2045, "h2"=w2043, "h1"=w2049) -> ("a*h2+(1-a)*h1"=w2044:dbl)  [unwired: 8 in]
                                }
                                }
                                n1370 = case shown="True" w1979 {
                                tunnel: w1977 -> [w2018 w2030]
                                tunnel: [w2018 w2029] -> w1983
                                tunnel: w1978 -> [_ w2019]
                                frame False {
                                }
                                frame True {
                                n1371 = disable-structure shown="Enabled" {
                                disable-tunnel: [w2040 w2041] -> w2020
                                disable-tunnel: w2019 -> [_ w2041]
                                frame Disabled {
                                n1372 = local read "h_gps"() -> (w2040:dbl)
                                }
                                frame Enabled {
                                }
                                }
                                n1373 = local read "pos_gps"() -> (w2024:dbl[])
                                n1374 = call-poly <vilib>:"Array To Matrix.vi"("Real 1D Array"=w2030) -> ("Real Matrix (Column Vector)"=w2034:T10)
                                n1375 = Array Subset(array=w2024, index=2, length=2) -> (w2025:dbl[])
                                n1376 = Build Array (concatenate)(w2025, w2020) -> (w2021:dbl[])
                                n1377 = global read "G_rio.vi" "H"() -> (w2039:T10)
                                n1378 = call-poly <vilib>:"Multiply.vi"("Real Matrix B"=w2034, "Real Matrix A"=w2039) -> ("A * B"=w2038:T10)
                                n1379 = call-poly <vilib>:"Array To Matrix.vi"("Real 1D Array"=w2021) -> ("Real Matrix (Column Vector)"=w2037:T10)
                                n1380 = call-poly <vilib>:"Subtract.vi"("Real Matrix B"=w2038, "Real Matrix A"=w2037) -> ("A - B"=w2035:T10)
                                n1381 = global read "G_rio.vi" "K"() -> (w2036:T10)
                                n1382 = call-poly <vilib>:"Multiply.vi"("Real Matrix B"=w2035, "Real Matrix A"=w2036) -> ("A * B"=w2028:T10)
                                n1383 = call-poly <vilib>:"Multiply.vi"("Real Matrix A"=w2028, "Real Scalar c"=0.5) -> ("c * A"=w2026:T10)
                                n1384 = call-poly <vilib>:"Add.vi"("Real Matrix B"=w2034, "Real Matrix A"=w2026) -> ("A + B"=w2033:T10)
                                n1385 = call-poly <vilib>:"Matrix To Array.vi"("Real Matrix"=w2033) -> ("Real 2D Array"=w2032:dbl[][])
                                n1386 = Index Array(array=w2032, index (col)=0 ("disabled index (col)")) -> (element=w2029:dbl[])  [unwired: 1 in]
                                }
                                }
                                n1387 = Replace Array Subset(array=w1983, new element=w1978, index=3) -> (w1981:dbl[])
                                }
                                }
                              }
                            }
                          }
                        }
                      }
                    }
                  }
                }
              }
              frame Disabled {
                n1388 = flat-sequence {
                  tunnel: [w2079] -> w2071
                  tunnel: w2072 -> [w2080]
                  tunnel: w2071 -> [w2106]
                  tunnel: [w2105] -> w2070
                  tunnel: [w2104] -> w2068
                  tunnel: [w2103] -> w2067
                  tunnel: w2070 -> [w2201]
                  tunnel: [w2201] -> w2069
                  tunnel: w2068 -> [w2193]
                  tunnel: w2067 -> [w2192]
                  tunnel: w2069 -> [w2214]
                  tunnel: [w2213] -> w2066
                  tunnel: w2066 -> [w2239]
                  tunnel: [w2239] -> w2065
                  tunnel: [w2238] -> w2064
                  tunnel: [w2237] -> w2063
                  tunnel: [w2236] -> w2062
                  tunnel: [w2235] -> w2061
                  tunnel: [w2234] -> w2060
                  tunnel: [w2342] -> w2059
                  tunnel: w2065 -> [w2342]
                  tunnel: w2064 -> [w2335]
                  tunnel: w2063 -> [w2336]
                  tunnel: w2062 -> [w2329]
                  tunnel: w2061 -> [w2328]
                  tunnel: w2060 -> [w2325]
                  frame #0 {
                    n1389 = Index Array(array=w2080, index=3) -> (element=w2085:dbl)
                    n1390 = global read "G_rio.vi" "VS_CAN"() -> (w2076:dbl)
                    n1391 = Equal To 0?(x=w2076) -> (x = 0?=w2075:bool)
                    n1392 = case shown="False" w2075 {
                      tunnel: [w2087 _] -> w2074
                      frame False {
                        n1393 = global read "G_rio.vi" "yaw_rate"() -> (w2090:dbl)
                        n1394 = local read "hbias"() -> (w2091:dbl)
                        n1395 = Subtract(x=w2090, y=w2091) -> (x-y=w2088:dbl)
                        n1396 = Negate(x=w2088) -> (-x=w2089:dbl)
                        n1397 = call "angleconv.vi"("deg"=w2089) -> ("rad"=w2087:dbl)  [unwired: 9 in, 1 out]
                      }
                      frame True {
                        w2095 = u64 18446744073709551615
                        n1398 = local read "hcount"() -> (w2098:u64)
                        n1399 = local read "hbias"() -> (w2101:dbl)
                        n1400 = Increment(x=w2098) -> (x+1=w2097:u64)
                        n1401 = global read "G_rio.vi" "yaw_rate"() -> (w2092:dbl)
                        n1402 = Not Equal?(x=w2098, y=w2095) -> (x != y?=w2096:bool)
                        n1403 = Multiply(x=w2101, y=w2098) -> (x*y=w2100:dbl)
                        n1404 = Add(x=w2092, y=w2100) -> (x+y=w2099:dbl)
                        n1405 = Select(t=w2097, s=w2096, f=w2095) -> (s? t:f=w2094:u64)
                        n1406 = local write "hcount"(w2094) -> ()
                        n1407 = Divide(x=w2099, y=w2094) -> (x/y=w2093:dbl)
                        n1408 = local write "hbias"(w2093) -> ()
                      }
                    }
                    n1409 = local read item#-1() -> (w2078)
                    n1410 = Subtract(x=w2074, y=w2078) -> (x-y=w2084:dbl)
                    n1411 = local read "dt"() -> (w2083:dbl)
                    n1412 = Multiply(x=w2084, y=w2083) -> (x*y=w2073:dbl)
                    n1413 = local write "rt"(w2073) -> ()
                    n1414 = call "headingoperater.vi"("h1"=w2073, "h2"=w2085) -> ("h2+h1"=w2082:dbl)  [unwired: 8 in, 1 out]
                    n1415 = Replace Array Subset(array=w2080, new element #1=w2082, index #1=3 ("index"), new element #2=w2074, index #2=4 ("index")) -> (w2079:dbl[])
                  }
                  frame #1 {
                    n1416 = global read "G_rio.vi" "gps_vel 1"() -> (w2133:dbl[])
                    n1417 = global read "G_rio.vi" "gps_vel 2"() -> (w2122:dbl[])
                    n1418 = global read "G_rio.vi" "VS_CAN"() -> (w2110:dbl)
                    n1419 = Index Array(array=w2133, index #1=1 ("index"), index #2=0 ("index"), index #3=0 ("index")) -> (element #1=w2128:dbl, element #2=w2117:dbl, element #3=w2111:dbl)
                    n1420 = Index Array(array=w2122, index #1=0 ("index"), index #2=1 ("index"), index #3=0 ("index")) -> (element #1=w2113:dbl, element #2=w2127:dbl, element #3=w2116:dbl)
                    n1421 = Equal?(x=w2111, y=w2113) -> (x = y?=w2115:bool)
                    n1422 = Absolute Value(x=w2110) -> (abs(x)=w2109:dbl)
                    n1423 = feedback-in #30(w2117) -> ()
                    n1424 = feedback #30(0.0 ("Real Matrix Element")) -> (w2130:dbl)
                    n1425 = feedback #31(0.0 ("Real Matrix Element")) -> (w2125:dbl)
                    n1426 = feedback-in #31(w2116) -> ()
                    n1427 = Greater?(x=w2117, y=w2130) -> (0:w2120:bool)
                    n1428 = Greater?(x=w2116, y=w2125) -> (0:w2118:bool)
                    n1429 = Not Equal To 0?(x=w2128) -> (x != 0?=w2121:bool)
                    n1430 = Not Equal To 0?(x=w2127) -> (x != 0?=w2119:bool)
                    n1431 = Greater?(x=w2109, y=5.0) -> (0:w2107:bool)
                    n1432 = Compound Arithmetic op=AND(w2107, w2121, w2120, w2115, w2119, w2118) -> (w2102:bool)
                    n1433 = case shown="True" w2102 {
                      tunnel: w2106 -> [w2140 w2166]
                      tunnel: [w2141 w2158] -> w2104
                      tunnel: [w2140 w2166] -> w2105
                      tunnel: [w2139 w2163] -> w2103
                      frame False {
                        n1434 = local read item#-1() -> (w2137)
                        n1435 = Multiply(x=0.9875 ("value"), y=w2137) -> (x*y=w2136:dbl)
                        n1436 = Add(x=0.011 ("value"), y=w2136) -> (x+y=w2134:dbl)
                        n1437 = local read item#-1() -> (w2139)
                        n1438 = Compound Arithmetic op=MULTIPLY(w2134, w2139) -> (w2141:dbl)
                      }
                      frame True {
                        w2165 = 0.001745329251994  # 0.1deg
                        n1439 = Index Array(array=w2166, index=3) -> (element=w2168:dbl)
                        n1440 = global read "G_rio.vi" "gps_vel 1"() -> (w2180:dbl[])
                        n1441 = global read "G_rio.vi" "gps_vel 2"() -> (w2178:dbl[])
                        n1442 = Index Array(array=w2180, index #1=4 ("index"), index #2=2 ("index")) -> (element #1=w2162:dbl, element #2=w2155:dbl)
                        n1443 = Index Array(array=w2178, index #1=4 ("index"), index #2=2 ("index")) -> (element #1=w2160:dbl, element #2=w2154:dbl)
                        n1444 = global read "G_rio.vi" "VS_CAN"() -> (w2147:dbl)
                        n1445 = global read "G_rio.vi" "VS_CAN"() -> (w2172:dbl)
                        n1446 = Add(x=w2155, y=w2154) -> (x+y=w2153:dbl)
                        n1447 = call "angleconv.vi"("deg"=w2162) -> ("rad"=w2161:dbl)  [unwired: 9 in, 1 out]
                        n1448 = call "angleconv.vi"("deg"=w2160) -> ("rad"=w2159:dbl)  [unwired: 9 in, 1 out]
                        n1449 = Absolute Value(x=w2147) -> (abs(x)=w2146:dbl)
                        n1450 = Greater Or Equal To 0?(x=w2172) -> (x >= 0?=w2173:bool)
                        n1451 = Multiply(x=w2153, y=0.5) -> (x*y=w2145:dbl)
                        n1452 = call "headingweightsum.vi"("a"=0.5, "h1"=w2159, "h2"=w2161) -> ("a*h2+(1-a)*h1"=w2171:dbl)  [unwired: 8 in]
                        n1453 = Divide(x=w2145, y=w2146) -> (x/y=w2144:dbl)
                        n1454 = Select(t=0.0, s=w2173, f=3.141592653589793) -> (s? t:f=w2170:dbl)
                        n1455 = Decrement(x=w2144) -> (x-1=w2151:dbl)
                        n1456 = call "headingoperater.vi"("h1"=w2170, "h2"=w2171) -> ("h2-h1"=w2143:dbl)  [unwired: 8 in, 1 out]
                        n1457 = local write "h_gps"(w2143) -> ()
                        n1458 = Absolute Value(x=w2151) -> (abs(x)=w2150:dbl)
                        n1459 = call "headingoperater.vi"("h1"=w2143, "h2"=w2168) -> ("h2-h1"=w2158:dbl)  [unwired: 8 in, 1 out]
                        n1460 = Less?(x=w2150, y=0.05) -> (x < y?=w2148:bool)
                        n1461 = case shown="True" w2148 {
                          tunnel: w2144 -> [_ w2188]
                          frame False {
                          }
                          frame True {
                            w2182 = u64 18446744073709551615
                            n1462 = local read "vcount"() -> (w2185:u64)
                            n1463 = local read "vgain"() -> (w2190:dbl)
                            n1464 = Increment(x=w2185) -> (x+1=w2184:u64)
                            n1465 = Not Equal?(x=w2185, y=w2182) -> (x != y?=w2183:bool)
                            n1466 = Multiply(x=w2190, y=w2185) -> (x*y=w2189:dbl)
                            n1467 = Add(x=w2188, y=w2189) -> (x+y=w2187:dbl)
                            n1468 = Select(t=w2184, s=w2183, f=w2182) -> (s? t:f=w2181:u64)
                            n1469 = Divide(x=w2187, y=w2181) -> (x/y=w2186:dbl)
                            n1470 = local write "vcount"(w2181) -> ()
                            n1471 = local write "vgain"(w2186) -> ()
                          }
                        }
                        n1472 = Absolute Value(x=w2158) -> (abs(x)=w2164:dbl)
                        n1473 = call "angleconv.vi"("rad"=w2158) -> ("deg"=w2142:dbl)  [unwired: 9 in, 1 out]
                        n1474 = Greater?(x=w2165, y=w2164) -> (0:w2167:bool)
                        n1475 = local write "heading error"(w2142) -> ()
                        n1476 = case shown="True" w2167 {
                          frame False {
                          }
                          frame True {
                            n1477 = local write item#-1(0.0 ("initH")) -> ()
                          }
                        }
                        n1478 = local read item#-1() -> (w2163)
                      }
                    }
                    n1479 = local write "get heading"(w2102) -> ()
                  }
                  frame #2 {
                    n1480 = local write item#-1(w2193) -> ()
                    n1481 = Multiply(x=w2193, y="heading gain") -> (x*y=w2200:dbl)
                    n1482 = Negate(x="heading gain") -> (-x=w2197:dbl)
                    n1483 = Multiply(x=w2197, y=w2192) -> (x*y=w2199:dbl)
                    n1484 = feedback #32(0.0) -> (w2194:dbl)
                    n1485 = Compound Arithmetic op=ADD(w2200, w2199, w2194) -> (w2196:dbl)
                    n1486 = local write item#-1(w2196) -> ()
                    n1487 = feedback-in #32(w2196) -> ()
                  }
                  frame #3 {
                    n1488 = global read "G_rio.vi" "VS_CAN"() -> (w2203:dbl)
                    n1489 = Index Array(array=w2214, index #1=1 ("index"), index #2=3 ("index"), index #3=0 ("index")) -> (element #1=w2218:dbl, element #2=w2230:dbl, element #3=w2216:dbl)
                    n1490 = local read "vgain"() -> (w2204:dbl)
                    n1491 = call "headingoperater.vi"("h1"=w2230, "h2"=1.5707963267948966) -> ("h2-h1"=w2229:dbl)  [unwired: 8 in, 1 out]
                    n1492 = Multiply(x=w2203, y=w2204) -> (x*y=w2202:dbl)
                    n1493 = Sine & Cosine(0:w2229) -> (1:w2226:dbl, 2:w2227:dbl)
                    n1494 = Divide(x=w2202, y=3.6) -> (x/y=w2207:dbl)
                    n1495 = Multiply(x=w2226, y=w2207) -> (x*y=w2224:dbl)
                    n1496 = Multiply(x=w2207, y=w2227) -> (x*y=w2225:dbl)
                    n1497 = local read item#-1() -> (w2206)
                    n1498 = local read item#-1() -> (w2205)
                    n1499 = Subtract(x=w2224, y=w2206) -> (x-y=w2223:dbl)
                    n1500 = Subtract(x=w2225, y=w2205) -> (x-y=w2221:dbl)
                    n1501 = local read "dt"() -> (w2222:dbl)
                    n1502 = Multiply(x=w2223, y=w2222) -> (x*y=w2219:dbl)
                    n1503 = Multiply(x=w2222, y=w2221) -> (x*y=w2217:dbl)
                    n1504 = Add(x=w2218, y=w2219) -> (x+y=w2211:dbl)
                    n1505 = Add(x=w2217, y=w2216) -> (x+y=w2209:dbl)
                    n1506 = Replace Array Subset(array=w2214, new element #1=w2211, index #1=1 ("index"), new element #2=w2209, index #2=0 ("index"), new element #3=w2207, index #3=2 ("index")) -> (w2213:dbl[])
                  }
                  frame #4 {
                    n1507 = global read "G_rio.vi" "gps_pos 1"() -> (w2266:dbl[])
                    n1508 = global read "G_rio.vi" "gps_pos 2"() -> (w2255:dbl[])
                    n1509 = global read "G_rio.vi" "VS_CAN"() -> (w2243:dbl)
                    n1510 = Index Array(array=w2266, index #1=1 ("index"), index #2=0 ("index"), index #3=0 ("index")) -> (element #1=w2261:dbl, element #2=w2250:dbl, element #3=w2244:dbl)
                    n1511 = Index Array(array=w2255, index #1=0 ("index"), index #2=1 ("index"), index #3=0 ("index")) -> (element #1=w2246:dbl, element #2=w2260:dbl, element #3=w2249:dbl)
                    n1512 = Equal?(x=w2244, y=w2246) -> (x = y?=w2248:bool)
                    n1513 = Absolute Value(x=w2243) -> (abs(x)=w2242:dbl)
                    n1514 = feedback #33(0.0 ("Real Matrix Element")) -> (w2263:dbl)
                    n1515 = feedback-in #33(w2250) -> ()
                    n1516 = feedback #34(0.0 ("Real Matrix Element")) -> (w2258:dbl)
                    n1517 = feedback-in #34(w2249) -> ()
                    n1518 = Greater?(x=w2250, y=w2263) -> (0:w2253:bool)
                    n1519 = Greater?(x=w2249, y=w2258) -> (0:w2251:bool)
                    n1520 = Not Equal To 0?(x=w2261) -> (x != 0?=w2254:bool)
                    n1521 = Not Equal To 0?(x=w2260) -> (x != 0?=w2252:bool)
                    n1522 = Greater?(x=w2242, y=5.0) -> (0:w2240:bool)
                    n1523 = Compound Arithmetic op=AND(w2240, w2254, w2253, w2248, w2252, w2251) -> (w2233:bool)
                    n1524 = case shown="True" w2233 {
                      tunnel: w2239 -> [_ w2319]
                      tunnel: [w2282 w2300] -> w2238
                      tunnel: [w2283 w2301] -> w2236
                      tunnel: [1.0 w2291] -> w2234
                      tunnel: [w2278 w2303] -> w2237
                      tunnel: [w2277 w2302] -> w2235
                      frame False {
                        n1525 = local read item#-1() -> (w2273)
                        n1526 = local read item#-1() -> (w2276)
                        n1527 = Multiply(x=0.9 ("value"), y=w2273) -> (x*y=w2272:dbl)
                        n1528 = Multiply(x=w2276, y=0.9) -> (x*y=w2269:dbl)
                        n1529 = Add(x=w2272, y=0.01 ("value")) -> (x+y=w2270:dbl)
                        n1530 = Add(x=w2269, y=0.01 ("value")) -> (x+y=w2267:dbl)
                        n1531 = local read item#-1() -> (w2281)
                        n1532 = local read item#-1() -> (w2279)
                        n1533 = Compound Arithmetic op=MULTIPLY(w2270, w2281) -> (w2283:dbl)
                        n1534 = Compound Arithmetic op=MULTIPLY(w2279, w2267) -> (w2282:dbl)
                        n1535 = local read item#-1() -> (w2277)
                        n1536 = local read item#-1() -> (w2278)
                      }
                      frame True {
                        n1537 = global read "G_rio.vi" "gps_pos 1"() -> (w2308:dbl[])
                        n1538 = global read "G_rio.vi" "gps_pos 2"() -> (w2307:dbl[])
                        n1539 = Add(x=w2308, y=w2307) -> (x+y=w2318:dbl[])
                        n1540 = Index Array(array=w2319, index #1=0 ("index"), index #2=1 ("index")) -> (element #1=w2309:dbl, element #2=w2311:dbl)
                        n1541 = Multiply(x=w2318, y=0.5) -> (x*y=w2285:dbl[])
                        "pos_gps" <- w2285
                        n1542 = Index Array(array=w2285, index #1=3 ("index"), index #2=2 ("index"), index #3=9 ("index")) -> (element #1=w2314:dbl, element #2=w2313:dbl, element #3=w2287:dbl)
                        n1543 = Subtract(x=w2311, y=w2313) -> (x-y=w2301:dbl)
                        n1544 = Subtract(x=w2309, y=w2314) -> (x-y=w2300:dbl)
                        n1545 = local read item#-1() -> (w2293)
                        n1546 = Divide(x=0.9, y=w2287) -> (x/y=w2305:dbl)
                        n1547 = Square(x=w2300) -> (x^2=w2296:dbl)
                        n1548 = Square(x=w2301) -> (x^2=w2295:dbl)
                        n1549 = Not Equal To 0?(x=w2293) -> (x != 0?=w2294:bool)
                        n1550 = Max & Min(x=w2305, y=1.0) -> (min(x,y)=w2292:dbl)  [unwired: 1 out]
                        n1551 = Add(x=w2296, y=w2295) -> (x+y=w2286:dbl)
                        n1552 = Select(t=w2293, s=w2294, f=w2292) -> (s? t:f=w2291:dbl)
                        n1553 = local read item#-1() -> (w2298)
                        n1554 = Square Root(x=w2286) -> (sqrt(x)=w2284:dbl)
                        n1555 = Equal To 0?(x=w2298) -> (x = 0?=w2290:bool)
                        n1556 = Less?(x=w2286, y=1.0) -> (x < y?=w2289:bool)
                        n1557 = local write "pos error"(w2284) -> ()
                        n1558 = And(x=w2290, y=w2289) -> (x .and. y?=w2297:bool)
                        n1559 = case shown="True" w2297 {
                          frame False {
                          }
                          frame True {
                            n1560 = local write "POS init"(FALSE ("Kalman init")) -> ()
                            n1561 = local write item#-1(0.0 ("initP")) -> ()
                          }
                        }
                        n1562 = local read item#-1() -> (w2302)
                        n1563 = local read item#-1() -> (w2303)
                      }
                    }
                    n1564 = local write "get position"(w2233) -> ()
                  }
                  frame #5 {
                    n1565 = local write item#-1(w2329) -> ()
                    n1566 = local write item#-1(w2335) -> ()
                    n1567 = Multiply(x=w2329, y="pos gain") -> (x*y=w2332:dbl)
                    n1568 = Multiply(x=w2335, y="pos gain") -> (x*y=w2339:dbl)
                    n1569 = Negate(x="pos gain") -> (-x=w2333:dbl)
                    n1570 = Negate(x="pos gain") -> (-x=w2338:dbl)
                    n1571 = Multiply(x=w2333, y=w2328) -> (x*y=w2334:dbl)
                    n1572 = Multiply(x=w2338, y=w2336) -> (x*y=w2337:dbl)
                    n1573 = feedback #35(0.0) -> (w2330:dbl)
                    n1574 = Compound Arithmetic op=ADD(w2332, w2334, w2330) -> (w2327:dbl)
                    n1575 = feedback-in #35(w2327) -> ()
                    n1576 = feedback #36(0.0) -> (w2341:dbl)
                    n1577 = Compound Arithmetic op=ADD(w2339, w2337, w2341) -> (w2324:dbl)
                    n1578 = feedback-in #36(w2324) -> ()
                    n1579 = Multiply(x=w2327, y=w2325) -> (x*y=w2326:dbl)
                    n1580 = Multiply(x=w2325, y=w2324) -> (x*y=w2323:dbl)
                    n1581 = local write item#-1(w2326) -> ()
                    n1582 = local write item#-1(w2323) -> ()
                  }
                }
                n1583 = Index Array(array=w2059, index #1=1 ("index"), index #2=0 ("index"), index #3=2 ("index")) -> (element #1=w2055:dbl, element #2=w2054:dbl, element #3=w2053:dbl, element #4=w2052:dbl, element #5=w2051:dbl)  [unwired: 2 in]
                n1584 = Build Array(w2055, w2054, w2053, w2052, w2051) -> (w2050:dbl[])
              }
            }
          }
          frame #2 {
            n1585 = flat-sequence {
              tunnel: w2344 -> [w2350]
              frame #0 {
                n1586 = local read "dt"() -> (w2347:dbl)
                n1587 = Array Subset(array=w2350, index=0, length=2) -> (w2358:dbl[])
                "pos" <- w2358
                n1588 = Index Array(array=w2350, index=3) -> (element=w2355:dbl)
                n1589 = Greater Than 0?(x=w2347) -> (x > 0?=w2346:bool)
                n1590 = call "angleconv.vi"("rad"=w2355) -> ("deg"=→"Heading":dbl)  [unwired: 9 in, 1 out]
                n1591 = Greater?(x=1.0, y=w2347) -> (0:w2349:bool)
                n1592 = local read "h_gps"() -> (w2351:dbl)
                n1593 = Compound Arithmetic op=AND(w2349, w2346) -> (w2345:bool)
                n1594 = case shown="True" w2345 {
                  tunnel: w2358 -> [w2368 _]
                  tunnel: w2355 -> [w2364 _]
                  tunnel: w2351 -> [w2363 _]
                  tunnel: w2350 -> [_ w2375]
                  frame False {
                    n1595 = local read "pos_gps"() -> (w2367:dbl[])
                    n1596 = global read "G_rio.vi" "VS_CAN"() -> (w2361:dbl)
                    n1597 = Array Subset(array=w2367, index=5, length=10) -> (w2372:dbl[])
                    n1598 = Array Subset(array=w2367, index=12, length=3) -> (w2369:dbl[])
                    n1599 = local read "map"() -> (w2362:i32)
                    n1600 = local read "dt"() -> (w2366:dbl)
                    n1601 = Build Array (concatenate)(w2372, w2369, w2368, w2366, w2362, w2361, w2364, w2363) -> (w2365:dbl[])
                    n1602 = shared-variable "veloster\\sharedvari.lvlib\\RIONAV"(w2365) -> ()  [unwired: 1 in, 1 out]
                  }
                  frame True {
                    n1603 = flat-sequence {
                      tunnel: w2375 -> [w2399]
                      frame #0 {
                        n1604 = Get Date/Time In Seconds() -> (seconds since 1Jan1904=w2390:timestamp)
                        n1605 = To Double Precision Float(number=w2390) -> (double precision float=w2384:dbl)
                        n1606 = global read "G_rio.vi" "LCM_POS_T"() -> (w2398:T17)
                        n1607 = local read "POS init"() -> (w2380:bool)
                        n1608 = Unbundle By Name(w2398) -> ("hash"=w2395:i64)
                        n1609 = local read "dt"() -> (w2379:dbl)
                        n1610 = Multiply(x=w2384, y=1000000.0) -> (x*y=w2382:dbl)
                        n1611 = Array To Cluster(array=w2399) -> (cluster=w2397:T18)
                        n1612 = Select(t=0.0, s=w2380, f=w2379) -> (s? t:f=w2377:dbl)
                        n1613 = call "hash.vi"("input"=w2395) -> ("output"=w2394:i64)  [unwired: 10 in]
                        n1614 = To Quad Integer(1:w2382) -> (0:w2381:i64)
                        n1615 = Unbundle(w2397) -> ("Real 2D Array[0]"=w2389:dbl, "Real 2D Array[1]"=w2388:dbl, "Real 2D Array[2]"=w2387:dbl, "Real 2D Array[3]"=w2386:dbl, "Real 2D Array[4]"=w2385:dbl)
                        n1616 = Bundle(cluster=w2398, "hash"=w2394, "sys time"=w2381, "dt"=w2377, "x"=w2389, "y"=w2388, "speed"=w2387, "heading"=w2386, "yaw_rate"=w2385) -> (w2376:T17)
                        n1617 = Flatten To String(anything=w2376, prepend array or string size? (T)=FALSE) -> (data string=w2392:string)  [unwired: 2 in, 2 out]
                        n1618 = global read "G_rio.vi" "LCM"() -> (w2391:T3)
                        n1619 = call "LCM_send.vi"("DATA"=w2392, "ID"="POS_T", "LCM"=w2391) -> ()  [unwired: 7 in, 2 out]
                      }
                    }
                  }
                }
                n1620 = call "headingoperater.vi"("h1"=0.0, "h2"=w2351) -> ("h2+h1"=w2352:dbl)  [unwired: 8 in, 1 out]
                n1621 = call "angleconv.vi"("rad"=w2352) -> ("deg"=→"H_GPS":dbl)  [unwired: 9 in, 1 out]
              }
            }
          }
        }
      }
    }
  }
